vi "S4ICS.vi"() -> ()   [LabVIEW 2018]
uses:
  <vilib>/picture/picture.llb/imagedata.ctl
  MotorSim/MotorSim.lvclass
  StateManager/StateManager.lvclass
  Motor/Motor.lvclass
  StateManager/StateManager.lvclass/StateManager.ctl
  Messenger/Messenger.lvclass
  Motor/Motor.lvclass/Motor.ctl
  ICS/ICS.lvclass/ICS.ctl
  TCP-Server/TCP-Server.lvclass/TCP-Server.ctl
  Message Queue/Message Cluster.ctl
  ICS/Global Test.vi
  TCP-Server/TCP-Server.lvclass
  ICS/ICS.lvclass
  Message Queue/Message Queue.lvlib
  MotorManager/MotorManager.lvclass
panel:
  out "version":string caption="vers."
  out "tab body":enum32{"Motors", "Config"}(tab)
  out "commCALW":bool
  out "commGMIR":bool
  out "commASEL":bool
  out "commWPROT":bool
  out "commWPSEL":bool
  out "commGFOC":bool
  out "GFOC home":bool caption="Home"
  out "GFOC limit":bool caption="Limit"
  out "guider cam anime":picture
  out "gmir stat":T1
  out "ASEL Value":dbl
  out "CALW Value":dbl
  out "WPSEL Value":dbl
  out "GMIR Value":dbl
  out "WPROT Value":dbl
  out "GFOC Value":dbl
  out "calw stat":T1
  out "asel stat":T1
  out "wpsel stat":T1
  out "wprot stat":T1
  out "gfoc stat":T1
  out "asel lim on":bool caption="Limit ON"
  out "asel sec ON":bool caption="Sec. ON"
  out "asel lim off":bool caption="Limit OFF"
  out "asel sec off":bool caption="Sec. OFF"
  out "asel anime":picture
  out "asel background":picture
  out "wpsel sec/2":bool caption="Sec. L/4"
  out "wpsel sec/4":bool caption="Sec. L/2"
  out "wp home":bool caption="Home"
  out "wprot ctl":dbl(knob) scale=0.0..360.0
  out "wpsel lim/2":bool caption="Limit L/4"
  out "wpsel lim/4":bool caption="Limit L/2"
  out "wpsel anime":picture
  out "calw2":bool caption="CW 2"
  out "calw1":bool caption="CW 1"
  out "calw0":bool caption="CW 0"
  out "calw knob":cluster{dbl, dbl, dbl, dbl, dbl}(knob)={10.0, 82.0, 154.0, 226.0, 298.0} scale=0.0..360.0
  out "GMIR home":bool caption="Home"
  out "gmir knob":dbl(knob) scale=0.0..360.0
  out "asel image":T2
  in  "tips":T3(array[cluster])=[{"tip name"="login: server off", "PT"="Estado do servidor TCP/IP do S4ICS\npara clientes da rede (e.g. S4GUI).", "EN"="State of the S4ICS TCP/IP server\nfor network clients (e.g. S4GUI)."}, {"tip name"="login: exit", "PT"="Encerra a execução do programa\nS4ICS.", "EN"="Ends the execution of the S4ICS\nprogram."}, {"tip name"="login: language", "PT"="Seleciona a linguagem dos textos\nde ajuda e das dicas ou as ocultam.", "EN"="Select the language of the texts\nof help and tips or hide them."}, {"tip name"="login: user", "PT"="Nome cadastrado do usuário para\npermitir sua identificação.", "EN"="User's registered name to allow\nidentification."}, {"tip name"="login: password", "PT"="Senha cadastrada do usuário\n(digitada no 1o. acesso do usuário).", "EN"="User's registered password\n(entered on user's first login)."}, {"tip name"="login: help", "PT"="Descreve a função dos elementos\nmostrados no painel do S4ICS.", "EN"="Describes the function of elements\nshown on the S4ICS panel."}, {"tip name"="login: login", "PT"="Acesso ao S4ICS com a permissão\nestabelecida pelo administrador.", "EN"="Access to S4ICS according to\npermission set by administrator."}, {"tip name"="stopped: start srv", "PT"="Habilita o servidor TCP/IP do S4ICS\n(faz logout automaticamente).", "EN"="Enables S4ICS TCP/IP server\n(automatically logs out)."}, {"tip name"="stopped: exit", "PT"="Fecha o programa S4ICS.", "EN"="Ends S4ICS program execution."}, {"tip name"="stopped: assist", "PT"="Abre janela para testar e estacionar\nos mecanismos do instrumento.", "EN"="Opens window to test and park\ninstrument mechanisms."}, {"tip name"="stopped: setup", "PT"="Abre a janela de configuração do\ninstrumento (acesso restrito). ", "EN"="Opens the window of instrument\nconfiguration (restricted access)."}, {"tip name"="stopped: control", "PT"="Abre a janela para controlar os\nmecanismos (acesso restrito).", "EN"="Opens the window to control the\nmechanisms (restricted access)."}, {"tip name"="stopped: logout", "PT"="Libera o S4ICS para outro usuário.", "EN"="Release S4ICS for another user."}, {"tip name"="running: stop", "PT"="Desabilita o servidor\nTCP/IP doS4ICS.", "EN"="Disables S4ICS TCP/IP server."}, {"tip name"="running: logout", "PT"="Libera o S4ICS para outro usuário.", "EN"="Release S4ICS for another user."}, {"tip name"="setup: save", "PT"="Salva as alterações mantendo o\nnome do arquivo de  configuração.", "EN"="Save the changes keeping the\nname of the configuration file."}, {"tip name"="setup: save as", "PT"="Salva as alterações em um arquivo\nde  configuração com outro nome.", "EN"="Save changes to a file\nunder another name."}, {"tip name"="setup: help", "PT"="Descreve a função dos elementos\nmostrados no painel abaixo.", "EN"="Describes the function of elements\nshown on below panel."}, {"tip name"="setup: cfg file", "PT"="Nome do arquivo da\nconfiguração atual.\n", "EN"="File name of current configuration."}, {"tip name"="setup: cfg user", "PT"="Nome do usuário que salvou\na configuração atual.", "EN"="Username who saved\nthe current configuration."}, {"tip name"="setup: cfg date", "PT"="Data da configuração atual.", "EN"="Date of current configuration."}, {"tip name"="setup: return", "PT"="Retorna ao menu anterior.", "EN"="Return to previous menu."}, {"tip name"="assist: return", "PT"="Retorna ao menu anterior.", "EN"="Return to previous menu."}, {"tip name"="control: return", "PT"="Retorna ao menu anterior.", "EN"="Return to previous menu."}, {"tip name"="cfg: previous", "PT"="Mostra e seleciona\no usuário anterior.", "EN"="Show and select\nprevious user."}, {"tip name"="cfg: next", "PT"="Mostra e seleciona\no próximo usuário.", "EN"="Show and select\nthe next user."}, {"tip name"="cfg: delete", "PT"="Remove da lista o\nusuário selecionado.", "EN"="Remove from the list\nthe selected user."}, {"tip name"="cfg: name", "PT"="Nome do novo usuário\npara ser inserido na lista.", "EN"="New user name to be\ninserted into the list."}, {"tip name"="cfg: insert", "PT"="Insere na lista o novo usuário com\no nome e a permissão indicados.", "EN"="Insert the new user with the\ngiven name and permission."}, {"tip name"="cfg: permission", "PT"="Permissão do usuário. Restringir\nas atribuições Admin e Control.", "EN"="User permission. Restrict the\nAdmin and Control assignments."}, {"tip name"="cfg: change", "PT"="Atribui a atribuição ao lado\npara o usuário selecionado.", "EN"="Assign left assignment\nfor the selected user."}, {"tip name"="cfg: auto", "PT"="Tempo limite de inatividade para\nlogout automático do usuário.", "EN"="Inactivity timeout to\nautomatic user logout."}, {"tip name"="cfg: enable", "PT"="Permite o envio de e-mails\nde manutenção e configuração.", "EN"="Allows sending maintenance\nand configuration emails."}, {"tip name"="cfg: service", "PT"="Endereço IP e porta do\nservidor de e-mail.", "EN"="IP address and port\nof email server."}, {"tip name"="cfg: admin", "PT"="Endereço de e-mail que receberá\nnotificações de nova configuração.", "EN"="Email address that will receive\nnew configuration notifications."}, {"tip name"="cfg: maint", "PT"="Endereço de email que irá receber\nnotificações de erro e alarme.", "EN"="Email address that will receive\nerror and alarm notifications."}, {"tip name"="cfg: check", "PT"="Envia e-mail e confere recebimento\npara testar o servidor de e-mail.", "EN"="Send emails and check receipt\nto test the email server."}, {"tip name"="cfg: ok", "PT"="Resultado do teste do servidor de\ne-mail. Aguarde alguns segundos.", "EN"="Test result from email server test.\nPlease, wait a few seconds."}, {"tip name"="cfg: srv ip", "PT"="Endereço IP do servidor do S4ICS:\nlocalhost ou IP local (ver abaixo).", "EN"="S4ICS server IP address:\nlocalhost or local IP (see below)."}, {"tip name"="cfg: srv port", "PT"="Porta do servidor do S4ICS que\nserá usada pelos clientes (S4GUI).", "EN"="S4ICS server port used\nby clients (like S4GUI)."}, {"tip name"="cfg: srv timeout", "PT"="Tempo de espera pela conexão:\nmenor tempo exigido pelo servidor do S4ICS.", "EN"="Connection wait time: lower time\nrequired by S4ICS server."}, {"tip name"="cfg: IP1", "PT"="Porta IP ativa (com conexão)\nneste computador.", "EN"="Active IP port (with connection)\non this computer."}, {"tip name"="cfg: IP2", "PT"="Porta IP ativa (com conexão)\nneste computador.", "EN"="Active IP port (with connection)\non this computer."}]
  in  "Enddelay":u32=25
  in  "TX-RXdelay":u32=25
  in  "pubTime0mq":i32=1000 caption="Pub Time*"
  in  "0mqEndpoint":string="5565" caption="PUB Port*"
  in  "address":string="192.168.1.170" caption="Address"
  in  "runMinimized":bool
  in  "autoSS":bool
  in  "log help":bool
  in  "enabled log":string="0123456" caption="LOG Enable"
  in  "WPSEL mode":string(combo)="Control" caption="Mechanism Mode"
  in  "CALW mode":string(combo)="Control" caption="Mechanism Mode"
  in  "GFOC mode":string(combo)="Control" caption="Mechanism Mode"
  in  "animation":bool
  in  "full init":bool
  in  "timeout":i32=100 caption="Timeout"
  in  "port":u16=5564 caption="Port"
  in  "pwrPM mains":bool=TRUE caption="Mains"
  in  "pwrPM password":string="ubnt" caption="Password"
  in  "pwrPM user":string="ubnt" caption="User"
  in  "pwrPM outlet":u16=5 caption="Outlet"
  in  "pwrPM port":u16=6080 caption="Port"
  in  "pwrPM ip":string="192.168.1.20" caption="IP"
  in  "pwrGD mains":bool=TRUE caption="Mains"
  in  "pwrGD password":string="ubnt" caption="Password"
  in  "pwrGD user":string="ubnt" caption="User"
  in  "pwrGD outlet":u16=6 caption="Outlet"
  in  "pwrGD port":u16=6080 caption="Port"
  in  "pwrGD ip":string="192.168.1.20" caption="IP"
  in  "GMIR disabled":bool
  in  "GMIR mode":string(combo)="Control" caption="Mechanism Mode"
  in  "GMIR ip":string="192.168.1.249" caption="ip"
  in  "GFOC positions":cluster{"pos_name":string, "pos_value":dbl}[](array[cluster])=[{"pos_name"="OFFSET", "pos_value"=0.0}] caption="GFOC" {"pos_value" min=-400.0 max=400.0 step=0.1}
  in  "GMIR positions":cluster{"pos_name":string, "pos_value":dbl}[](array[cluster])=[{"pos_name"="OFFSET", "pos_value"=0.0}] caption="GMIR" {"pos_value" min=-10.0 max=110.0 step=0.1}
  in  "WPSEL disabled":bool
  in  "WPROT disabled":bool
  in  "WPSEL ip":string="192.168.1.246" caption="ip"
  in  "WPROT mode":string(combo)="Control" caption="Mechanism Mode"
  in  "WPROT ip":string="192.168.1.245" caption="ip"
  in  "WPSEL positions":cluster{"pos_name":string, "pos_value":dbl}[](array[cluster])=[{"pos_name"="OFFSET", "pos_value"=0.0}, {"pos_name"="L/4", "pos_value"=0.0}, {"pos_name"="OFF", "pos_value"=400000.0}, {"pos_name"="L/2", "pos_value"=800000.0}] caption="WPSEL" {"pos_value" min=-400.0 max=400.0 step=0.1}
  in  "WPROT positions":cluster{"pos_name":string, "pos_value":dbl}[](array[cluster])=[{"pos_name"="OFFSET", "pos_value"=0.0}, {"pos_name"="WP1", "pos_value"=0.0}, {"pos_name"="WP2", "pos_value"=1875.0}, {"pos_name"="WP3", "pos_value"=3750.0}, {"pos_name"="WP4", "pos_value"=5625.0}, {"pos_name"="WP5", "pos_value"=7500.0}, {"pos_name"="WP6", "pos_value"=9375.0}, {"pos_name"="WP7", "pos_value"=11250.0}, {"pos_name"="WP8", "pos_value"=13125.0}, {"pos_name"="WP9", "pos_value"=15000.0}, {"pos_name"="WP10", "pos_value"=16875.0}, {"pos_name"="WP11", "pos_value"=18750.0}, {"pos_name"="WP12", "pos_value"=20625.0}, {"pos_name"="WP13", "pos_value"=22500.0}, {"pos_name"="WP14", "pos_value"=24375.0}, {"pos_name"="WP15", "pos_value"=26250.0}, {"pos_name"="WP16", "pos_value"=28125.0}] caption="WPROT" {"pos_value" min=-10.0 max=110.0 step=0.1}
  in  "CALW disabled":bool
  in  "ASEL disabled":bool
  in  "CALW ip":string="192.168.1.247" caption="ip"
  in  "ASEL mode":string(combo)="Control" caption="Mechanism Mode"
  in  "ASEL ip":string="192.168.1.248" caption="ip"
  in  "CALW positions":cluster{"pos_name":string, "pos_value":dbl}[](array[cluster])=[{"pos_name"="OFFSET", "pos_value"=0.0}, {"pos_name"="OFF", "pos_value"=0.0}, {"pos_name"="POLARIZER", "pos_value"=12000.0}, {"pos_name"="PINHOLE", "pos_value"=24000.0}, {"pos_name"="SHUTTER", "pos_value"=36000.0}, {"pos_name"="DEPOLARIZER", "pos_value"=48000.0}] caption="CALW" {"pos_value" min=-400.0 max=400.0 step=0.1}
  in  "ASEL positions":cluster{"pos_name":string, "pos_value":dbl}[](array[cluster])=[{"pos_name"="OFFSET", "pos_value"=0.0}, {"pos_name"="OFF", "pos_value"=0.0}, {"pos_name"="ON", "pos_value"=4800.0}] caption="ASEL" {"pos_value" min=-10.0 max=110.0 step=0.1}
  in  "S4ICS password":string="se4RFVgy&8"
  in  "S4ICS login":string="s4ics@lna.br"
  in  "S4ICS email":string="s4ics@lna.br" caption="S4ICS account"
  in  "auto logout":u32=200 caption="Auto Logout period" min=30 max=3000
  out "email ok":bool
  in  "check email":bool
  in  "maint. email":string="frodrigues@lna.br" caption="Maintenance"
  in  "admin email":string="nivaldo@lna.br" caption="Configuration"
  in  "email service":string="smtp.gmail.com:587" caption="Server IP:PORT"
  out "user list":T4(array[cluster]) caption="Name                 Permission        PW"
  in  "user delete":bool
  in  "user permission":string(combo)="Start / Stop" caption="Permission"
  in  "change permission":bool
  in  "user insert":bool
  in  "user name":string caption="New User"
  in  "user previous":bool
  in  "user next":bool
  in  "email enable":bool caption="Email service"
  in  "channel":T5(ring)=enum."Inner TCP/IP" caption="Channel"
  out "local IP 1":string
  out "local IP 2":string
  in  "comm help":bool
  out "tab menu":T6(tab)
  in  "login help":bool
  in  "loginPW":string caption="Password"
  in  "loginUser":string caption="User Name"
  in  "login":bool
  out "server":bool
  in  "exitLogin":bool
  in  "language":enum32{"PT", "EN", "NONE"}(radio)=enum."NONE"
  in  "stop server":bool
  in  "logout running":bool
  in  "exitStopped":bool
  in  "logout stopped":bool
  in  "start server":bool
  in  "control":bool
  in  "setup":bool
  in  "assist":bool
  in  "return assist":bool
  in  "save as":bool
  out "last cfg date":string caption="Date"
  out "last cfg user":string caption="User"
  in  "save config":bool
  in  "return setup":bool
  in  "config help":bool
  out "cfgFile":string caption="CONFIG FILE"
  out "control response":string caption="Response"
  in  "control instruction":string caption="Instruction"
  in  "control send":bool
  in  "control jump":bool caption="JUMP"
  in  "control position":dbl caption="Mech. Position"
  in  "return control":bool
  in  "control stop":bool
  in  "control motor sel":T7(radio) caption="Motor"
  # "GFOC - Guiding Focuser"
  # "GMIR - Guiding Mirror"
  # "CALW - Calibration Wheel"
  # "FOCUSER"
  # "CLEAR"
  # "GUIDING"
  # "CAMERA"
  # "POLARIZER"
  # "PINHOLE"
  # "SHUTTER"
  # "PATROL"
  # "MIRROR"
  # "DEPOLARIZER"
  # "WPROT - Waveplate Rotator"
  # "WPSEL - Waveplate Selector"
  # "ASEL - Analyser Selector"
  # "POLARIMETRIC MECHANISMS"
  # "SERVER COMMUNICATION"
  # "USER LIST"
  # "(*) Requires EXIT after SAVE\n      Exigido EXIT depois de SAVE"
  # "SIMULATION"
  # "ANIMATION"
  # "ON"
  # "FAST"
  # "FULL"
  # "OFF"
  # "s"
  # "EMAIL SETTINGS"
  # "GUIDING MECHANISMS"
  # "POWER"
  # "POWER"
  # "GMIR & GFOC"
  # "GFOC motor is driven by the GMIR cotroller."
  # "IDENTIFICATION"
  # "LAST CONFIGURATION"
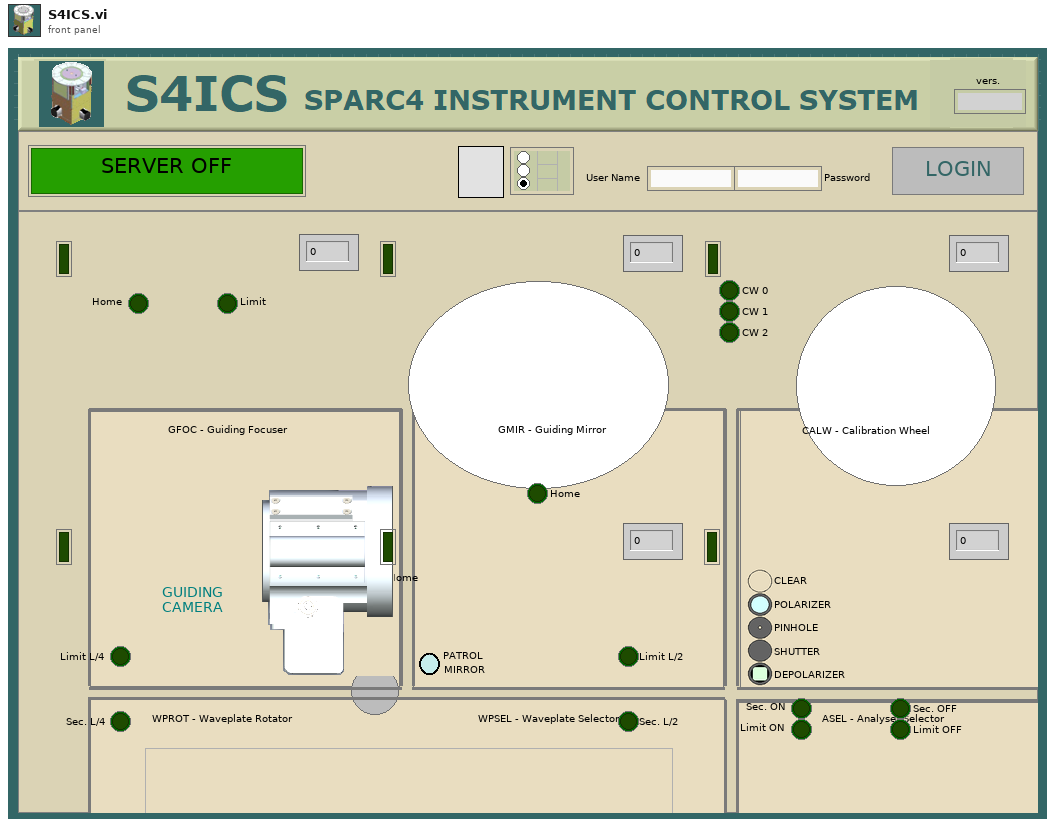
[diagram p1: front panel]
types:
  T1 = cluster{"mode":string, "condition":string, "position":string, "pos_name":string, "pos_id":string}
  T2 = typedef "imagedata.ctl" = cluster{"image type":i32, "image depth":i32, "image":u8[], "mask":u8[], "colors":u32[], "Rectangle":cluster{"left":i16, "top":i16, "right":i16, "bottom":i16}}
  T3 = cluster{"tip name":string, "PT":string, "EN":string}[]
  T4 = cluster{"name":string, "permission":string, "password":string}[]
  T5 = enum32{"Local Panel", "Inner TCP/IP", "Outer TCP/IP", "MQTT", "ZeroMQ"}
  T6 = enum32{"Login", "Running", "Stopped", "Assist", "Setup", "Control"}
  T7 = enum32{"No Selection", "control WPROT", "control WPSEL", "control ASEL", "control CALW", "control GFOC", "control GMIR"}
  T8 = cluster{"S4commandQueueName":string, "S4statusQueueName":string, "comm configuration":cluster{"channel":enum32{"Local Panel", "Inner TCP/IP", "Outer TCP/IP", "MQTT", "ZeroMQ"}, "address":string, "port":u16, "timeout":i32}}
  T9 = enum32{"Motors", "Config", "Status", "Anime", "Param"}
  T10 = cluster{"email service":string, "maint. email":string, "admin email":string, "S4ICS email":string, "S4ICS login":string, "S4ICS password":string, "email enabled":bool}
  T11 = cluster{"period":u32, "initial position (0)":i32, "translation (100)":i32, "forward":bool}[]
  T12 = enum8{"Enabled", "Disabled", "Disabled and Grayed Out"}
  T13 = enum32{"Invalid", "Standard", "Closed", "Hidden", "Minimized", "Maximized"}
  T14 = cluster{"left":i16, "top":i16, "right":i16, "bottom":i16}
  T15 = enum32{"Login", "Stopped", "Running", "Setup", "Assist", "Control"}
  T16 = enum16{"Wait", "ActiveInit", "ActiveGoto", "ActiveUpdate", "ActiveStop", "ActiveFinish", "SimInit", "SimGoto", "SimUptate", "SimFinish", "CyclicStart", "CyclicUpdate", "CyclicFinish"}
  T17 = cluster{"action":string, "param":string, "pos_name":string, "pos_idx":i32, "ack":bool, "stop":bool, "offset":bool, "immediate":bool, "instructions":string[]}
  T18 = typedef "Message Queue.lvlib/Message Cluster.ctl" = cluster{"Message":string, "Message Data":variant}
  T19 = cluster{"channel":enum32{"Local Panel", "Inner TCP/IP", "Outer TCP/IP", "MQTT", "ZeroMQ"}, "address":string, "port":u16, "timeout":i32}
  T20 = cluster{"name":string, "permission":string, "password":string}
  T21 = cluster{"[0]":dbl, "[1]":dbl, "[2]":dbl, "[3]":dbl, "[4]":dbl}
  T22 = enum32{"invalid app kind", "Development System", "Run Time System", "Student Edition", "Embedded LabVIEW", "Evaluation", "Custom"}
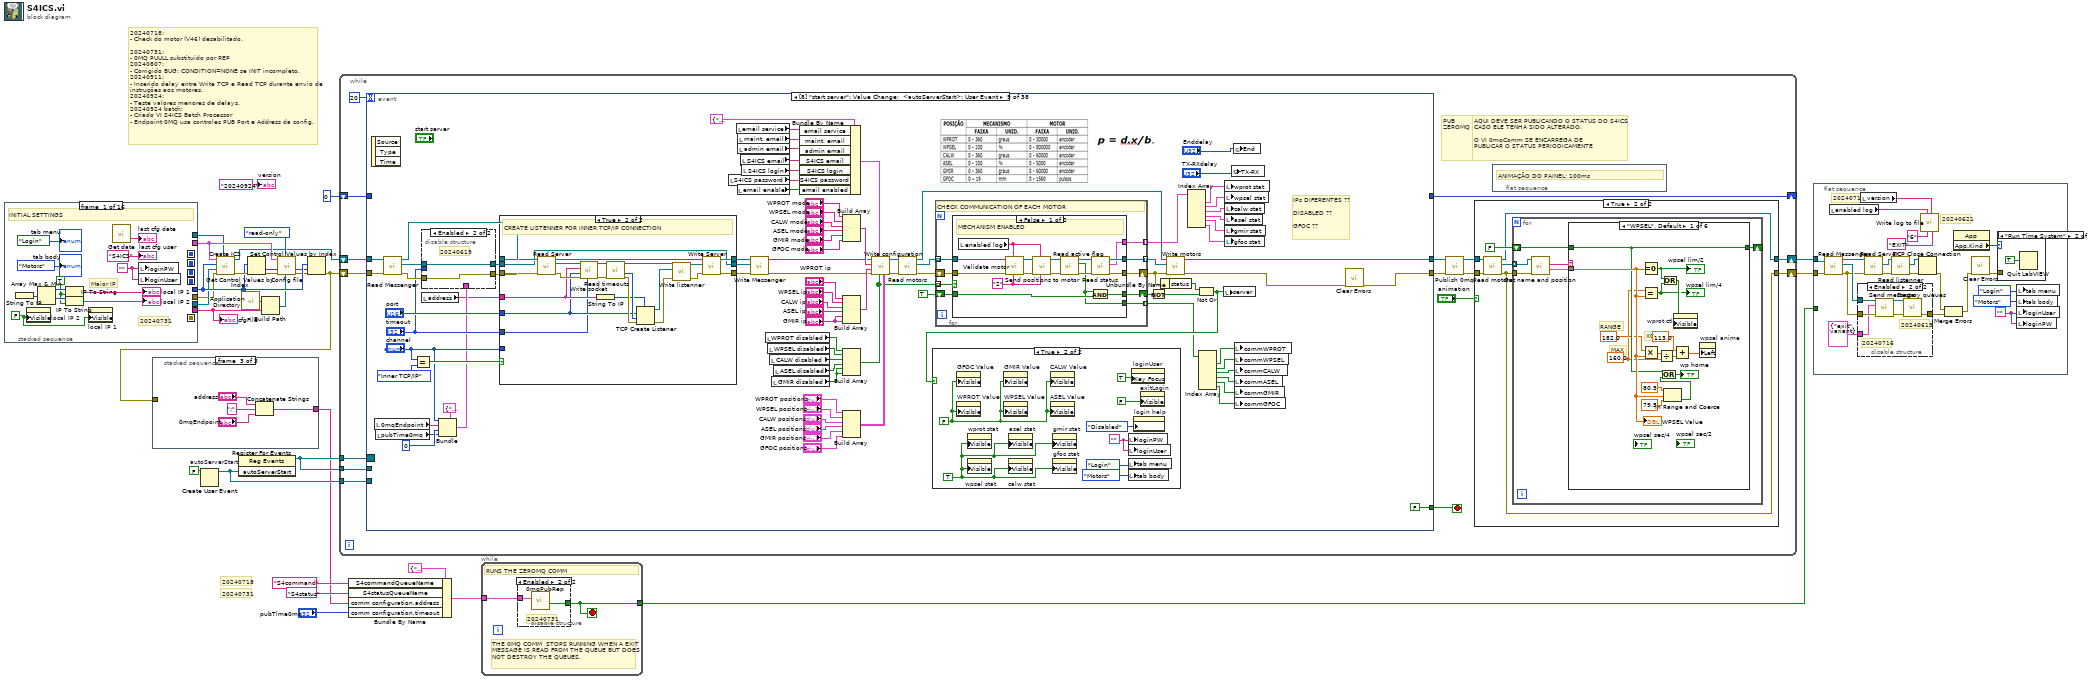
[diagram p0: block diagram]
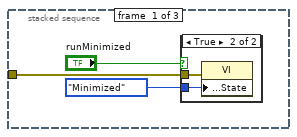
[diagram p2: hidden frame]
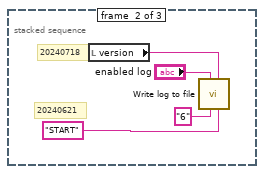
[diagram p4: hidden frame]
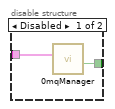
[diagram p5: hidden frame]
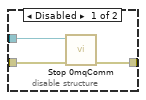
[diagram p6: hidden frame]
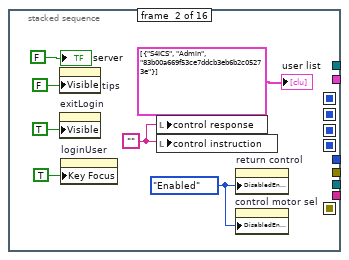
[diagram p8: hidden frame]
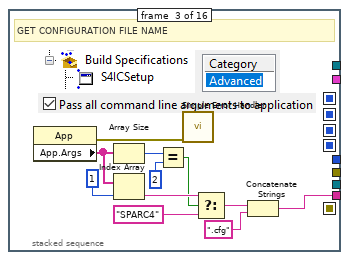
[diagram p9: hidden frame]
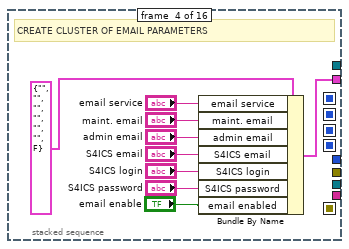
[diagram p10: hidden frame]
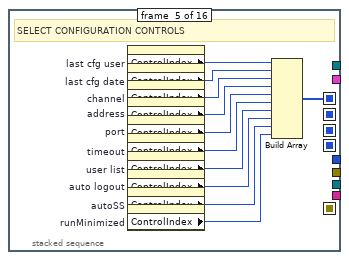
[diagram p11: hidden frame]
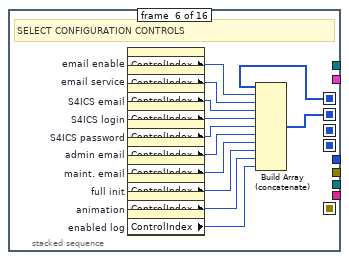
[diagram p12: hidden frame]
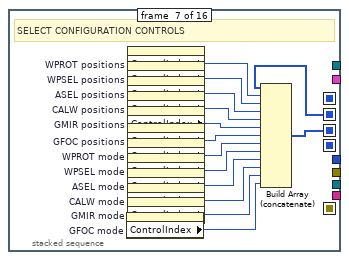
[diagram p13: hidden frame]
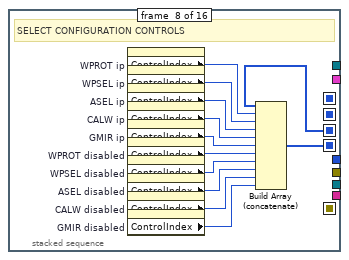
[diagram p14: hidden frame]
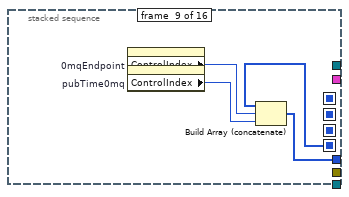
[diagram p15: hidden frame]
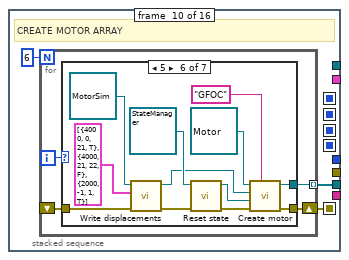
[diagram p16: hidden frame]
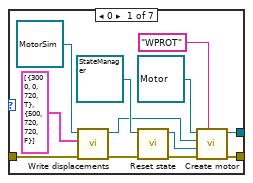
[diagram p17: hidden frame]
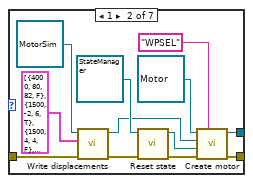
[diagram p18: hidden frame]
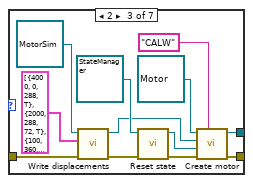
[diagram p19: hidden frame]
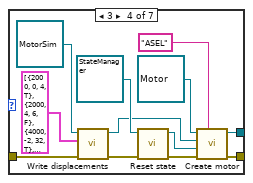
[diagram p20: hidden frame]
diagram:
  w12 = FALSE  # autoServerStart
  # "20240731"
  # "20240718"
  # "20240718:\n- Check do motor (V46) desabilitado.\n\n20240731:\n- 0MQ PUULL substituído por REP\n20240807:\n- Corrigido BUG: CONDITION=NONE se INIT incompleto.\n20240911:\n- Inserido delay entre Write TCP e Read TCP durante envio de instruções aos motores.\n20240924:\n- Teste valores menores de delays.\n20240924 batch:\n- Criado VI S4ICS Batch Processor\n- Endpoint 0MQ usa controles PUB Port e Address da config."
  n1 = stacked-sequence {
    seq-local: [_ _ _ _ w78 _ _ _ _ _ _ _ _ _ _ _] -> [_ _ _ _ _ w92 _ _ _ _ _ _ _ _ _ _]
    seq-local: [_ _ _ _ _ w84 _ _ _ _ _ _ _ _ _ _] -> [_ _ _ _ _ _ w99 _ _ _ _ _ _ _ _ _]
    seq-local: [_ _ _ _ _ _ w98 _ _ _ _ _ _ _ _ _] -> [_ _ _ _ _ _ _ w118 _ _ _ _ _ _ _ _]
    seq-local: [_ _ _ _ _ _ _ _ _ w124 _ _ _ _ _ _] -> [_ _ _ _ _ _ _ _ _ _ _ _ _ _ w240 _]
    seq-local: [_ _ _ _ _ _ _ w107 _ _ _ _ _ _ _ _] -> [_ _ _ _ _ _ _ _ w122 _ _ _ _ _ _ _]
    tunnel: [_ _ w58 _ _ _ _ _ _ _ _ _ _ _ _ _] -> w27
    tunnel: [_ _ _ w61 _ _ _ _ _ _ _ _ _ _ _ _] -> w24
    tunnel: [_ _ _ _ _ _ _ _ w121 _ _ _ _ _ _ _] -> w26
    tunnel: [_ _ _ _ _ _ _ _ _ w125 _ _ _ _ _ _] -> w25
    tunnel: [_ _ _ _ _ _ _ _ _ _ _ _ _ _ w235 _] -> w15
    tunnel: [_ _ _ _ _ _ _ _ _ _ _ _ _ _ w234 _] -> w14
    frame #0 {
      w33 = FALSE
      w37 = TRUE
      w34 = ""
      # "20240731"
      # "Maior IP"
      # "INITIAL SETTINGS"
      n2 = String To IP() -> (0:w40:u32[])  [unwired: 1 in]
      n3 = property on="local IP 2" class="Str"("Visible"=w33) -> ()  [unwired: 2 in, 2 out]
      n4 = Array Max & Min(array=w40) -> (max value=w39:u32, min value=w38:u32)  [unwired: 2 out]
      n5 = IP To String(1:w37, 2:w39) -> (0:→"local IP 1":string)
      n6 = IP To String(1:w37, 2:w38) -> (0:→"local IP 2":string)
      n7 = property on="local IP 1" class="Str"("Visible"=w33) -> ()  [unwired: 2 in, 2 out]
      n8 = call "Get date.vi"() -> ("date/time string"=→"last cfg date":string)  [unwired: 3 in]
      n9 = local write "loginPW"(w34) -> ()
      n10 = local write "loginUser"(w34) -> ()
      "last cfg user" <- "S4ICS" ("last user")
      "tab menu" <- T6."Login" ("tab menu")
      "tab body" <- T9."Motors" ("tab body")
    }
    frame #1 {
      w43 = ""
      w44 = T12."Enabled" ("Disabled")
      n11 = property on="tips" class="Arr (strict)"("Visible"=FALSE) -> ()  [unwired: 2 in, 2 out]
      n12 = property on="exitLogin" class="Bool"("Visible"=TRUE) -> ()  [unwired: 2 in, 2 out]
      n13 = property on="loginUser" class="Str"("Key Focus"=TRUE) -> ()  [unwired: 2 in, 2 out]
      n14 = local write "control response"(w43) -> ()
      n15 = local write "control instruction"(w43) -> ()
      n16 = property on="return control" class="Bool"("DisabledEnum"=w44) -> ()  [unwired: 2 in, 2 out]
      n17 = property on="control motor sel" class="RadioBtnsControl (strict)"("DisabledEnum"=w44) -> ()  [unwired: 2 in, 2 out]
      "server" <- FALSE
      "user list" <- T4 [{"name"="S4ICS", "permission"="Admin", "password"="83b00a669f53ce7ddcb3eb6b2c05273e"}] ("users")
    }
    frame #2 {
      # "GET CONFIGURATION FILE NAME"
      n18 = property class="App"() -> (error out=w59:errorcluster, "App.Args"=w55:string[])  [unwired: 2 in, 1 out]
      n19 = Array Size(array=w55) -> (size(s)=w57:i32)
      n20 = Index Array(array=w55, index=1) -> (element=w54:string)
      n21 = Equal?(x=w57, y=2 ("x")) -> (x = y?=w50:bool)
      n22 = call <vilib>:"Simple Error Handler.vi"("error in (no error)"=w59) -> ()  [unwired: 4 in, 5 out]
      n23 = Select(t=w54, s=w50, f="SPARC4" ("string")) -> (s? t:f=w52:string)
      n24 = Concatenate Strings(w52, ".cfg" ("string")) -> (w58:string)
    }
    frame #3 {
      # "CREATE CLUSTER OF EMAIL PARAMETERS"
      n25 = Bundle By Name(cluster=T10 {"email service"="", "maint. email"="", "admin email"="", "S4ICS email"="", "S4ICS login"="", "S4ICS password"="", "email enabled"=FALSE} ("email cluster"), "email service"="email service", "maint. email"="maint. email", "admin email"="admin email", "S4ICS email"="S4ICS email", "S4ICS login"="S4ICS login", "S4ICS password"="S4ICS password", "email enabled"="email enable") -> (w61:T10)
    }
    frame #4 {
      # "SELECT CONFIGURATION CONTROLS"
      n26 = property on="last cfg user" class="Str"() -> ("ControlIndex"=w79:i32)  [unwired: 2 in, 2 out]
      n27 = property on="last cfg date" class="Str"() -> ("ControlIndex"=w80:i32)  [unwired: 2 in, 2 out]
      n28 = property on="channel" class="Enum (strict)"() -> ("ControlIndex"=w72:i32)  [unwired: 2 in, 2 out]
      n29 = property on="address" class="Str"() -> ("ControlIndex"=w73:i32)  [unwired: 2 in, 2 out]
      n30 = property on="port" class="DigNum (strict)"() -> ("ControlIndex"=w74:i32)  [unwired: 2 in, 2 out]
      n31 = property on="timeout" class="DigNum (strict)"() -> ("ControlIndex"=w75:i32)  [unwired: 2 in, 2 out]
      n32 = property on="user list" class="Arr (strict)"() -> ("ControlIndex"=w76:i32)  [unwired: 2 in, 2 out]
      n33 = property on="auto logout" class="DigNum (strict)"() -> ("ControlIndex"=w77:i32)  [unwired: 2 in, 2 out]
      n34 = property on="autoSS" class="Bool (strict)"() -> ("ControlIndex"=w71:i32)  [unwired: 2 in, 2 out]
      n35 = property on="runMinimized" class="Bool (strict)"() -> ("ControlIndex"=w70:i32)  [unwired: 2 in, 2 out]
      n36 = Build Array(w79, w80, w72, w73, w74, w75, w76, w77, w71, w70) -> (w78:i32[])
    }
    frame #5 {
      # "SELECT CONFIGURATION CONTROLS"
      n37 = property on="email enable" class="Bool (strict)"() -> ("ControlIndex"=w88:i32)  [unwired: 2 in, 2 out]
      n38 = property on="email service" class="Str"() -> ("ControlIndex"=w89:i32)  [unwired: 2 in, 2 out]
      n39 = property on="S4ICS email" class="Str"() -> ("ControlIndex"=w90:i32)  [unwired: 2 in, 2 out]
      n40 = property on="S4ICS login" class="Str"() -> ("ControlIndex"=w91:i32)  [unwired: 2 in, 2 out]
      n41 = property on="S4ICS password" class="Str"() -> ("ControlIndex"=w87:i32)  [unwired: 2 in, 2 out]
      n42 = property on="admin email" class="Str"() -> ("ControlIndex"=w86:i32)  [unwired: 2 in, 2 out]
      n43 = property on="maint. email" class="Str"() -> ("ControlIndex"=w85:i32)  [unwired: 2 in, 2 out]
      n44 = property on="full init" class="Bool (strict)"() -> ("ControlIndex"=w83:i32)  [unwired: 2 in, 2 out]
      n45 = property on="animation" class="Bool (strict)"() -> ("ControlIndex"=w82:i32)  [unwired: 2 in, 2 out]
      n46 = property on="enabled log" class="Str"() -> ("ControlIndex"=w81:i32)  [unwired: 2 in, 2 out]
      n47 = Build Array (concatenate)(w92, w88, w89, w90, w91, w87, w86, w85, w83, w82, w81) -> (w84:i32[])
    }
    frame #6 {
      # "SELECT CONFIGURATION CONTROLS"
      n48 = property on="GFOC mode" class="CmbBox"() -> ("ControlIndex"=w97:i32)  [unwired: 2 in, 2 out]
      n49 = property on="WPROT positions" class="Arr (strict)"() -> ("ControlIndex"=w102:i32)  [unwired: 2 in, 2 out]
      n50 = property on="WPSEL positions" class="Arr (strict)"() -> ("ControlIndex"=w103:i32)  [unwired: 2 in, 2 out]
      n51 = property on="ASEL positions" class="Arr (strict)"() -> ("ControlIndex"=w104:i32)  [unwired: 2 in, 2 out]
      n52 = property on="CALW positions" class="Arr (strict)"() -> ("ControlIndex"=w105:i32)  [unwired: 2 in, 2 out]
      n53 = property on="GMIR positions" class="Arr (strict)"() -> ("ControlIndex"=w106:i32)  [unwired: 2 in, 2 out]
      n54 = property on="GFOC positions" class="Arr (strict)"() -> ("ControlIndex"=w101:i32)  [unwired: 2 in, 2 out]
      n55 = property on="WPROT mode" class="CmbBox"() -> ("ControlIndex"=w100:i32)  [unwired: 2 in, 2 out]
      n56 = property on="WPSEL mode" class="CmbBox"() -> ("ControlIndex"=w93:i32)  [unwired: 2 in, 2 out]
      n57 = property on="ASEL mode" class="CmbBox"() -> ("ControlIndex"=w94:i32)  [unwired: 2 in, 2 out]
      n58 = property on="CALW mode" class="CmbBox"() -> ("ControlIndex"=w95:i32)  [unwired: 2 in, 2 out]
      n59 = property on="GMIR mode" class="CmbBox"() -> ("ControlIndex"=w96:i32)  [unwired: 2 in, 2 out]
      n60 = Build Array (concatenate)(w99, w102, w103, w104, w105, w106, w101, w100, w93, w94, w95, w96, w97) -> (w98:i32[])
    }
    frame #7 {
      # "SELECT CONFIGURATION CONTROLS"
      n61 = property on="WPROT ip" class="Str"() -> ("ControlIndex"=w117:i32)  [unwired: 2 in, 2 out]
      n62 = property on="WPSEL ip" class="Str"() -> ("ControlIndex"=w116:i32)  [unwired: 2 in, 2 out]
      n63 = property on="ASEL ip" class="Str"() -> ("ControlIndex"=w115:i32)  [unwired: 2 in, 2 out]
      n64 = property on="CALW ip" class="Str"() -> ("ControlIndex"=w114:i32)  [unwired: 2 in, 2 out]
      n65 = property on="GMIR ip" class="Str"() -> ("ControlIndex"=w113:i32)  [unwired: 2 in, 2 out]
      n66 = property on="WPROT disabled" class="Bool (strict)"() -> ("ControlIndex"=w112:i32)  [unwired: 2 in, 2 out]
      n67 = property on="WPSEL disabled" class="Bool (strict)"() -> ("ControlIndex"=w111:i32)  [unwired: 2 in, 2 out]
      n68 = property on="ASEL disabled" class="Bool (strict)"() -> ("ControlIndex"=w110:i32)  [unwired: 2 in, 2 out]
      n69 = property on="CALW disabled" class="Bool (strict)"() -> ("ControlIndex"=w109:i32)  [unwired: 2 in, 2 out]
      n70 = property on="GMIR disabled" class="Bool (strict)"() -> ("ControlIndex"=w108:i32)  [unwired: 2 in, 2 out]
      n71 = Build Array (concatenate)(w118, w117, w116, w115, w114, w113, w112, w111, w110, w109, w108) -> (w107:i32[])
    }
    frame #8 {
      n72 = property on="0mqEndpoint" class="Str"() -> ("ControlIndex"=w120:i32)  [unwired: 2 in, 2 out]
      n73 = property on="pubTime0mq" class="DigNum (strict)"() -> ("ControlIndex"=w119:i32)  [unwired: 2 in, 2 out]
      n74 = Build Array (concatenate)(w122, w120, w119) -> (w121:i32[])
    }
    frame #9 {
      # "CREATE MOTOR ARRAY"
      n75 = for {
        N: 6 -> [_]
        shift-right: [w129] -> w124
        shift-left: _ -> [w128]
        tunnel: [w127] -> w125 mode=indexing
        i -> [w126]
        n76 = case shown="5" w126 {
          tunnel: [w141 w153 w165 w177 w189 w201 w202] -> w129
          tunnel: w128 -> [w140 w152 w164 w176 w188 w200 w202]
          tunnel: [w134 w146 w158 w170 w182 w194 _] -> w127
          frame 0 {
            n77 = call-dynamic "Write displacements.vi"("error in (no error)"=w140, "displacements"=T11 [{"period"=3000, "initial position (0)"=0, "translation (100)"=720, "forward"=TRUE}, {"period"=500, "initial position (0)"=720, "translation (100)"=720, "forward"=FALSE}] ("WPROT moves"), "MotorSim in"=refnum<class "MotorSim.lvclass"> refnum ("MotorSim.lvclass")) -> ("error out"=w135:errorcluster, "MotorSim out"=w132:refnum<class "MotorSim.lvclass">)  [unwired: 7 in]
            n78 = call "Reset state.vi"("error in (no error)"=w135, "StateManager in"=refnum<class "StateManager.lvclass"> refnum ("StateManager.lvclass")) -> ("error out"=w139:errorcluster, "StateManager out"=w133:refnum<class "StateManager.lvclass">)  [unwired: 8 in]
            n79 = call-dynamic "Create motor.vi"("name"="WPROT", "error in (no error)"=w139, "StateManager"=w133, "MotorSim"=w132, "Motor in"=refnum<class "Motor.lvclass"> refnum ("Motor.lvclass")) -> ("error out"=w141:errorcluster, "Motor out"=w134:refnum<class "Motor.lvclass">)  [unwired: 5 in]
          }
          frame 1 {
            n80 = call-dynamic "Write displacements.vi"("error in (no error)"=w152, "displacements"=T11 [{"period"=4000, "initial position (0)"=80, "translation (100)"=82, "forward"=FALSE}, {"period"=1500, "initial position (0)"=-2, "translation (100)"=6, "forward"=TRUE}, {"period"=1500, "initial position (0)"=4, "translation (100)"=4, "forward"=FALSE}, {"period"=6000, "initial position (0)"=0, "translation (100)"=80, "forward"=TRUE}, {"period"=6000, "initial position (0)"=80, "translation (100)"=82, "forward"=TRUE}, {"period"=2000, "initial position (0)"=162, "translation (100)"=6, "forward"=FALSE}, {"period"=2000, "initial position (0)"=156, "translation (100)"=156, "forward"=FALSE}] ("WPSEL moves"), "MotorSim in"=refnum<class "MotorSim.lvclass"> refnum ("MotorSim.lvclass")) -> ("error out"=w147:errorcluster, "MotorSim out"=w144:refnum<class "MotorSim.lvclass">)  [unwired: 7 in]
            n81 = call "Reset state.vi"("error in (no error)"=w147, "StateManager in"=refnum<class "StateManager.lvclass"> refnum ("StateManager.lvclass")) -> ("error out"=w151:errorcluster, "StateManager out"=w145:refnum<class "StateManager.lvclass">)  [unwired: 8 in]
            n82 = call-dynamic "Create motor.vi"("name"="WPSEL", "error in (no error)"=w151, "StateManager"=w145, "MotorSim"=w144, "Motor in"=refnum<class "Motor.lvclass"> refnum ("Motor.lvclass")) -> ("error out"=w153:errorcluster, "Motor out"=w146:refnum<class "Motor.lvclass">)  [unwired: 5 in]
          }
          frame 2 {
            n83 = call-dynamic "Write displacements.vi"("error in (no error)"=w164, "displacements"=T11 [{"period"=4000, "initial position (0)"=0, "translation (100)"=288, "forward"=TRUE}, {"period"=2000, "initial position (0)"=288, "translation (100)"=72, "forward"=TRUE}, {"period"=100, "initial position (0)"=360, "translation (100)"=360, "forward"=FALSE}, {"period"=1200, "initial position (0)"=0, "translation (100)"=72, "forward"=TRUE}, {"period"=1200, "initial position (0)"=72, "translation (100)"=72, "forward"=TRUE}, {"period"=1200, "initial position (0)"=144, "translation (100)"=72, "forward"=TRUE}, {"period"=1200, "initial position (0)"=216, "translation (100)"=72, "forward"=TRUE}, {"period"=1200, "initial position (0)"=288, "translation (100)"=72, "forward"=TRUE}, {"period"=100, "initial position (0)"=360, "translation (100)"=360, "forward"=FALSE}] ("CALW moves"), "MotorSim in"=refnum<class "MotorSim.lvclass"> refnum ("MotorSim.lvclass")) -> ("error out"=w159:errorcluster, "MotorSim out"=w156:refnum<class "MotorSim.lvclass">)  [unwired: 7 in]
            n84 = call "Reset state.vi"("error in (no error)"=w159, "StateManager in"=refnum<class "StateManager.lvclass"> refnum ("StateManager.lvclass")) -> ("error out"=w163:errorcluster, "StateManager out"=w157:refnum<class "StateManager.lvclass">)  [unwired: 8 in]
            n85 = call-dynamic "Create motor.vi"("name"="CALW", "error in (no error)"=w163, "StateManager"=w157, "MotorSim"=w156, "Motor in"=refnum<class "Motor.lvclass"> refnum ("Motor.lvclass")) -> ("error out"=w165:errorcluster, "Motor out"=w158:refnum<class "Motor.lvclass">)  [unwired: 5 in]
          }
          frame 3 {
            n86 = call-dynamic "Write displacements.vi"("error in (no error)"=w176, "displacements"=T11 [{"period"=2000, "initial position (0)"=0, "translation (100)"=4, "forward"=TRUE}, {"period"=2000, "initial position (0)"=4, "translation (100)"=6, "forward"=FALSE}, {"period"=4000, "initial position (0)"=-2, "translation (100)"=32, "forward"=TRUE}, {"period"=2000, "initial position (0)"=30, "translation (100)"=2, "forward"=FALSE}, {"period"=4000, "initial position (0)"=28, "translation (100)"=28, "forward"=FALSE}] ("ASEL moves"), "MotorSim in"=refnum<class "MotorSim.lvclass"> refnum ("MotorSim.lvclass")) -> ("error out"=w171:errorcluster, "MotorSim out"=w168:refnum<class "MotorSim.lvclass">)  [unwired: 7 in]
            n87 = call "Reset state.vi"("error in (no error)"=w171, "StateManager in"=refnum<class "StateManager.lvclass"> refnum ("StateManager.lvclass")) -> ("error out"=w175:errorcluster, "StateManager out"=w169:refnum<class "StateManager.lvclass">)  [unwired: 8 in]
            n88 = call-dynamic "Create motor.vi"("name"="ASEL", "error in (no error)"=w175, "StateManager"=w169, "MotorSim"=w168, "Motor in"=refnum<class "Motor.lvclass"> refnum ("Motor.lvclass")) -> ("error out"=w177:errorcluster, "Motor out"=w170:refnum<class "Motor.lvclass">)  [unwired: 5 in]
          }
          frame 4 {
            n89 = call-dynamic "Write displacements.vi"("error in (no error)"=w188, "displacements"=T11 [{"period"=3000, "initial position (0)"=0, "translation (100)"=370, "forward"=TRUE}, {"period"=3000, "initial position (0)"=370, "translation (100)"=360, "forward"=TRUE}, {"period"=3000, "initial position (0)"=710, "translation (100)"=350, "forward"=TRUE}, {"period"=100, "initial position (0)"=0, "translation (100)"=0, "forward"=TRUE}] ("WPROT moves"), "MotorSim in"=refnum<class "MotorSim.lvclass"> refnum ("MotorSim.lvclass")) -> ("error out"=w183:errorcluster, "MotorSim out"=w180:refnum<class "MotorSim.lvclass">)  [unwired: 7 in]
            n90 = call "Reset state.vi"("error in (no error)"=w183, "StateManager in"=refnum<class "StateManager.lvclass"> refnum ("StateManager.lvclass")) -> ("error out"=w187:errorcluster, "StateManager out"=w181:refnum<class "StateManager.lvclass">)  [unwired: 8 in]
            n91 = call-dynamic "Create motor.vi"("name"="GMIR", "error in (no error)"=w187, "StateManager"=w181, "MotorSim"=w180, "Motor in"=refnum<class "Motor.lvclass"> refnum ("Motor.lvclass")) -> ("error out"=w189:errorcluster, "Motor out"=w182:refnum<class "Motor.lvclass">)  [unwired: 5 in]
          }
          frame 5 {
            n92 = call-dynamic "Write displacements.vi"("error in (no error)"=w200, "displacements"=T11 [{"period"=4000, "initial position (0)"=0, "translation (100)"=21, "forward"=TRUE}, {"period"=4000, "initial position (0)"=21, "translation (100)"=22, "forward"=FALSE}, {"period"=2000, "initial position (0)"=-1, "translation (100)"=1, "forward"=TRUE}] ("GFOC moves"), "MotorSim in"=refnum<class "MotorSim.lvclass"> refnum ("MotorSim.lvclass")) -> ("error out"=w195:errorcluster, "MotorSim out"=w192:refnum<class "MotorSim.lvclass">)  [unwired: 7 in]
            n93 = call "Reset state.vi"("error in (no error)"=w195, "StateManager in"=refnum<class "StateManager.lvclass"> refnum ("StateManager.lvclass")) -> ("error out"=w199:errorcluster, "StateManager out"=w193:refnum<class "StateManager.lvclass">)  [unwired: 8 in]
            n94 = call-dynamic "Create motor.vi"("name"="GFOC", "error in (no error)"=w199, "StateManager"=w193, "MotorSim"=w192, "Motor in"=refnum<class "Motor.lvclass"> refnum ("Motor.lvclass")) -> ("error out"=w201:errorcluster, "Motor out"=w194:refnum<class "Motor.lvclass">)  [unwired: 5 in]
          }
          frame 6, Default {
            # "Useless case: just to take \n\"Default\" from others."
          }
        }
      }
    }
    frame #10 {
      # "CONTROLS WAITING FOR IMPLEMENTATION"
    }
    frame #11 {
      w203 = sgl 0.5 ("Zoom Factor")
      # "ANIMATION: GFOC, GMIR, AND CALW"
      n95 = call <vilib>:"Application Directory.vi"() -> ("Application Directory"=w211:path)
      n96 = property on="calw knob" class="Knob (strict)"("Scale.Visible"=FALSE) -> ()  [unwired: 2 in, 2 out]
      n97 = property on="gmir knob" class="Knob (strict)"("Scale.Visible"=FALSE) -> ()  [unwired: 2 in, 2 out]
      n98 = Build Path(base path=w211, name or relative path="Custom\\Luca transparent.png") -> (appended path=w212:path)
      n99 = call <vilib>:"Read PNG File.vi"("path to PNG file"=w212) -> ("image data"=w209:T2)  [unwired: 8 in, 2 out]
      n100 = call <vilib>:"Draw Flattened Pixmap.vi"("image data"=w209, "picture"=picture data[5B]) -> ("new picture"=→"guider cam anime":picture)  [unwired: 7 in]
      n101 = property on="asel background" class="Pict"("ZoomFactor"=w203) -> ()  [unwired: 2 in, 2 out]
      n102 = property on="asel anime" class="Pict"("ZoomFactor"=w203) -> ()  [unwired: 2 in, 2 out]
      "calw knob" <- cluster{dbl, dbl, dbl, dbl, dbl} {0.0, 72.0, 144.0, 216.0, 288.0} ("Knob")
    }
    frame #12 {
      # "ANIMATION: WPROT, WPSEL, AND ASEL"
      n103 = call <vilib>:"Application Directory.vi"() -> ("Application Directory"=w228:path)
      n104 = call <vilib>:"Application Directory.vi"() -> ("Application Directory"=w218:path)
      n105 = call <vilib>:"Application Directory.vi"() -> ("Application Directory"=w222:path)
      n106 = Build Path(base path=w228, name or relative path="Custom\\wpsel transparent.png") -> (appended path=w229:path)
      n107 = Build Path(base path=w218, name or relative path="Custom\\asel transparent.png") -> (appended path=w217:path)
      n108 = Build Path(base path=w222, name or relative path="Custom\\asel background.png") -> (appended path=w223:path)
      n109 = call <vilib>:"Read PNG File.vi"("path to PNG file"=w229) -> ("image data"=w226:T2)  [unwired: 8 in, 2 out]
      n110 = call <vilib>:"Read PNG File.vi"("path to PNG file"=w223) -> ("image data"=w221:T2)  [unwired: 8 in, 2 out]
      n111 = call <vilib>:"Draw Flattened Pixmap.vi"("image data"=w226, "picture"=picture data[5B]) -> ("new picture"=→"wpsel anime":picture)  [unwired: 7 in]
      n112 = call <vilib>:"Read PNG File.vi"("path to PNG file"=w217) -> ("image data"=→"asel image":T2)  [unwired: 8 in, 2 out]
      n113 = call <vilib>:"Draw Flattened Pixmap.vi"("image data"=w221, "picture"=picture data[5B]) -> ("new picture"=→"asel background":picture)  [unwired: 7 in]
      n114 = property on="asel image" class="Clust (strict)"("Visible"=FALSE) -> ()  [unwired: 2 in, 2 out]
    }
    frame #13 {
      w230 = TRUE
      w231 = FALSE
      # "MECHANISM STATUS DISPLAY"
      n115 = property on="wprot stat" class="Clust (strict)"("Visible"=w231) -> ()  [unwired: 2 in, 2 out]
      n116 = property on="wpsel stat" class="Clust (strict)"("Visible"=w231) -> ()  [unwired: 2 in, 2 out]
      n117 = property on="GFOC Value" class="DigNum (strict)"("Visible"=w230) -> ()  [unwired: 2 in, 2 out]
      n118 = property on="WPROT Value" class="DigNum (strict)"("Visible"=w230) -> ()  [unwired: 2 in, 2 out]
      n119 = property on="asel stat" class="Clust (strict)"("Visible"=w231) -> ()  [unwired: 2 in, 2 out]
      n120 = property on="calw stat" class="Clust (strict)"("Visible"=w231) -> ()  [unwired: 2 in, 2 out]
      n121 = property on="GMIR Value" class="DigNum (strict)"("Visible"=w230) -> ()  [unwired: 2 in, 2 out]
      n122 = property on="WPSEL Value" class="DigNum (strict)"("Visible"=w230) -> ()  [unwired: 2 in, 2 out]
      n123 = property on="gmir stat" class="Clust (strict)"("Visible"=w231) -> ()  [unwired: 2 in, 2 out]
      n124 = property on="gfoc stat" class="Clust (strict)"("Visible"=w231) -> ()  [unwired: 2 in, 2 out]
      n125 = property on="CALW Value" class="DigNum (strict)"("Visible"=w230) -> ()  [unwired: 2 in, 2 out]
      n126 = property on="ASEL Value" class="DigNum (strict)"("Visible"=w230) -> ()  [unwired: 2 in, 2 out]
    }
    frame #14 {
      # "PELA URGÊNCIA, OS PARÂMETROS DE PUB 0MQ\nFORAM  INSERIDOS  NA CLASSE MESSENGER."
      # "CREATE THE QUEUED COMMUNICATION OBJECTS"
      n127 = call-dynamic "Create messenger.vi"("InterComm path"=path "InterComm.vi", "0mqComm path"=path "0mqComm.vi" ("InterComm path"), "error in (no error)"=w240, "S4statusQueueName"="S4status", "S4commandQueueName"="S4command", "Messenger in"=refnum<class "Messenger.lvclass"> refnum) -> ("error out"=w236:errorcluster, "Messenger out"=w233:refnum<class "Messenger.lvclass">)  [unwired: 4 in]
      n128 = call-dynamic "Create queues.vi"("error in (no error)"=w236, "timeout"=500, "Messenger in"=w233) -> ("error out"=w235:errorcluster, "Messenger out"=w234:refnum<class "Messenger.lvclass">)  [unwired: 7 in]
    }
    frame #15 {
      w243 = FALSE ("commWPROT")
      # "RESET THE COMMUNICATION LEDS"
      "commCALW" <- w243
      "commGMIR" <- w243
      "commASEL" <- w243
      "commWPROT" <- w243
      "commWPSEL" <- w243
      "commGFOC" <- w243
    }
  }
  "cfgFile" <- w27
  n129 = Create User Event(user event datatype=w12) -> (user event=w11:refnum<user-event>)  [unwired: 1 in, 1 out]
  n130 = call "Create ICS.vi"("Messenger"=w14, "error in (no error)"=w15, "motors"=w25, "control indices"=w26, "email settings"=w24) -> ("error out"=w29:errorcluster, "ICS out"=w16:refnum<class "ICS.lvclass">)  [unwired: 5 in]
  n131 = register-events(w11) -> (reference out=w9:refnum<event-registration>)  [unwired: 2 in, 1 out]
  n132 = call <vilib>:"Application Directory.vi"() -> ("Application Directory"=w23:path)
  n133 = Get Control Values by Index(1:w26, 3:w29) -> (10:w18:variant[], 11:w22:errorcluster)  [unwired: 1 in]
  n134 = Build Path(base path=w23, name or relative path=w27) -> (appended path=w20:path)
  n135 = call "Config file.vi"("path"=w20, "access (0:read/write)"=enum16{"read/write", "read-only", "write-only"}."read-only", "error in (no error)"=w22, "data values"=w18, "email settings"=w24) -> ("error out"=w21:errorcluster, "data out"=w17:variant[])  [unwired: 5 in]
  n136 = Set Control Values by Index(1:w26, 2:w17, 3:w21) -> (11:w2:errorcluster)  [unwired: 1 in]
  n137 = stacked-sequence {
    tunnel: w2 -> [w244 _ _]
    tunnel: [_ _ w253] -> w1
    frame #0 {
      n138 = case shown="True" "runMinimized" {
        tunnel: w244 -> [_ w248]
        tunnel: T13."Minimized" ("Front Panel Window:State") -> [_ w247]
        frame False {
        }
        frame True {
          n139 = property class="VI"(error in=w248, "Front Panel Window:State"=w247) -> ()  [unwired: 1 in, 2 out]
        }
      }
    }
    frame #1 {
      # "20240718"
      # "20240621"
      n140 = local read "version"() -> (w252:string)
      n141 = call "Write log to file.vi"("prefix"="START" ("current priority"), "version"=w252, "current priority"="6", "enabled priority"="enabled log") -> ()  [unwired: 5 in, 3 out]
    }
    frame #2 {
      n142 = Concatenate Strings("address", ":" ("string"), "0mqEndpoint") -> (w253:string)
    }
  }
  n143 = while {
    shift-right: [w267] -> w30
    shift-left: w16 -> [w270]
    shift-right: [w266] -> w10
    shift-left: w2 -> [w271]
    shift-right: [w268] -> _
    shift-left: 0 -> [w269]
    tunnel: w9 -> [w264]
    tunnel: w11 -> [w263]
    tunnel: w9 -> [w262]
    stop <- w257 stop-if-true
    # "PUB\nZEROMQ"
    # "AQUI DEVE SER PUBLICANDO O STATUS DO S4ICS\nCASO ELE TENHA SIDO ALTERADO.\n\nO VI 0mqComm SE ENCARREGA DE \nPUBLICAR O STATUS PERIODICAMENTE"
    n144 = event shown="[8] \"start server\": Value Change;  <autoServerStart>: User Event" {
      selector: w264 -> [_ _ _ _ _ _ _ _ _ _ _ _ _ _ _ _ _ _ _ _ _ _ _ _ _ _ _ _ _ _ _ _ _ _ _ _ _ _]
      dyn-events: _ -> [_ _ _ _ _ _ _ _ _ _ _ _ _ _ _ _ _ _ _ _ _ _ _ _ _ _ _ _ _ _ _ _ _ _ _ _ _ _]
      timeout: 20 -> [_ _ _ _ _ _ _ _ _ _ _ _ _ _ _ _ _ _ _ _ _ _ _ _ _ _ _ _ _ _ _ _ _ _ _ _ _ _]
      tunnel: w270 -> [w400 w1770 w1828 w1839 w1841 w1916 w1924 w1960 w2083 w2221 w2247 w2251 w2255 w2260 w2289 w2352 w2414 w2416 w2417 w2420 w2422 w2424 w2425 w2434 w2443 w2461 w2509 w2551 w2594 w2610 w2616 w2638 w2653 w2664 w2681 w2714 w2763 w2786]
      tunnel: w271 -> [w410 w1769 w1827 w1838 w1840 w1915 w1923 w1959 w2082 w2220 w2246 w2250 w2256 w2259 w2290 w2353 w2413 w2415 w2418 w2419 w2421 w2423 w2426 w2433 w2442 w2462 w2510 w2550 w2591 w2609 w2615 w2626 w2652 w2663 w2682 w2711 w2760 w2787]
      tunnel: [w407 w1769 w1827 w1838 w1858 w1915 w1923 w1944 w2033 w2219 w2235 w2250 w2254 w2259 w2280 w2350 w2413 w2415 w2418 w2419 w2421 w2423 w2426 w2433 w2442 w2463 w2508 w2550 w2593 w2609 w2615 w2632 w2652 w2662 w2685 w2710 w2759 w2784] -> w260
      tunnel: [w406 w1770 w1828 w1839 w1859 w1916 w1924 w1943 w2096 w2218 w2234 w2251 w2253 w2260 w2287 w2351 w2414 w2416 w2417 w2420 w2422 w2424 w2425 w2434 w2443 w2459 w2506 w2551 w2592 w2610 w2616 w2631 w2653 w2661 w2679 w2714 w2763 w2785] -> w261
      tunnel: w269 -> [w403 _ _ _ _ _ _ _ _ _ _ _ _ _ _ _ _ _ _ _ _ _ _ _ _ _ _ _ _ _ _ _ _ _ _ _ _ _]
      tunnel: [w402 _ _ _ _ _ _ _ _ _ _ _ _ _ _ _ _ _ _ _ _ _ _ _ _ _ _ _ _ _ _ _ _ _ _ _ _ _] -> w268
      tunnel: w263 -> [w399 _ _ _ _ _ _ _ _ _ _ _ _ _ _ _ _ _ _ _ _ _ _ _ _ _ _ _ _ _ _ _ _ _ _ _ _ _]
      tunnel: w262 -> [w398 _ _ _ _ _ _ _ _ _ _ _ _ _ _ _ _ _ _ _ _ _ _ _ _ _ _ _ _ _ _ _ _ _ _ _ _ _]
      tunnel: [_ _ _ _ _ _ _ _ FALSE TRUE TRUE _ _ _ _ _ _ _ _ _ _ _ _ _ _ _ _ _ _ _ _ _ _ _ _ _ _ _] -> w257
      event Timeout {
        # "CHECK FOR SERVER ENABLE"
        n145 = event-data() -> ()  [unwired: 1 in, 3 out]
        n146 = local read "server"() -> (w405:bool)
        n147 = call-dynamic "Check moving.vi"("error in (no error)"=w410, "ICS in"=w400) -> ("error out"=w409:errorcluster, "in motion"=w401:bool, "ICS out"=w408:refnum<class "ICS.lvclass">)  [unwired: 7 in]
        n148 = Or(x=w401, y=w405) -> (x .or. y?=w404:bool)
        n149 = case shown="True" w404 {
          tunnel: w409 -> [w415 w468]
          tunnel: w408 -> [w416 w466]
          tunnel: [w412 w470] -> w407
          tunnel: [w411 w469] -> w406
          tunnel: w403 -> [w429 _]
          tunnel: [w426 _] -> w402
          tunnel: w399 -> [w421 _]
          tunnel: w398 -> [w417 w455]
          frame False {
            # "READ AND DISCARD 0MQ PULL MESSAGES"
            # "CHECK FOR AUTOMATIC LOGOUT"
            n150 = First Call?() -> (First Call?: T/F=w420:bool)
            n151 = call-dynamic "Read Messenger.vi"("error in (no error)"=w415, "ICS in"=w416) -> ("error out"=w413:errorcluster, "Messenger.lvclass"=w414:refnum<class "Messenger.lvclass">, "ICS out"=w411:refnum<class "ICS.lvclass">)  [unwired: 7 in]
            n152 = And(x=w420, y="autoSS") -> (x .and. y?=w418:bool)
            n153 = case shown="True" w418 {
              selector: w418 -> [_ w431]
              tunnel: w421 -> [_ w436]
              tunnel: w417 -> [_ _]
              frame False {
              }
              frame True {
                w435 = T12."Disabled and Grayed Out" ("Disabled")
                n154 = Generate User Event(user event=w436, event data cluster=w431) -> (user event out=w430:refnum<user-event>)  [unwired: 2 in, 1 out]
                n155 = Destroy User Event(user event=w430) -> ()  [unwired: 1 in, 1 out]
                n156 = property on="assist" class="Bool"("DisabledEnum"=w435) -> ()  [unwired: 2 in, 2 out]
                n157 = property on="setup" class="Bool"("DisabledEnum"=w435) -> ()  [unwired: 2 in, 2 out]
                n158 = property on="control" class="Bool"("DisabledEnum"=w435) -> ()  [unwired: 2 in, 2 out]
                n159 = property on="start server" class="Bool"("DisabledEnum"=T12."Enabled" ("Disabled")) -> ()  [unwired: 2 in, 2 out]
                n160 = local write "tab menu"(T6."Stopped" ("tab menu")) -> ()
                n161 = local write "tab body"(enum32{"Motors", "Config"}."Motors" ("tab body")) -> ()
              }
            }
            n162 = call-dynamic "Get command.vi"("error in (no error)"=w413, "Messenger in"=w414) -> ("error out"=w412:errorcluster)  [unwired: 6 in, 3 out]
            n163 = local read "tab menu"() -> (w427:T6)
            n164 = Multiply(x="auto logout", y=1000 ("f")) -> (x*y=w422:u32)
            n165 = Not Equal?(x=w427, y=T15."Login" ("tab menu")) -> (x != y?=w425:bool)
            n166 = case shown="True" w425 {
              tunnel: w429 -> [_ w440]
              tunnel: [0 w441] -> w426
              tunnel: w422 -> [_ w438]
              frame False {
              }
              frame True {
                n167 = Greater?(x=w440, y=w438) -> (0:w439:bool)
                n168 = case shown="True" w439 {
                  tunnel: w440 -> [w444 _]
                  tunnel: [w442 0] -> w441
                  frame False {
                    # "KEEP COUNTING"
                    n169 = Add(x=w444, y=5) -> (x+y=w442:i32)
                  }
                  frame True {
                    w450 = ""
                    # "LOGOUT"
                    n170 = local write "tab menu"(T6."Login" ("tab menu")) -> ()
                    n171 = local write "tab body"(enum32{"Motors", "Config"}."Motors" ("tab body")) -> ()
                    n172 = local write "loginPW"(w450) -> ()
                    n173 = local write "loginUser"(w450) -> ()
                    n174 = local read "server"() -> (w445:bool)
                    n175 = Not(x=w445) -> (.not. x?=w451:bool)
                    n176 = property on="exitLogin" class="Bool"("Visible"=w451) -> ()  [unwired: 2 in, 2 out]
                    n177 = property on="loginUser" class="Str"("Key Focus"=TRUE) -> ()  [unwired: 2 in, 2 out]
                  }
                }
              }
            }
          }
          frame True {
            # "CHECK FOR INCOMMING MESSAGES FROM CLIENTS"
            n178 = local read "channel"() -> (w465:T5)
            n179 = call-dynamic "Read motors.vi"("ICS in"=w466) -> ("motors"=w463:refnum<class "Motor.lvclass">[])  [unwired: 8 in, 2 out]
            n180 = First Call?() -> (First Call?: T/F=w454:bool)
            n181 = Equal?(x=w465, y=T5."Inner TCP/IP" ("channel")) -> (x = y?=w453:bool)
            n182 = case shown="True" w453 {
              tunnel: w468 -> [w488 w507]
              tunnel: [w487 w506] -> w467
              tunnel: w466 -> [w486 w508]
              tunnel: [w485 w505] -> w458
              tunnel: [w484 w504] -> w456
              tunnel: [w483 w503] -> w462
              tunnel: [FALSE w502] -> w452
              frame False {
                # "READ CLIENT COMMAND\nUSING INTERCOMM VI"
                n183 = disable-structure shown="Enabled" {
                  disable-tunnel: w488 -> [w499 w501]
                  disable-tunnel: [w492 w500] -> w487
                  disable-tunnel: w486 -> [w498 w500]
                  disable-tunnel: [w497 _] -> w485
                  disable-tunnel: [w496 _] -> w484
                  disable-tunnel: [w489 w501] -> w483
                  frame Enabled {
                    n184 = call-dynamic "Read Messenger.vi"("error in (no error)"=w499, "ICS in"=w498) -> ("error out"=w495:errorcluster, "Messenger.lvclass"=w494:refnum<class "Messenger.lvclass">, "ICS out"=w493:refnum<class "ICS.lvclass">)  [unwired: 7 in]
                    n185 = call-dynamic "Get command.vi"("error in (no error)"=w495, "Messenger in"=w494) -> ("error out"=w490:errorcluster, "isAcommand"=w496:bool, "command"=w497:string, "Messenger out"=w491:refnum<class "Messenger.lvclass">)  [unwired: 6 in]
                    n186 = call-dynamic "Write Messenger.vi"("error in (no error)"=w490, "Messenger.lvclass"=w491, "ICS in"=w493) -> ("error out"=w489:errorcluster, "ICS out"=w492:refnum<class "ICS.lvclass">)  [unwired: 7 in]
                  }
                  frame Disabled {
                  }
                }
              }
              frame True {
                # "READ CLIENT COMMAND\nUSING INNER TCP/IP CONNECTION\nAND/OR ZEROMQ PULL"
                n187 = disable-structure shown="Disabled" {
                  disable-tunnel: w508 -> [w519 w534]
                  disable-tunnel: w507 -> [w518 w535]
                  disable-tunnel: [w515 w533] -> w506
                  disable-tunnel: [w511 w532] -> w505
                  disable-tunnel: [w510 w531] -> w504
                  disable-tunnel: [w509 w536] -> w503
                  disable-tunnel: [_ w530] -> w502
                  frame Disabled {
                    n188 = call "Read Server.vi"("error in (no error)"=w518, "ICS in"=w519) -> ("error out"=w517:errorcluster, "Server"=w520:refnum<class "TCP-Server.lvclass">, "ICS out"=w516:refnum<class "ICS.lvclass">)  [unwired: 7 in]
                    n189 = call-dynamic "Wait on listenner.vi"("error in (no error)"=w517, "Server in"=w520) -> ("error out"=w513:errorcluster, "Server out"=w514:refnum<class "TCP-Server.lvclass">)  [unwired: 8 in]
                    n190 = call "Write Server.vi"("error in (no error)"=w513, "Server"=w514, "ICS in"=w516) -> ("error out"=w512:errorcluster, "ICS out"=w515:refnum<class "ICS.lvclass">)  [unwired: 7 in]
                    n191 = case shown="Error" w512 {
                      selector: w512 -> [w525 w528]
                      tunnel: w514 -> [w521 _]
                      tunnel: [w524 w527] -> w509
                      tunnel: [w522 FALSE] -> w510
                      tunnel: [w523 _] -> w511
                      frame No Error {
                        n192 = call-dynamic "Receive message.vi"("error in (no error)"=w525, "Server in"=w521) -> ("error out"=w524:errorcluster, "isAcommand"=w522:bool, "message"=w523:string)  [unwired: 6 in, 1 out]
                      }
                      frame Error {
                        n193 = call <vilib>:"Clear Errors.vi"("error in (no error)"=w528, "specific error code to clear (0: all)"=56) -> ("error out"=w527:errorcluster)  [unwired: 4 in, 1 out]
                      }
                    }
                  }
                  frame Enabled {
                    n194 = call-dynamic "Read 0mq-Tcp command.vi"("error in (no error)"=w535, "ICS in"=w534) -> ("error out"=w536:errorcluster, "isAcommand"=w531:bool, "command"=w532:string, "ICS out"=w533:refnum<class "ICS.lvclass">, "rec0mq"=w530:bool)  [unwired: 5 in]
                  }
                }
              }
            }
            n195 = for {
              tunnel: w463 -> [w473] mode=indexing
              # "UPDATE STATUS DISPLAY"
              n196 = call-dynamic "Read status.vi"("Motor in"=w473) -> ("name"=w475:string, "status"=w474:T1)  [unwired: 7 in, 2 out]
              n197 = case shown="\"ASEL\"" w475 {
                tunnel: w474 -> [w476 w477 w478 w479 w480 w481]
                frame "Default", Default {
                  "gfoc stat" <- w476
                }
                frame "WPROT" {
                  "wprot stat" <- w477
                }
                frame "WPSEL" {
                  "wpsel stat" <- w478
                }
                frame "ASEL" {
                  "asel stat" <- w479
                }
                frame "CALW" {
                  "calw stat" <- w480
                }
                frame "GMIR" {
                  "gmir stat" <- w481
                }
              }
            }
            n198 = case shown="True" w454 {
              tunnel: w455 -> [_ w472]
              frame False {
              }
              frame True {
                n199 = Unregister For Events(event registration refnum=w472) -> (error out=w471:errorcluster)  [unwired: 1 in]
                n200 = call <vilib>:"Clear Errors.vi"("error in (no error)"=w471) -> ()  [unwired: 5 in, 2 out]
              }
            }
            n201 = call "Check message.vi"("error in (no error)"=w462, "isAcommand"=w456, "message in"=w458) -> ("error out"=w461:errorcluster, "valid"=w460:bool, "message"=w459:string, "not empty"=w457:bool)  [unwired: 5 in]
            n202 = case shown="False" w460 {
              tunnel: [w538 w1632] -> w470
              tunnel: w467 -> [w544 w1639]
              tunnel: [w539 w1633] -> w469
              tunnel: w459 -> [_ w1613]
              tunnel: w461 -> [w537 w1640]
              tunnel: w457 -> [_ w1635]
              tunnel: w453 -> [_ w1602]
              tunnel: w452 -> [_ w1601]
              frame False {
                # "NO CLIENT CONNECTION: TAKE CARE OF MECHANISMS"
                n203 = call-dynamic "Select motor.vi"("error in (no error)"=w537, "ICS in"=w544) -> ("error out"=w540:errorcluster, "valid"=w543:bool, "selected motor"=w542:refnum<class "Motor.lvclass">, "ICS out"=w541:refnum<class "ICS.lvclass">)  [unwired: 6 in]
                n204 = case shown="True" w543 {
                  tunnel: w542 -> [_ w700]
                  tunnel: [w546 w688] -> w538
                  tunnel: w541 -> [w547 w680]
                  tunnel: w540 -> [w548 w699]
                  tunnel: [w545 w691] -> w539
                  frame False {
                    # "NO MOTOR SELECTED, GET UPDATED MOTOR INFORMATION"
                    n205 = disable-structure shown="Enabled" {
                      disable-tunnel: w548 -> [w568 w602 w675]
                      disable-tunnel: w547 -> [w567 w603 w676]
                      disable-tunnel: [w551 w604 w675] -> w546
                      disable-tunnel: [w550 w605 w676] -> w545
                      frame Disabled {
                        # "DEPOIS DE TESTAR O FUNCIONAMENTO,\nCRIAR UM VI PARA SELECIONAR UM MOTOR\nQUE ESTEJA HABILITADO E NO MODO CONTROL"
                        n206 = call-dynamic "Read motors.vi"("error in (no error)"=w568, "ICS in"=w567) -> ("error out"=w565:errorcluster, "motors"=w552:refnum<class "Motor.lvclass">[], "ICS out"=w566:refnum<class "ICS.lvclass">)  [unwired: 7 in]
                        n207 = call-dynamic "Read MotorManager.vi"("error in (no error)"=w565, "ICS in"=w566) -> ("error out"=w570:errorcluster, "MotorManager.lvclass"=w569:refnum<class "MotorManager.lvclass">, "ICS out"=w553:refnum<class "ICS.lvclass">)  [unwired: 7 in]
                        n208 = Build Array("GS0", "V31") -> (w560:string[])
                        n209 = call-dynamic "Read current state.vi"("error in (no error)"=w570, "StateManager in"=w569) -> ("error out"=w564:errorcluster, "currentState"=w554:u32, "StateManager out"=w555:refnum<class "MotorManager.lvclass">)  [unwired: 7 in]
                        n210 = Index Array(array=w552, index=w554) -> (element=w563:refnum<class "Motor.lvclass">)
                        n211 = Wait (ms)(milliseconds to wait=u32 50) -> ()  [unwired: 1 out]
                        n212 = call-dynamic "Send instructions.vi"("error in (no error)"=w564, "instructions"=w560, "Motor in"=w563) -> ("error out"=w557:errorcluster, "error"=w558:bool, "replies"=w559:string[], "Motor out"=w556:refnum<class "Motor.lvclass">)  [unwired: 4 in, 1 out]
                        n213 = case shown="False" w558 {
                          tunnel: w559 -> [w595 _]
                          tunnel: w557 -> [w594 w597]
                          tunnel: w556 -> [w593 _]
                          tunnel: w555 -> [w576 _]
                          tunnel: w554 -> [w583 _]
                          tunnel: w553 -> [w579 w596]
                          tunnel: w552 -> [w584 _]
                          tunnel: [w572 w597] -> w551
                          tunnel: [w571 w596] -> w550
                          frame False {
                            # "STORE MOTOR INFO AND SELECT ANOTHER MOTOR FOR NEXT READING"
                            n214 = Increment(x=w583) -> (x+1=w586:u32)
                            n215 = Index Array(array=w595, index=1) -> (element=w592:string)
                            n216 = Decimal String To Number(string=w592, default (0L)=u32 0 ("default (0 I32)")) -> (number=w591:u32)  [unwired: 1 in, 1 out]
                            n217 = Greater Or Equal?(x=w586, y=u32 5) -> (x >= y?=w587:bool)
                            n218 = call-dynamic "Write motor info.vi"("error in (no error)"=w594, "motor info"=w591, "Motor in"=w593) -> ("error out"=w581:errorcluster, "Motor out"=w582:refnum<class "Motor.lvclass">)  [unwired: 7 in]
                            n219 = Select(t=u32 0 ("y"), s=w587, f=w586) -> (s? t:f=w577:u32)
                            n220 = Replace Array Subset(array=w584, new element=w582, index=w583) -> (w580:refnum<class "Motor.lvclass">[])
                            n221 = call-dynamic "Write motors.vi"("error in (no error)"=w581, "motors"=w580, "ICS in"=w579) -> ("error out"=w578:errorcluster, "ICS out"=w574:refnum<class "ICS.lvclass">)  [unwired: 7 in]
                            n222 = call-dynamic "Write current state.vi"("error in (no error)"=w578, "currentState"=w577, "StateManager in"=w576) -> ("error out"=w575:errorcluster, "StateManager out"=w573:refnum<class "MotorManager.lvclass">)  [unwired: 7 in]
                            n223 = call-dynamic "Write MotorManager.vi"("error in (no error)"=w575, "MotorManager.lvclass"=w573, "ICS in"=w574) -> ("error out"=w572:errorcluster, "ICS out"=w571:refnum<class "ICS.lvclass">)  [unwired: 7 in]
                          }
                          frame True {
                            # "NO RESPONSE FROM MOTOR"
                          }
                        }
                      }
                      frame Disabled {
                        n224 = Tick Count (ms)() -> (millisecond timer value=w598:u32)
                        n225 = call-dynamic "Check moving.vi"("error in (no error)"=w602, "ICS in"=w603) -> ("error out"=w600:errorcluster, "in motion"=w599:bool, "ICS out"=w601:refnum<class "ICS.lvclass">)  [unwired: 7 in]
                        n226 = case shown="False" w599 {
                          tunnel: w601 -> [w615 w673]
                          tunnel: w600 -> [w614 w674]
                          tunnel: [w613 w673] -> w605
                          tunnel: [w612 w674] -> w604
                          tunnel: w598 -> [w606 _]
                          frame False {
                            # "V46 DE S4DMX FOI ALTERADO:\nV46 < 0   MOTOR SEM INIT\nV46 = 0   MOTOR PARADO\nV46 = 1   MOTOR BUSY \nV46 > 10  ERRO NO MOVIMENTO."
                            # "NO MECHANISM IS MOVING, CHECK MOTORS"
                            n227 = call-dynamic "Read motors.vi"("error in (no error)"=w614, "ICS in"=w615) -> ("error out"=w609:errorcluster, "motors"=w610:refnum<class "Motor.lvclass">[], "ICS out"=w611:refnum<class "ICS.lvclass">)  [unwired: 7 in]
                            n228 = for {
                              tunnel: w610 -> [w624] mode=indexing
                              tunnel: w609 -> [w623]
                              tunnel: [w625] -> w608 mode=indexing
                              tunnel: [w618] -> w607
                              n229 = call-dynamic "Read status.vi"("error in (no error)"=w623, "Motor in"=w624) -> ("error out"=w621:errorcluster, "name"=w619:string, "status"=w620:T1, "Motor out"=w622:refnum<class "Motor.lvclass">)  [unwired: 6 in]
                              n230 = case shown="\"ANY\", Default" w619 {
                                tunnel: [w626 w639] -> w625
                                tunnel: w622 -> [w626 w638]
                                tunnel: w621 -> [_ w637]
                                tunnel: w620 -> [_ w636]
                                frame "GFOC" {
                                }
                                frame "ANY", Default {
                                n231 = local read "enabled log"() -> (w646:string)
                                n232 = local read "version"() -> (w645:string)
                                n233 = Build Array("V46") -> (w648:string[])
                                n234 = call-dynamic "Send check instructions.vi"("version"=w645, "current code"="7", "enabled codes"=w646, "error in (no error)"=w637, "prefix"="CHECK", "instructions"=w648, "Motor in"=w638) -> ("error out"=w640:errorcluster, "error"=w634:bool, "replies"=w643:string[], "Motor out"=w641:refnum<class "Motor.lvclass">)  [unwired: 1 out]
                                n235 = Index Array(array=w643, index=0) -> (element=w635:string)
                                n236 = Select(t="10" ("current code"), s=w634, f=w635) -> (s? t:f=w632:string)
                                n237 = Decimal String To Number(string=w632, default (0L)=0 ("index")) -> (number=w628:i32)  [unwired: 1 in, 1 out]
                                n238 = Less Than 0?(x=w628) -> (x < 0?=w630:bool)
                                n239 = Select(t=-1 ("index"), s=w630, f=w628) -> (s? t:f=w627:i32)
                                n240 = case shown="-1" w627 {
                                tunnel: w641 -> [w656 w658 w665 w672]
                                tunnel: w640 -> [w655 w657 w664 w671]
                                tunnel: [w653 w658 w662 w669] -> w639
                                tunnel: [w652 w657 w661 w668] -> _
                                tunnel: w636 -> [w650 _ w659 w666]
                                frame -1 {
                                # "POWER OFF"
                                n241 = Bundle By Name(cluster=w650, "condition"="NONE") -> (w654:T1)
                                n242 = call-dynamic "Write status.vi"("error in (no error)"=w655, "status"=w654, "Motor in"=w656) -> ("error out"=w652:errorcluster, "Motor out"=w653:refnum<class "Motor.lvclass">)  [unwired: 7 in]
                                }
                                frame 0 {
                                # "READY"
                                }
                                frame 1 {
                                # "BUSY"
                                n243 = Bundle By Name(cluster=w659, "condition"="TIMEOUT") -> (w663:T1)
                                n244 = call-dynamic "Write status.vi"("error in (no error)"=w664, "status"=w663, "Motor in"=w665) -> ("error out"=w661:errorcluster, "Motor out"=w662:refnum<class "Motor.lvclass">)  [unwired: 7 in]
                                }
                                frame 10, Default {
                                # "SUB ERROR"
                                n245 = Bundle By Name(cluster=w666, "condition"="TIMEOUT") -> (w670:T1)
                                n246 = call-dynamic "Write status.vi"("error in (no error)"=w671, "status"=w670, "Motor in"=w672) -> ("error out"=w668:errorcluster, "Motor out"=w669:refnum<class "Motor.lvclass">)  [unwired: 7 in]
                                }
                                }
                                }
                              }
                              n247 = Tick Count (ms)() -> (millisecond timer value=w618:u32)
                            }
                            n248 = disable-structure shown="Disabled" {
                              disable-tunnel: w607 -> [w617 _]
                              disable-tunnel: w606 -> [w616 _]
                              frame Disabled {
                                # "100 ms"
                                n249 = Subtract(x=w617, y=w616) -> ()  [unwired: 1 out]
                              }
                              frame Enabled {
                              }
                            }
                            n250 = call-dynamic "Write motors.vi"("error in (no error)"=w609, "motors"=w608, "ICS in"=w611) -> ("error out"=w612:errorcluster, "ICS out"=w613:refnum<class "ICS.lvclass">)  [unwired: 7 in]
                          }
                          frame True {
                          }
                        }
                      }
                      frame Enabled {
                        # "FICOU PARA A PRÓXIMA VERSÃO O CKECK DO MOTOR\nTALVEZ SEJA MELHOR FAZER ISSO NUM LOOP SEPARADO."
                      }
                    }
                  }
                  frame True {
                    # "20240718"
                    # "PROCESS SELECTED MOTOR"
                    n251 = call-dynamic "Read StateManager.vi"("error in (no error)"=w699, "Motor in"=w700) -> ("error out"=w697:errorcluster, "StateManager"=w698:refnum<class "StateManager.lvclass">, "Motor out"=w685:refnum<class "Motor.lvclass">, "stateEnum"=w694:T16)  [unwired: 5 in, 1 out]
                    n252 = call-dynamic "Read current state.vi"("error in (no error)"=w697, "StateManager in"=w698) -> ("error out"=w696:errorcluster, "currentState"=w695:u32, "StateManager out"=w679:refnum<class "StateManager.lvclass">)  [unwired: 7 in]
                    n253 = local read "version"() -> (w677:string)
                    n254 = Variant To Data(error in=w696, type=w694, Variant=w695) -> (data=w687:T16, error out=w686:errorcluster)
                    n255 = case shown="\"ActiveGoto\"" w687 {
                      tunnel: w686 -> [w704 w759 w815 w884 w915 w1037 w1105 w1188 w1236 w1341 w1415 w1473 w1526]
                      tunnel: w685 -> [w706 w758 w816 w885 w916 w1036 w1104 w1187 w1235 w1340 w1416 w1474 w1527]
                      tunnel: [w707 w766 w825 w887 w909 w1009 w1100 w1183 w1229 w1319 w1418 w1477 w1512] -> w684
                      tunnel: [w702 w762 w820 w881 w901 w988 w1101 w1185 w1233 w1338 w1400 w1467 w1528] -> w683
                      tunnel: [w705 w765 w824 w886 w908 w1035 w1099 w1182 w1228 w1337 w1417 w1476 w1511] -> w682
                      tunnel: [w703 w763 w821 w879 w902 w989 w1102 w1186 w1234 w1339 w1399 w1466 w1510] -> w681
                      tunnel: w680 -> [w707 w766 w825 w887 w909 w1025 w1100 w1183 w1229 w1320 w1418 w1477 w1512]
                      tunnel: w679 -> [w705 w765 w824 w886 w908 w1035 w1099 w1182 w1228 w1337 w1417 w1476 w1511]
                      tunnel: [w701 w761 w819 w868 w900 T16."Wait" ("stateEnum") T16."SimUptate" ("stateEnum") T16."SimUptate" ("stateEnum") w1232 T16."Wait" ("stateEnum") w1419 w1456 w1508] -> w678
                      tunnel: w677 -> [_ w749 w808 w866 w892 w993 _ _ _ _ w1390 w1451 w1507]
                      frame "Wait", Default {
                        # "CHECK FOR RECEIVED COMMAND (ACK = TRUE) - MOTOR STATE MACHINE"
                        n256 = call-dynamic "Read ack flag.vi"("error in (no error)"=w704, "Motor in"=w706) -> ("error out"=w713:errorcluster, "ack"=w716:bool, "Motor out"=w714:refnum<class "Motor.lvclass">)  [unwired: 6 in, 1 out]
                        n257 = call "Read mode.vi"("error in (no error)"=w713, "Motor in"=w714) -> ("error out"=w711:errorcluster, "mode"=w715:string, "Motor out"=w712:refnum<class "Motor.lvclass">)  [unwired: 7 in]
                        n258 = call-dynamic "Read action-param.vi"("error in (no error)"=w711, "Motor in"=w712) -> ("error out"=w708:errorcluster, "action"=w710:string, "Motor out"=w709:refnum<class "Motor.lvclass">)  [unwired: 6 in, 1 out]
                        n259 = case shown="True" w716 {
                          tunnel: w715 -> [_ w728]
                          tunnel: w710 -> [_ w727]
                          tunnel: [T16."Wait" ("stateEnum") w721] -> w701
                          tunnel: w709 -> [w718 w725]
                          tunnel: w708 -> [w719 w724]
                          tunnel: [w718 w723] -> w702
                          tunnel: [w719 w722] -> w703
                          frame False {
                            # "NO COMMAND WAS RECEIVED"
                          }
                          frame True {
                            # "COMMAND RECEIVED, SET NEXT STATE"
                            n260 = case shown="\"ACTIVE\"" w728 {
                              tunnel: w727 -> [_ w737 w744]
                              tunnel: [T16."Wait" ("stateEnum") w736 w743] -> w721
                              frame "NONE", Default {
                              }
                              frame "ACTIVE" {
                                n261 = case shown="\"STOP\"" w737 {
                                tunnel: [T16."ActiveInit" ("stateEnum") T16."ActiveGoto" ("stateEnum") T16."CyclicStart" ("stateEnum") T16."ActiveStop" ("stateEnum") T16."Wait" ("stateEnum")] -> w736
                                frame "INIT" {
                                }
                                frame "GOTO" {
                                }
                                frame "CYCLIC" {
                                }
                                frame "STOP" {
                                }
                                frame "NONE", Default {
                                }
                                }
                              }
                              frame "SIMULATED" {
                                n262 = case shown="\"STOP\"" w744 {
                                tunnel: [T16."SimInit" ("stateEnum") T16."SimGoto" ("stateEnum") T16."SimFinish" ("stateEnum") T16."Wait" ("stateEnum")] -> w743
                                frame "INIT" {
                                }
                                frame "GOTO" {
                                }
                                frame "STOP" {
                                }
                                frame "NONE", Default {
                                }
                                }
                              }
                            }
                            n263 = Equal?(x=T16."Wait" ("stateEnum"), y=w721) -> (x = y?=w726:bool)
                            n264 = case shown="True" w726 {
                              tunnel: w725 -> [w730 w734]
                              tunnel: w724 -> [w729 w733]
                              tunnel: [w729 w732] -> w722
                              tunnel: [w730 w731] -> w723
                              frame False {
                              }
                              frame True {
                                n265 = call-dynamic "Clear ack flag.vi"("error in (no error)"=w733, "Motor in"=w734) -> ("error out"=w732:errorcluster, "Motor out"=w731:refnum<class "Motor.lvclass">)  [unwired: 8 in]
                              }
                            }
                          }
                        }
                      }
                      frame "ActiveInit" {
                        # "SEND INIT INSTRUCTIONS TO MOTOR"
                        n266 = call-dynamic "Get init instructions.vi"("error in (no error)"=w759, "Motor in"=w758) -> ("error out"=w760:errorcluster, "name"=w750:string, "init instructions"=w753:string[], "Motor out"=w757:refnum<class "Motor.lvclass">)  [unwired: 6 in]
                        n267 = local read "enabled log"() -> (w752:string)
                        n268 = call-dynamic "Send and log instructions.vi"("version"=w749, "current code"="2" ("current priority"), "enabled codes"=w752, "error in (no error)"=w760, "prefix"=w750, "instructions"=w753, "Motor in"=w757) -> ("error out"=w755:errorcluster, "replies"=w754:string[], "Motor out"=w756:refnum<class "Motor.lvclass">, "ok"=w764:bool)  [unwired: 1 out]
                        n269 = case shown="False" w764 {
                          tunnel: w755 -> [w778 w801]
                          tunnel: w756 -> [w779 w800]
                          tunnel: [w789 w795] -> w762
                          tunnel: [w788 w797] -> w763
                          tunnel: [T16."Wait" ("stateEnum") T16."ActiveUpdate" ("stateEnum")] -> w761
                          tunnel: w754 -> [w776 _]
                          tunnel: w753 -> [w775 _]
                          tunnel: w752 -> [w774 _]
                          tunnel: w749 -> [w770 _]
                          frame False {
                            w784 = ""
                            # "ERROR: CLEAR ACK FLAG IN ORDER TO ENABLE COMMANDS"
                            n270 = call-dynamic "Read name.vi"("error in (no error)"=w778, "Motor in"=w779) -> ("error out"=w783:errorcluster, "name"=w780:string, "Motor out"=w768:refnum<class "Motor.lvclass">)  [unwired: 7 in]
                            n271 = Concatenate Strings("COM ERROR ", w780, ": ActiveInit. Send Instructions, OK return fails.") -> (w769:string)
                            n272 = call-dynamic "Motor write log.vi"("prefix"=w769, "version"=w770, "current priority"="2", "enabled priority"=w774, "error in (no error)"=w783, "resp array"=w776, "send array"=w775, "Motor in"=w768) -> ("error out"=w777:errorcluster, "Motor out"=w767:refnum<class "Motor.lvclass">)  [unwired: 2 out]
                            n273 = Bundle By Name(cluster=T1 {"mode"="", "condition"="", "position"="", "pos_name"="", "pos_id"=""} ("status"), "mode"=w784, "condition"="NONE" ("x"), "position"=w784, "pos_name"=w784, "pos_id"=w784) -> (w785:T1)
                            n274 = call-dynamic "Write command in.vi"("error in (no error)"=w777, "command in"=T17 {"action"="", "param"="", "pos_name"="", "pos_idx"=0, "ack"=FALSE, "stop"=FALSE, "offset"=FALSE, "immediate"=FALSE, "instructions"=[]}, "Motor in"=w767) -> ("error out"=w786:errorcluster, "Motor out"=w787:refnum<class "Motor.lvclass">)  [unwired: 7 in]
                            n275 = call-dynamic "Write status.vi"("hold if empty"=TRUE, "error in (no error)"=w786, "status"=w785, "Motor in"=w787) -> ("error out"=w788:errorcluster, "Motor out"=w789:refnum<class "Motor.lvclass">)  [unwired: 6 in]
                          }
                          frame True {
                            w803 = ""
                            # "MOTOR RECEIVED INSTRUCTIONS: SET BUSY CONDITION"
                            n276 = Bundle By Name(cluster=T1 {"mode"="", "condition"="", "position"="", "pos_name"="", "pos_id"=""} ("status"), "mode"=w803, "condition"="BUSY" ("string"), "position"=w803, "pos_name"="NONE", "pos_id"="-1") -> (w804:T1)
                            n277 = call-dynamic "Write status.vi"("hold if empty"=TRUE, "error in (no error)"=w801, "status"=w804, "Motor in"=w800) -> ("error out"=w798:errorcluster, "Motor out"=w796:refnum<class "Motor.lvclass">)  [unwired: 6 in]
                            n278 = call-dynamic "Write moving flag.vi"("error in (no error)"=w798, "moving"=TRUE, "Motor in"=w796) -> ("error out"=w797:errorcluster, "Motor out"=w795:refnum<class "Motor.lvclass">)  [unwired: 7 in]
                          }
                        }
                      }
                      frame "ActiveGoto" {
                        # "SEND GOTO INSTRUCTIONS TO MOTOR"
                        n279 = call-dynamic "Get goto instructions.vi"("error in (no error)"=w815, "Motor in"=w816) -> ("error out"=w817:errorcluster, "name"=w809:string, "goto instructions"=w812:string[], "Motor out"=w818:refnum<class "Motor.lvclass">)  [unwired: 6 in]
                        n280 = local read "enabled log"() -> (w810:string)
                        n281 = call-dynamic "Send and log instructions.vi"("version"=w808, "current code"="2" ("current priority"), "enabled codes"=w810, "error in (no error)"=w817, "prefix"=w809, "instructions"=w812, "Motor in"=w818) -> ("error out"=w814:errorcluster, "replies"=w813:string[], "Motor out"=w822:refnum<class "Motor.lvclass">, "ok"=w823:bool)  [unwired: 1 out]
                        n282 = case shown="False" w823 {
                          tunnel: w814 -> [w842 w853]
                          tunnel: w822 -> [w841 w854]
                          tunnel: [w844 w858] -> w820
                          tunnel: [w843 w857] -> w821
                          tunnel: [T16."Wait" ("stateEnum") T16."ActiveUpdate" ("stateEnum")] -> w819
                          tunnel: w810 -> [w838 _]
                          tunnel: w813 -> [w836 _]
                          tunnel: w812 -> [w835 _]
                          tunnel: w808 -> [w829 _]
                          frame False {
                            w846 = ""
                            # "ERROR: CLEAR ACK FLAG IN ORDER TO ENABLE COMMANDS"
                            n283 = call-dynamic "Read name.vi"("error in (no error)"=w842, "Motor in"=w841) -> ("error out"=w840:errorcluster, "name"=w834:string, "Motor out"=w827:refnum<class "Motor.lvclass">)  [unwired: 7 in]
                            n284 = Concatenate Strings("COM ERROR ", w834, ": ActiveGoto. Send instructions, OK return fails. ") -> (w828:string)
                            n285 = call-dynamic "Motor write log.vi"("prefix"=w828, "version"=w829, "current priority"="0", "enabled priority"=w838, "error in (no error)"=w840, "resp array"=w836, "send array"=w835, "Motor in"=w827) -> ("error out"=w839:errorcluster, "Motor out"=w826:refnum<class "Motor.lvclass">)  [unwired: 2 out]
                            n286 = Bundle By Name(cluster=T1 {"mode"="", "condition"="", "position"="", "pos_name"="", "pos_id"=""} ("status"), "mode"=w846, "condition"="TIMEOUT" ("x"), "position"=w846, "pos_name"=w846, "pos_id"=w846) -> (w847:T1)
                            n287 = call-dynamic "Write command in.vi"("error in (no error)"=w839, "command in"=T17 {"action"="", "param"="", "pos_name"="", "pos_idx"=0, "ack"=FALSE, "stop"=FALSE, "offset"=FALSE, "immediate"=FALSE, "instructions"=[]}, "Motor in"=w826) -> ("error out"=w848:errorcluster, "Motor out"=w849:refnum<class "Motor.lvclass">)  [unwired: 7 in]
                            n288 = call-dynamic "Write status.vi"("hold if empty"=TRUE, "error in (no error)"=w848, "status"=w847, "Motor in"=w849) -> ("error out"=w843:errorcluster, "Motor out"=w844:refnum<class "Motor.lvclass">)  [unwired: 6 in]
                          }
                          frame True {
                            w855 = TRUE ("hold if empty")
                            w861 = ""
                            # "MOTOR RECEIVED INSTRUCTIONS: SET BUSY CONDITION"
                            n289 = Bundle By Name(cluster=T1 {"mode"="", "condition"="", "position"="", "pos_name"="", "pos_id"=""} ("status"), "mode"=w861, "condition"="BUSY" ("string"), "position"=w861, "pos_name"="NONE", "pos_id"="-1") -> (w862:T1)
                            n290 = call-dynamic "Write status.vi"("hold if empty"=w855, "error in (no error)"=w853, "status"=w862, "Motor in"=w854) -> ("error out"=w856:errorcluster, "Motor out"=w859:refnum<class "Motor.lvclass">)  [unwired: 6 in]
                            n291 = call-dynamic "Write moving flag.vi"("error in (no error)"=w856, "moving"=w855, "Motor in"=w859) -> ("error out"=w857:errorcluster, "Motor out"=w858:refnum<class "Motor.lvclass">)  [unwired: 7 in]
                          }
                        }
                      }
                      frame "ActiveStop" {
                        # "20240718"
                        n292 = call-dynamic "Read stop flag.vi"("error in (no error)"=w884, "Motor in"=w885) -> ("error out"=w875:errorcluster, "stop"=w883:bool, "Motor out"=w877:refnum<class "Motor.lvclass">)  [unwired: 7 in]
                        n293 = case shown="False" w883 {
                          tunnel: string[] ["STOP", "SR0=0"] ("instructions") -> [w890 w891]
                          tunnel: [w889 w891] -> w878
                          tunnel: "V46=251" -> [w888 _]
                          frame False {
                            # "STOP CMD WHILE\nMOTOR MOVING"
                            n294 = Insert Into Array(array=w890, new element=w888) -> (w889:string[])  [unwired: 1 in]
                          }
                          frame True {
                            # "STOP CMD WHILE\nMOTOR STATIC"
                          }
                        }
                        n295 = local read "enabled log"() -> (w872:string)
                        n296 = call-dynamic "Read name.vi"("error in (no error)"=w875, "Motor in"=w877) -> ("error out"=w874:errorcluster, "name"=w867:string, "Motor out"=w876:refnum<class "Motor.lvclass">)  [unwired: 7 in]
                        n297 = call-dynamic "Send and log instructions.vi"("version"=w866, "current code"="2" ("current priority"), "enabled codes"=w872, "error in (no error)"=w874, "prefix"=w867, "instructions"=w878, "Motor in"=w876) -> ("error out"=w879:errorcluster, "Motor out"=w881:refnum<class "Motor.lvclass">, "ok"=w869:bool)  [unwired: 2 out]
                        n298 = Select(t=T16."ActiveFinish" ("stateEnum"), s=w869, f=T16."ActiveStop" ("stateEnum")) -> (s? t:f=w868:T16)
                      }
                      frame "ActiveUpdate" {
                        n299 = local read "enabled log"() -> (w894:string)
                        n300 = call-dynamic "Get update instructions.vi"("error in (no error)"=w915, "only position"=FALSE, "Motor in"=w916) -> ("error out"=w911:errorcluster, "name"=w893:string, "read instructions"=w896:string[], "Motor out"=w910:refnum<class "Motor.lvclass">)  [unwired: 5 in]
                        n301 = call-dynamic "Send and log instructions.vi"("version"=w892, "current code"="5" ("current priority"), "enabled codes"=w894, "error in (no error)"=w911, "prefix"=w893, "instructions"=w896, "Motor in"=w910) -> ("error out"=w912:errorcluster, "error"=w907:bool, "replies"=w914:string[], "Motor out"=w913:refnum<class "Motor.lvclass">)  [unwired: 1 out]
                        n302 = case shown="False" w907 {
                          tunnel: w914 -> [w944 w981]
                          tunnel: w913 -> [w951 w971]
                          tunnel: w912 -> [w953 w980]
                          tunnel: [w925 w979] -> w906
                          tunnel: [w955 T16."ActiveUpdate" ("stateEnum")] -> w899
                          tunnel: [w926 w970] -> w898
                          tunnel: w896 -> [w943 w982]
                          tunnel: w893 -> [w938 w976]
                          tunnel: w894 -> [w940 _]
                          tunnel: w892 -> [w935 w973]
                          frame False {
                            # "PROCESS MOTOR RESPONSES"
                            n303 = Index Array(array=w944, index=1) -> (element=w952:string)
                            n304 = Index Array(array=w944, index=0) -> (element=w937:string)
                            n305 = call-dynamic "Encoder to mechanism position.vi"("error in (no error)"=w953, "motor position"=w952, "Motor in"=w951) -> ("error out"=w949:errorcluster, "mechanism position"=w942:string, "Motor out"=w950:refnum<class "Motor.lvclass">)  [unwired: 6 in]
                            n306 = Concatenate Strings("S4DMX ERROR ", w938, ": ActiveUpdate. Track code, error=1. ", w937) -> (w933:string)
                            n307 = call-dynamic "Write status position.vi"("error in (no error)"=w949, "status position"=w942, "Motor in"=w950) -> ("error out"=w930:errorcluster, "Motor out"=w932:refnum<class "Motor.lvclass">)  [unwired: 7 in]
                            n308 = Concatenate Strings(w938, "=" ("current priority"), w942) -> (w934:string)
                            n309 = call-dynamic "Motor write log.vi"("prefix"=w934, "version"=w935, "current priority"="5", "enabled priority"=w940, "error in (no error)"=w930, "Motor in"=w932) -> ("error out"=w929:errorcluster, "Motor out"=w931:refnum<class "Motor.lvclass">)  [unwired: 2 in, 2 out]
                            n310 = call-dynamic "Track movement.vi"("error in (no error)"=w929, "tracking code"=w937, "Motor in"=w931) -> ("error out"=w927:errorcluster, "error"=w946:bool, "moving"=w954:bool, "Motor out"=w928:refnum<class "Motor.lvclass">)  [unwired: 5 in]
                            n311 = Select(t=T16."ActiveUpdate" ("stateEnum"), s=w954, f=T16."ActiveFinish" ("stateEnum")) -> (s? t:f=w955:T16)
                            n312 = case shown="True" w946 {
                              tunnel: w940 -> [_ w969]
                              tunnel: w943 -> [_ w968]
                              tunnel: w944 -> [_ w967]
                              tunnel: w935 -> [_ w965]
                              tunnel: w933 -> [_ w964]
                              tunnel: w928 -> [w959 w963]
                              tunnel: w927 -> [w958 w960]
                              tunnel: [w959 w962] -> w926
                              tunnel: [w958 w961] -> w925
                              frame False {
                              }
                              frame True {
                                n313 = call-dynamic "Motor write log.vi"("prefix"=w964, "version"=w965, "current priority"="0", "enabled priority"=w969, "error in (no error)"=w960, "resp array"=w967, "send array"=w968, "Motor in"=w963) -> ("error out"=w961:errorcluster, "Motor out"=w962:refnum<class "Motor.lvclass">)  [unwired: 2 out]
                              }
                            }
                          }
                          frame True {
                            # "ERROR ON COMMUNICATION: TRY AGAIN"
                            n314 = local read "enabled log"() -> (w978:string)
                            n315 = Concatenate Strings("COM ERROR ", w976, ": ActiveUpdate. Send Instructions, error=1. ") -> (w972:string)
                            n316 = call-dynamic "Motor write log.vi"("prefix"=w972, "version"=w973, "current priority"="2", "enabled priority"=w978, "error in (no error)"=w980, "resp array"=w981, "send array"=w982, "Motor in"=w971) -> ("error out"=w979:errorcluster, "Motor out"=w970:refnum<class "Motor.lvclass">)  [unwired: 2 out]
                          }
                        }
                        n317 = call-dynamic "Read stop flag.vi"("error in (no error)"=w906, "Motor in"=w898) -> ("error out"=w903:errorcluster, "stop"=w905:bool, "Motor out"=w904:refnum<class "Motor.lvclass">)  [unwired: 7 in]
                        n318 = case shown="True" w905 {
                          tunnel: w904 -> [w919 w923]
                          tunnel: w903 -> [w918 w924]
                          tunnel: [w918 w922] -> w902
                          tunnel: [w919 w921] -> w901
                          tunnel: [w917 T16."ActiveStop" ("stateEnum")] -> w900
                          tunnel: w899 -> [w917 _]
                          frame False {
                          }
                          frame True {
                            n319 = call-dynamic "Clear stop flag.vi"("error in (no error)"=w924, "Motor in"=w923) -> ("error out"=w922:errorcluster, "Motor out"=w921:refnum<class "Motor.lvclass">)  [unwired: 8 in]
                          }
                        }
                      }
                      frame "ActiveFinish" {
                        w984 = "\t"
                        w1044 = ""
                        # "20240621"
                        # "TODO O CASE DEDERIA SER UM VI DA CLASSE MOTOR"
                        n320 = call-dynamic "Read command in.vi"("error in (no error)"=w1037, "Motor in"=w1036) -> ("error out"=w1003:errorcluster, "command in"=w1046:T17, "Motor out"=w1004:refnum<class "Motor.lvclass">)  [unwired: 6 in, 1 out]
                        n321 = call-dynamic "Read name.vi"("error in (no error)"=w1003, "Motor in"=w1004) -> ("error out"=w1001:errorcluster, "name"=w986:string, "Motor out"=w1002:refnum<class "Motor.lvclass">)  [unwired: 7 in]
                        n322 = call-dynamic "Read tracking code.vi"("error in (no error)"=w1001, "Motor in"=w1002) -> ("error out"=w999:errorcluster, "tracking code"=w1000:string, "Motor out"=w997:refnum<class "Motor.lvclass">)  [unwired: 7 in]
                        n323 = Unbundle By Name(w1046) -> ("action"=w1033:string, "pos_name"=w1023:string, "pos_idx"=w1043:i32, "stop"=w1045:bool)  [unwired: 2 out]
                        n324 = Equal?(x="INIT", y=w1033) -> (x = y?=w1031:bool)
                        n325 = Search and Replace String(input string=w1023, search string="L/" ("replace string (\"\")")) -> (offset past replacement=w1022:i32)  [unwired: 6 in, 3 out]
                        n326 = Equal?(x=w986, y="WPSEL" ("x")) -> (x = y?=w1020:bool)
                        n327 = Greater Or Equal To 0?(x=w1022) -> (x >= 0?=w1021:bool)
                        n328 = Number To Decimal String(number=w1043) -> (decimal integer string=w1042:string)  [unwired: 1 in]
                        n329 = Not Equal?(x="0", y=w1000) -> (x != y?=w1014:bool)
                        n330 = Select(t="NONE" ("condition"), s=w1031, f="TIMEOUT" ("condition")) -> (s? t:f=w1027:string)
                        n331 = And(x=w1020, y=w1021) -> (x .and. y?=w1019:bool)
                        n332 = case shown="False" w1045 {
                          tunnel: [w1068 "-1"] -> w1047
                          tunnel: [w1067 "NONE" ("pos_name")] -> w1048
                          tunnel: w1023 -> [w1070 _]
                          tunnel: [w1071 w1093] -> w1011
                          tunnel: w1042 -> [w1069 _]
                          tunnel: w1014 -> [w1066 _]
                          tunnel: w1027 -> [w1065 w1093]
                          tunnel: [w1064 w1095] -> w1013
                          tunnel: w1025 -> [w1063 w1095]
                          tunnel: w999 -> [w1062 w1094]
                          tunnel: [w1061 w1094] -> w1012
                          tunnel: w1019 -> [w1060 _]
                          frame False {
                            # "END OF MOVEMENT"
                            n333 = case shown="False" w1066 {
                              tunnel: [w1072 w1092] -> w1071
                              tunnel: w1070 -> [w1078 _]
                              tunnel: w1069 -> [w1079 _]
                              tunnel: [w1079 "-1" ("t")] -> w1068
                              tunnel: [w1078 "NONE" ("condition")] -> w1067
                              tunnel: w1065 -> [_ w1092]
                              tunnel: [w1074 w1089] -> w1064
                              tunnel: w1063 -> [w1077 w1089]
                              tunnel: w1062 -> [w1076 w1088]
                              tunnel: [w1073 w1088] -> w1061
                              tunnel: w1060 -> [w1075 _]
                              frame False {
                                # "NORMAL END"
                                n334 = case shown="False" w1075 {
                                tunnel: [w1082 w1087] -> w1074
                                tunnel: w1077 -> [w1082 w1086]
                                tunnel: w1076 -> [w1081 w1085]
                                tunnel: [w1081 w1084] -> w1073
                                tunnel: ["READY" ("condition") ""] -> w1072
                                frame False {
                                }
                                frame True {
                                n335 = call-dynamic "Add wprot init.vi"("error in (no error)"=w1085, "ICS in"=w1086) -> ("error out"=w1084:errorcluster, "ICS out"=w1087:refnum<class "ICS.lvclass">)  [unwired: 8 in]
                                }
                                }
                              }
                              frame True {
                                # "END WITH ERROR"
                              }
                            }
                          }
                          frame True {
                            # "FINISHED BY STOP COMMAND"
                          }
                        }
                        n336 = Equal?(x=w986, y="WPROT" ("x")) -> (x = y?=w1010:bool)
                        n337 = case shown="True" w1010 {
                          tunnel: [w1054 w1059] -> w1009
                          tunnel: w1013 -> [w1054 w1058]
                          tunnel: w1012 -> [w1053 w1057]
                          tunnel: w1011 -> [w1052 w1055]
                          tunnel: [w1053 w1056] -> w998
                          tunnel: [w1052 w1055] -> w1008
                          frame False {
                          }
                          frame True {
                            n338 = call-dynamic "Set wpsel ready.vi"("error in (no error)"=w1057, "ICS in"=w1058) -> ("error out"=w1056:errorcluster, "ICS out"=w1059:refnum<class "ICS.lvclass">)  [unwired: 8 in]
                          }
                        }
                        n339 = call-dynamic "Write commPriority.vi"("error in (no error)"=w998, "commPriority"=FALSE ("moving"), "Motor in"=w997) -> ("error out"=w1017:errorcluster, "Motor out"=w1018:refnum<class "Motor.lvclass">)  [unwired: 7 in]
                        n340 = call-dynamic "Write moving flag.vi"("error in (no error)"=w1017, "moving"=FALSE, "Motor in"=w1018) -> ("error out"=w1006:errorcluster, "Motor out"=w1007:refnum<class "Motor.lvclass">)  [unwired: 7 in]
                        n341 = call-dynamic "Write command in.vi"("error in (no error)"=w1006, "Motor in"=w1007) -> ("error out"=w1050:errorcluster, "Motor out"=w1049:refnum<class "Motor.lvclass">)  [unwired: 8 in]
                        n342 = call-dynamic "Clear ack flag.vi"("error in (no error)"=w1050, "Motor in"=w1049) -> ("error out"=w1040:errorcluster, "Motor out"=w1041:refnum<class "Motor.lvclass">)  [unwired: 8 in]
                        n343 = Bundle By Name(cluster=T1 {"mode"="", "condition"="", "position"="", "pos_name"="", "pos_id"=""} ("status"), "mode"=w1044, "condition"=w1008, "position"=w1044, "pos_name"=w1048, "pos_id"=w1047) -> (w1039:T1)
                        n344 = call-dynamic "Write status.vi"("hold if empty"=TRUE, "error in (no error)"=w1040, "status"=w1039, "Motor in"=w1041) -> ("error out"=w995:errorcluster, "Motor out"=w996:refnum<class "Motor.lvclass">)  [unwired: 6 in]
                        n345 = call-dynamic "Get status.vi"("error in (no error)"=w995, "Motor in"=w996) -> ("error out"=w990:errorcluster, "status string"=w987:string, "Motor out"=w991:refnum<class "Motor.lvclass">)  [unwired: 7 in]
                        n346 = Concatenate Strings(w986, w984, " Finish " ("current priority"), w984, w987) -> (w992:string)
                        n347 = call-dynamic "Motor write log.vi"("prefix"=w992, "version"=w993, "current priority"="6", "error in (no error)"=w990, "Motor in"=w991) -> ("error out"=w989:errorcluster, "Motor out"=w988:refnum<class "Motor.lvclass">)  [unwired: 3 in, 2 out]
                      }
                      frame "SimInit" {
                        w1112 = ""
                        n348 = local read "full init"() -> (w1103:bool)
                        n349 = case shown="False" w1103 {
                          tunnel: w1104 -> [w1132 w1160]
                          tunnel: w1105 -> [w1133 w1159]
                          tunnel: [w1137 w1153] -> w1117
                          tunnel: [w1136 w1152] -> w1116
                          tunnel: [w1135 w1150] -> w1115
                          frame True {
                            w1122 = 0 ("move index")
                            # "FULL INIT: SIMULATE ALL MOVEMENTS OF MECHANISM"
                            n350 = call-dynamic "Write moving flag.vi"("error in (no error)"=w1133, "moving"=TRUE, "Motor in"=w1132) -> ("error out"=w1131:errorcluster, "Motor out"=w1130:refnum<class "Motor.lvclass">)  [unwired: 7 in]
                            n351 = call <vilib>:"Space Constant.vi"() -> ("String"=w1140:string)
                            n352 = call-dynamic "Read MotorSim.vi"("error in (no error)"=w1131, "Motor in"=w1130) -> ("error out"=w1125:errorcluster, "MotorSim"=w1128:refnum<class "MotorSim.lvclass">, "Motor out"=w1137:refnum<class "Motor.lvclass">)  [unwired: 7 in]
                            n353 = Concatenate Strings("INIT" ("string"), w1140, "NONE" ("string")) -> (w1129:string)
                            n354 = call-dynamic "Write move index.vi"("error in (no error)"=w1125, "move index"=w1122, "MotorSim in"=w1128) -> ("error out"=w1124:errorcluster, "MotorSim out"=w1127:refnum<class "MotorSim.lvclass">)  [unwired: 7 in]
                            n355 = call-dynamic "Read movements.vi"("error in (no error)"=w1124, "index"=w1122, "MotorSim in"=w1127) -> ("error out"=w1123:errorcluster, "period"=w1120:u32, "initial position (0)"=w1121:i32, "MotorSim out"=w1126:refnum<class "MotorSim.lvclass">, "translation (100)"=w1119:i32, "forward"=w1118:bool)  [unwired: 3 in]
                            n356 = call-dynamic "Start movement.vi"("motor instructions"=w1129, "translation (100)"=w1119, "forward"=w1118, "error in (no error)"=w1123, "period"=w1120, "initial position (0)"=w1121, "MotorSim in"=w1126) -> ("error out"=w1135:errorcluster, "MotorSim out"=w1136:refnum<class "MotorSim.lvclass">)  [unwired: 3 in]
                          }
                          frame False {
                            # "FAST INIT: ONE DELAY ONLY IS DONE"
                            n357 = call-dynamic "Read max value.vi"("error in (no error)"=w1159, "Motor in"=w1160) -> ("error out"=w1148:errorcluster, "max value"=w1156:string, "Motor out"=w1147:refnum<class "Motor.lvclass">)  [unwired: 6 in, 1 out]
                            n358 = call <vilib>:"Space Constant.vi"() -> ("String"=w1161:string)
                            n359 = Fract/Exp String To Number(string=w1156) -> (number=w1141:dbl)  [unwired: 3 in, 1 out]
                            n360 = Random Number (0-1)() -> (number: 0 to 1=w1168:dbl)
                            n361 = Concatenate Strings("INIT" ("string"), w1161, "NONE" ("string")) -> (w1142:string)
                            n362 = call-dynamic "Write moving flag.vi"("error in (no error)"=w1148, "moving"=TRUE, "Motor in"=w1147) -> ("error out"=w1146:errorcluster, "Motor out"=w1145:refnum<class "Motor.lvclass">)  [unwired: 7 in]
                            n363 = Add(x=w1168, y=0.3) -> (x+y=w1166:dbl)
                            n364 = Divide(x=w1166, y=2.0) -> (x/y=w1162:dbl)
                            n365 = call-dynamic "Read MotorSim.vi"("error in (no error)"=w1146, "Motor in"=w1145) -> ("error out"=w1151:errorcluster, "MotorSim"=w1154:refnum<class "MotorSim.lvclass">, "Motor out"=w1153:refnum<class "Motor.lvclass">)  [unwired: 7 in]
                            n366 = Multiply(x=w1162, y=u32 12000 ("loopLimite")) -> (x*y=w1164:dbl)
                            n367 = Multiply(x=w1141, y=w1162) -> (x*y=w1169:dbl)
                            n368 = To Unsigned Long Integer(number=w1164) -> (unsigned 32bit integer=w1144:u32)
                            n369 = To Long Integer(number=w1169) -> (32bit integer=w1143:i32)
                            n370 = call-dynamic "Start movement.vi"("motor instructions"=w1142, "translation (100)"=w1143, "forward"=FALSE, "error in (no error)"=w1151, "period"=w1144, "initial position (0)"=w1143, "MotorSim in"=w1154) -> ("error out"=w1150:errorcluster, "MotorSim out"=w1152:refnum<class "MotorSim.lvclass">)  [unwired: 3 in]
                          }
                        }
                        n371 = call-dynamic "Write MotorSim.vi"("error in (no error)"=w1115, "MotorSim"=w1116, "Motor in"=w1117) -> ("error out"=w1111:errorcluster, "Motor out"=w1109:refnum<class "Motor.lvclass">)  [unwired: 7 in]
                        n372 = Bundle By Name(cluster=T1 {"mode"="", "condition"="", "position"="", "pos_name"="", "pos_id"=""} ("status"), "mode"=w1112, "condition"="BUSY" ("string"), "position"=w1112, "pos_name"="NONE", "pos_id"="-1") -> (w1107:T1)
                        n373 = call-dynamic "Write status.vi"("hold if empty"=TRUE, "error in (no error)"=w1111, "status"=w1107, "Motor in"=w1109) -> ("error out"=w1102:errorcluster, "Motor out"=w1101:refnum<class "Motor.lvclass">)  [unwired: 6 in]
                      }
                      frame "SimGoto" {
                        w1191 = ""
                        n374 = call-dynamic "Read command in.vi"("error in (no error)"=w1188, "Motor in"=w1187) -> ("error out"=w1178:errorcluster, "command in"=w1210:T17, "Motor out"=w1181:refnum<class "Motor.lvclass">)  [unwired: 6 in, 1 out]
                        n375 = Unbundle By Name(w1210) -> ("action"=w1209:string, "param"=w1177:string)
                        n376 = Fract/Exp String To Number(string=w1177) -> (number=w1176:dbl)  [unwired: 3 in, 1 out]
                        n377 = call-dynamic "Unit conversion.vi"("error in (no error)"=w1178, "To(T) or From(F) Encoder"=FALSE ("hold if empty"), "value in"=w1176, "Motor in"=w1181) -> ("error out"=w1179:errorcluster, "value out"=w1175:dbl, "Motor out"=w1180:refnum<class "Motor.lvclass">)  [unwired: 5 in]
                        n378 = call-dynamic "Read max value.vi"("error in (no error)"=w1179, "Motor in"=w1180) -> ("error out"=w1195:errorcluster, "max value"=w1224:string, "position"=w1208:string, "Motor out"=w1194:refnum<class "Motor.lvclass">)  [unwired: 6 in]
                        n379 = Fract/Exp String To Number(string=w1208, default (0 dbl)=0 ("default (0 DBL)")) -> (number=w1173:i32)  [unwired: 2 in, 1 out]
                        n380 = Fract/Exp String To Number(string=w1208) -> (number=w1206:dbl)  [unwired: 3 in, 1 out]
                        n381 = Fract/Exp String To Number(string=w1224) -> (number=w1205:dbl)  [unwired: 3 in, 1 out]
                        n382 = call <vilib>:"Space Constant.vi"() -> ("String"=w1213:string)
                        n383 = Subtract(x=w1206, y=w1175) -> (x-y=w1223:dbl)
                        n384 = Concatenate Strings(w1209, w1213, w1177) -> (w1201:string)
                        n385 = Divide(x=w1223, y=w1205) -> (x/y=w1222:dbl)
                        n386 = call-dynamic "Write moving flag.vi"("error in (no error)"=w1195, "moving"=TRUE, "Motor in"=w1194) -> ("error out"=w1193:errorcluster, "Motor out"=w1192:refnum<class "Motor.lvclass">)  [unwired: 7 in]
                        n387 = Absolute Value(x=w1223) -> (abs(x)=w1216:dbl)
                        n388 = Less Than 0?(x=w1223) -> (x < 0?=w1204:bool)
                        n389 = Multiply(x=w1222, y=u32 12000 ("loopLimite")) -> (x*y=w1219:dbl)
                        n390 = Absolute Value(x=w1219) -> (abs(x)=w1217:dbl)
                        n391 = To Long Integer(number=w1216) -> (32bit integer=w1172:i32)
                        n392 = call-dynamic "Read MotorSim.vi"("error in (no error)"=w1193, "Motor in"=w1192) -> ("error out"=w1202:errorcluster, "MotorSim"=w1203:refnum<class "MotorSim.lvclass">, "Motor out"=w1200:refnum<class "Motor.lvclass">)  [unwired: 7 in]
                        n393 = To Unsigned Long Integer(number=w1217) -> (unsigned 32bit integer=w1218:u32)
                        n394 = Add(x=u32 1000 ("loopLimite"), y=w1218) -> (x+y=w1171:u32)
                        n395 = call-dynamic "Start movement.vi"("motor instructions"=w1201, "translation (100)"=w1172, "forward"=w1204, "error in (no error)"=w1202, "period"=w1171, "initial position (0)"=w1173, "MotorSim in"=w1203) -> ("error out"=w1198:errorcluster, "MotorSim out"=w1199:refnum<class "MotorSim.lvclass">)  [unwired: 3 in]
                        n396 = call-dynamic "Write MotorSim.vi"("error in (no error)"=w1198, "MotorSim"=w1199, "Motor in"=w1200) -> ("error out"=w1211:errorcluster, "Motor out"=w1212:refnum<class "Motor.lvclass">)  [unwired: 7 in]
                        n397 = Bundle By Name(cluster=T1 {"mode"="", "condition"="", "position"="", "pos_name"="", "pos_id"=""} ("status"), "mode"=w1191, "condition"="BUSY" ("string"), "position"=w1191, "pos_name"="NONE", "pos_id"="-1") -> (w1197:T1)
                        n398 = call-dynamic "Write status.vi"("hold if empty"=TRUE, "error in (no error)"=w1211, "status"=w1197, "Motor in"=w1212) -> ("error out"=w1186:errorcluster, "Motor out"=w1185:refnum<class "Motor.lvclass">)  [unwired: 6 in]
                      }
                      frame "SimUptate" {
                        w1226 = T16."SimFinish" ("stateEnum")
                        n399 = call-dynamic "Read command in.vi"("error in (no error)"=w1236, "Motor in"=w1235) -> ("error out"=w1248:errorcluster, "command in"=w1247:T17, "Motor out"=w1249:refnum<class "Motor.lvclass">)  [unwired: 6 in, 1 out]
                        n400 = Unbundle By Name(w1247) -> ("stop"=w1246:bool)
                        n401 = call-dynamic "Read MotorSim.vi"("error in (no error)"=w1248, "Motor in"=w1249) -> ("error out"=w1253:errorcluster, "MotorSim"=w1254:refnum<class "MotorSim.lvclass">, "Motor out"=w1245:refnum<class "Motor.lvclass">)  [unwired: 7 in]
                        n402 = Select(t=w1226, s=w1246, f=T16."SimUptate" ("stateEnum")) -> (s? t:f=w1238:T16)
                        n403 = local read "full init"() -> (w1227:bool)
                        n404 = call-dynamic "Get position.vi"("error in (no error)"=w1253, "MotorSim in"=w1254) -> ("error out"=w1241:errorcluster, "end"=w1244:bool, "MotorSim out"=w1243:refnum<class "MotorSim.lvclass">, "current position"=w1242:string)  [unwired: 5 in, 1 out]
                        n405 = case shown="True" w1244 {
                          tunnel: w1243 -> [w1258 w1268]
                          tunnel: w1242 -> [w1256 w1266]
                          tunnel: w1241 -> [w1257 w1267]
                          tunnel: w1226 -> [_ w1263]
                          tunnel: [w1255 w1261] -> w1232
                          tunnel: [w1256 w1265] -> w1240
                          tunnel: [w1258 w1264] -> w1239
                          tunnel: [w1257 w1260] -> w1237
                          tunnel: w1238 -> [w1255 w1262]
                          tunnel: w1227 -> [_ w1259]
                          frame False {
                          }
                          frame True {
                            n406 = case shown="True" w1259 {
                              tunnel: w1268 -> [w1270 w1289]
                              tunnel: w1267 -> [w1271 w1276]
                              tunnel: w1266 -> [w1272 w1279]
                              tunnel: [w1272 w1278] -> w1265
                              tunnel: [w1271 w1273] -> w1260
                              tunnel: [w1270 w1280] -> w1264
                              tunnel: w1263 -> [w1269 w1277]
                              tunnel: w1262 -> [_ w1281]
                              tunnel: [w1269 w1282] -> w1261
                              frame False {
                              }
                              frame True {
                                n407 = call-dynamic "Read displacements.vi"("error in (no error)"=w1276, "MotorSim in"=w1289) -> ("error out"=w1275:errorcluster, "displacements"=w1287:T11, "MotorSim out"=w1288:refnum<class "MotorSim.lvclass">)  [unwired: 7 in]
                                n408 = call-dynamic "Read move index.vi"("error in (no error)"=w1275, "MotorSim in"=w1288) -> ("error out"=w1274:errorcluster, "move index"=w1286:i32, "MotorSim out"=w1290:refnum<class "MotorSim.lvclass">)  [unwired: 7 in]
                                n409 = Increment(x=w1286) -> (x+1=w1284:i32)
                                n410 = Array Size(array=w1287) -> (size(s)=w1285:i32)
                                n411 = Equal?(x=w1284, y=w1285) -> (x = y?=w1283:bool)
                                n412 = case shown="False" w1283 {
                                tunnel: w1274 -> [w1293 w1309]
                                tunnel: w1290 -> [w1306 w1310]
                                tunnel: w1284 -> [w1303 _]
                                tunnel: [T16."SimUptate" ("stateEnum") w1307] -> w1282
                                tunnel: w1281 -> [_ _]
                                tunnel: [w1299 w1310] -> w1280
                                tunnel: [w1301 w1309] -> w1273
                                tunnel: w1279 -> [_ w1308]
                                tunnel: [w1294 w1308] -> w1278
                                tunnel: w1277 -> [_ w1307]
                                frame False {
                                n413 = call-dynamic "Write move index.vi"("error in (no error)"=w1293, "move index"=w1303, "MotorSim in"=w1306) -> ("error out"=w1304:errorcluster, "MotorSim out"=w1305:refnum<class "MotorSim.lvclass">)  [unwired: 7 in]
                                n414 = call-dynamic "Read movements.vi"("error in (no error)"=w1304, "index"=w1303, "MotorSim in"=w1305) -> ("error out"=w1302:errorcluster, "period"=w1297:u32, "initial position (0)"=w1295:i32, "MotorSim out"=w1300:refnum<class "MotorSim.lvclass">, "translation (100)"=w1296:i32, "forward"=w1298:bool)  [unwired: 3 in]
                                n415 = call-dynamic "Start movement.vi"("translation (100)"=w1296, "forward"=w1298, "error in (no error)"=w1302, "period"=w1297, "initial position (0)"=w1295, "MotorSim in"=w1300) -> ("error out"=w1301:errorcluster, "MotorSim out"=w1299:refnum<class "MotorSim.lvclass">)  [unwired: 4 in]
                                n416 = Number To Fractional String(number=w1295, precision (6)=i16 3) -> (F-format string=w1294:string)  [unwired: 2 in]
                                }
                                frame True {
                                }
                                }
                              }
                            }
                          }
                        }
                        n417 = Bundle By Name(cluster=T1 {"mode"="", "condition"="", "position"="", "pos_name"="", "pos_id"=""} ("status"), "position"=w1240) -> (w1250:T1)
                        n418 = call-dynamic "Write MotorSim.vi"("error in (no error)"=w1237, "MotorSim"=w1239, "Motor in"=w1245) -> ("error out"=w1251:errorcluster, "Motor out"=w1252:refnum<class "Motor.lvclass">)  [unwired: 7 in]
                        n419 = call-dynamic "Write status.vi"("hold if empty"=TRUE, "error in (no error)"=w1251, "status"=w1250, "Motor in"=w1252) -> ("error out"=w1234:errorcluster, "Motor out"=w1233:refnum<class "Motor.lvclass">)  [unwired: 6 in]
                      }
                      frame "SimFinish" {
                        n420 = call-dynamic "Read command in.vi"("error in (no error)"=w1341, "Motor in"=w1340) -> ("error out"=w1324:errorcluster, "command in"=w1355:T17, "Motor out"=w1326:refnum<class "Motor.lvclass">)  [unwired: 6 in, 1 out]
                        n421 = Unbundle By Name(w1355) -> ("param"=w1328:string, "pos_name"=w1317:string, "pos_idx"=w1335:i32, "stop"=w1342:bool)  [unwired: 2 out]
                        n422 = call-dynamic "Read name.vi"("error in (no error)"=w1324, "Motor in"=w1326) -> ("error out"=w1315:errorcluster, "name"=w1323:string, "Motor out"=w1325:refnum<class "Motor.lvclass">)  [unwired: 7 in]
                        n423 = Equal?(x=w1323, y="WPSEL") -> (x = y?=w1321:bool)
                        n424 = call-dynamic "Encoder to mechanism position.vi"("error in (no error)"=w1315, "motor position"=w1328, "Motor in"=w1325) -> ("error out"=w1330:errorcluster, "mechanism position"=w1327:string, "Motor out"=w1329:refnum<class "Motor.lvclass">)  [unwired: 6 in]
                        n425 = Search and Replace String(input string=w1317, search string="L/" ("replace string (\"\")")) -> (offset past replacement=w1316:i32)  [unwired: 6 in, 3 out]
                        n426 = case shown="False" w1342 {
                          tunnel: [w1374 "-1"] -> w1347
                          tunnel: [w1368 "NONE" ("pos_name")] -> w1333
                          tunnel: w1335 -> [w1373 _]
                          tunnel: w1317 -> [w1368 _]
                          tunnel: [w1370 ""] -> w1332
                          tunnel: ["READY" ("condition") "TIMEOUT" ("pos_name")] -> w1331
                          tunnel: w1327 -> [w1371 _]
                          tunnel: w1321 -> [w1367 _]
                          tunnel: w1320 -> [w1363 w1382]
                          tunnel: [w1362 w1382] -> w1319
                          tunnel: w1316 -> [w1365 _]
                          tunnel: [w1361 w1381] -> w1314
                          tunnel: w1315 -> [w1360 w1381]
                          frame False {
                            # "END OF MOVEMENT"
                            n427 = Greater Or Equal To 0?(x=w1365) -> (x >= 0?=w1366:bool)
                            n428 = Search and Replace String(input string=w1371, search string="-") -> (result string=w1370:string)  [unwired: 6 in, 3 out]
                            n429 = Number To Decimal String(number=w1373) -> (decimal integer string=w1374:string)  [unwired: 1 in]
                            n430 = And(x=w1367, y=w1366) -> (x .and. y?=w1364:bool)
                            n431 = case shown="True" w1364 {
                              tunnel: w1363 -> [w1376 w1380]
                              tunnel: [w1376 w1379] -> w1362
                              tunnel: w1360 -> [w1375 w1378]
                              tunnel: [w1375 w1377] -> w1361
                              frame False {
                              }
                              frame True {
                                n432 = call-dynamic "Add wprot init.vi"("error in (no error)"=w1378, "ICS in"=w1380) -> ("error out"=w1377:errorcluster, "ICS out"=w1379:refnum<class "ICS.lvclass">)  [unwired: 8 in]
                              }
                            }
                          }
                          frame True {
                            # "FINISHED BY STOP COMMAND"
                          }
                        }
                        n433 = call-dynamic "Write moving flag.vi"("error in (no error)"=w1330, "moving"=FALSE, "Motor in"=w1329) -> ("error out"=w1349:errorcluster, "Motor out"=w1352:refnum<class "Motor.lvclass">)  [unwired: 7 in]
                        n434 = call-dynamic "Write command in.vi"("error in (no error)"=w1349, "Motor in"=w1352) -> ("error out"=w1350:errorcluster, "Motor out"=w1351:refnum<class "Motor.lvclass">)  [unwired: 8 in]
                        n435 = call-dynamic "Read MotorSim.vi"("error in (no error)"=w1350, "Motor in"=w1351) -> ("error out"=w1313:errorcluster, "MotorSim"=w1359:refnum<class "MotorSim.lvclass">, "Motor out"=w1358:refnum<class "Motor.lvclass">)  [unwired: 7 in]
                        n436 = Merge Errors(w1313, w1314) -> (w1312:errorcluster)
                        n437 = call-dynamic "Get position.vi"("error in (no error)"=w1312, "MotorSim in"=w1359) -> ("error out"=w1356:errorcluster, "MotorSim out"=w1357:refnum<class "MotorSim.lvclass">)  [unwired: 5 in, 3 out]
                        n438 = Bundle By Name(cluster=T1 {"mode"="", "condition"="", "position"="", "pos_name"="", "pos_id"=""} ("status"), "mode"="", "condition"=w1331, "position"=w1332, "pos_name"=w1333, "pos_id"=w1347) -> (w1354:T1)
                        n439 = call-dynamic "Write MotorSim.vi"("error in (no error)"=w1356, "MotorSim"=w1357, "Motor in"=w1358) -> ("error out"=w1346:errorcluster, "Motor out"=w1343:refnum<class "Motor.lvclass">)  [unwired: 7 in]
                        n440 = call-dynamic "Clear ack flag.vi"("error in (no error)"=w1346, "Motor in"=w1343) -> ("error out"=w1345:errorcluster, "Motor out"=w1344:refnum<class "Motor.lvclass">)  [unwired: 8 in]
                        n441 = call-dynamic "Write status.vi"("hold if empty"=TRUE, "error in (no error)"=w1345, "status"=w1354, "Motor in"=w1344) -> ("error out"=w1339:errorcluster, "Motor out"=w1338:refnum<class "Motor.lvclass">)  [unwired: 6 in]
                      }
                      frame "CyclicStart" {
                        w1406 = ""
                        n442 = call-dynamic "Read action-param.vi"("error in (no error)"=w1415, "Motor in"=w1416) -> ("error out"=w1414:errorcluster, "param"=w1412:string, "Motor out"=w1413:refnum<class "Motor.lvclass">)  [unwired: 6 in, 1 out]
                        n443 = local read "enabled log"() -> (w1393:string)
                        n444 = call-dynamic "Get cyclic instructions.vi"("error in (no error)"=w1414, "cyclic parameter"=w1412, "Motor in"=w1413) -> ("error out"=w1420:errorcluster, "start"=w1408:bool, "cyclic instructions"=w1394:string[], "Motor out"=w1421:refnum<class "Motor.lvclass">)  [unwired: 5 in]
                        n445 = Select(t=T16."CyclicUpdate" ("stateEnum"), s=w1408, f=T16."CyclicFinish" ("stateEnum")) -> (s? t:f=w1411:T16)
                        n446 = call-dynamic "Send instructions.vi"("error in (no error)"=w1420, "instructions"=w1394, "Motor in"=w1421) -> ("error out"=w1397:errorcluster, "replies"=w1395:string[], "Motor out"=w1388:refnum<class "Motor.lvclass">, "ok"=w1422:bool)  [unwired: 4 in, 1 out]
                        n447 = call-dynamic "Motor write log.vi"("prefix"="BUG ERROR. <Cyclic Start> ", "version"=w1390, "current priority"="0", "enabled priority"=w1393, "error in (no error)"=w1397, "resp array"=w1395, "send array"=w1394, "Motor in"=w1388) -> ("error out"=w1396:errorcluster, "Motor out"=w1387:refnum<class "Motor.lvclass">)  [unwired: 2 out]
                        n448 = case shown="False" w1422 {
                          tunnel: w1396 -> [w1429 w1438]
                          tunnel: w1387 -> [w1430 w1439]
                          tunnel: [w1426 w1442] -> w1402
                          tunnel: [w1425 w1441] -> w1401
                          tunnel: [T16."Wait" ("stateEnum") w1435] -> w1419
                          tunnel: w1411 -> [_ w1435]
                          tunnel: w1408 -> [_ w1434]
                          tunnel: [w1423 w1433] -> w1405
                          tunnel: [w1423 w1432] -> w1404
                          tunnel: ["TIMEOUT" ("string") "BUSY"] -> w1403
                          frame False {
                            w1423 = ""
                            # "ERROR: CLEAR COMMAND INPUT"
                            n449 = call-dynamic "Write command in.vi"("error in (no error)"=w1429, "command in"=T17 {"action"="", "param"="", "pos_name"="", "pos_idx"=0, "ack"=FALSE, "stop"=FALSE, "offset"=FALSE, "immediate"=FALSE, "instructions"=[]}, "Motor in"=w1430) -> ("error out"=w1425:errorcluster, "Motor out"=w1426:refnum<class "Motor.lvclass">)  [unwired: 7 in]
                          }
                          frame True {
                            # "MOTOR RECEIVED INSTRUCTIONS: SET BUSY CONDITION"
                            n450 = case shown="False" w1434 {
                              tunnel: [w1443 "NONE"] -> w1433
                              tunnel: [w1443 "-1"] -> w1432
                              frame False {
                                w1443 = ""
                              }
                              frame True {
                              }
                            }
                            n451 = call-dynamic "Write cyclic flag.vi"("error in (no error)"=w1438, "cyclic"=w1434, "Motor in"=w1439) -> ("error out"=w1436:errorcluster, "Motor out"=w1437:refnum<class "Motor.lvclass">)  [unwired: 7 in]
                            n452 = call-dynamic "Write moving flag.vi"("error in (no error)"=w1436, "moving"=TRUE ("hold if empty"), "Motor in"=w1437) -> ("error out"=w1441:errorcluster, "Motor out"=w1442:refnum<class "Motor.lvclass">)  [unwired: 7 in]
                          }
                        }
                        n453 = Bundle By Name(cluster=T1 {"mode"="", "condition"="", "position"="", "pos_name"="", "pos_id"=""} ("status"), "mode"=w1406, "condition"=w1403, "position"=w1406, "pos_name"=w1405, "pos_id"=w1404) -> (w1398:T1)
                        n454 = call-dynamic "Write status.vi"("hold if empty"=TRUE, "error in (no error)"=w1401, "status"=w1398, "Motor in"=w1402) -> ("error out"=w1399:errorcluster, "Motor out"=w1400:refnum<class "Motor.lvclass">)  [unwired: 6 in]
                      }
                      frame "CyclicUpdate" {
                        # "TO STOP PRG1 WITHOUT ANY WP MOVEMENT, ICS MUST WRITE V42=0 AND THEN INVERT AND RESTORE THE POLARITY OF DI2 INPUT (POL=2064 / POL=16)."
                        n455 = call-dynamic "Read stop flag.vi"("error in (no error)"=w1473, "Motor in"=w1474) -> ("error out"=w1463:errorcluster, "stop"=w1461:bool, "Motor out"=w1464:refnum<class "Motor.lvclass">)  [unwired: 7 in]
                        n456 = call-dynamic "Clear stop flag.vi"("error in (no error)"=w1463, "Motor in"=w1464) -> ("error out"=w1462:errorcluster, "Motor out"=w1465:refnum<class "Motor.lvclass">)  [unwired: 8 in]
                        n457 = disable-structure shown="Enabled" {
                          disable-tunnel: ["LTEX" "V31"] -> w1475
                          frame Disabled {
                          }
                          frame Enabled {
                          }
                        }
                        n458 = local read "enabled log"() -> (w1455:string)
                        n459 = Build Array("V42=0", "POL=2064", "POL=16") -> (w1468:string[])
                        n460 = Build Array(w1475) -> (w1472:string[])
                        n461 = Select(t=w1468, s=w1461, f=w1472) -> (s? t:f=w1452:string[])
                        n462 = Select(t=T16."CyclicFinish" ("stateEnum"), s=w1461, f=T16."CyclicUpdate" ("stateEnum")) -> (s? t:f=w1457:T16)
                        n463 = call-dynamic "Send instructions.vi"("error in (no error)"=w1462, "instructions"=w1452, "Motor in"=w1465) -> ("error out"=w1446:errorcluster, "replies"=w1453:string[], "Motor out"=w1449:refnum<class "Motor.lvclass">, "ok"=w1458:bool)  [unwired: 4 in, 1 out]
                        n464 = call-dynamic "Motor write log.vi"("prefix"="BUG ERROR. <Cyclic  Update> ", "version"=w1451, "current priority"="0", "enabled priority"=w1455, "error in (no error)"=w1446, "resp array"=w1453, "send array"=w1452, "Motor in"=w1449) -> ("error out"=w1447:errorcluster, "Motor out"=w1448:refnum<class "Motor.lvclass">)  [unwired: 2 out]
                        n465 = case shown="False" w1458 {
                          tunnel: w1453 -> [w1487 _]
                          tunnel: w1448 -> [w1481 w1503]
                          tunnel: w1447 -> [w1489 w1502]
                          tunnel: [w1490 w1493] -> w1466
                          tunnel: [w1480 w1492] -> w1467
                          tunnel: w1452 -> [w1488 w1505]
                          tunnel: w1457 -> [_ w1491]
                          tunnel: [T16."CyclicUpdate" ("stateEnum") w1491] -> w1456
                          tunnel: w1455 -> [w1484 _]
                          tunnel: w1451 -> [w1483 _]
                          frame False {
                            # "COMMUNICATION ERROR"
                            n466 = call-dynamic "Motor write log.vi"("prefix"="COM ERROR <Cyclic Update>. Send instructions, ok=0. ", "version"=w1483, "current priority"="1", "enabled priority"=w1484, "error in (no error)"=w1489, "resp array"=w1487, "send array"=w1488, "Motor in"=w1481) -> ("error out"=w1490:errorcluster, "Motor out"=w1480:refnum<class "Motor.lvclass">)  [unwired: 2 out]
                          }
                          frame True {
                            w1498 = ""
                            # "CORRECTION HAS NOT YET BEEN IMPLEMENTED."
                            # "CHECK AND CORRECT CYCLIC POSITION"
                            n467 = Index Array(array=w1505, index=0) -> (element=w1501:string)
                            n468 = call-dynamic "Read predef by index.vi"("error in (no error)"=w1502, "index"=w1501, "Motor in"=w1503) -> ("error out"=w1495:errorcluster, "pos_name"=w1500:string, "pos_value"=w1499:string, "Motor out"=w1496:refnum<class "Motor.lvclass">)  [unwired: 5 in]
                            n469 = Bundle By Name(cluster=T1 {"mode"="", "condition"="", "position"="", "pos_name"="", "pos_id"=""} ("status"), "mode"=w1498, "condition"=w1498, "position"=w1499, "pos_name"=w1500, "pos_id"=w1501) -> (w1494:T1)
                            n470 = call-dynamic "Write status.vi"("hold if empty"=TRUE, "error in (no error)"=w1495, "status"=w1494, "Motor in"=w1496) -> ("error out"=w1493:errorcluster, "Motor out"=w1492:refnum<class "Motor.lvclass">)  [unwired: 6 in]
                          }
                        }
                      }
                      frame "CyclicFinish" {
                        n471 = call-dynamic "Read cyclic flag.vi"("error in (no error)"=w1526, "Motor in"=w1527) -> ("error out"=w1524:errorcluster, "cyclic"=w1523:bool, "Motor out"=w1525:refnum<class "Motor.lvclass">)  [unwired: 7 in]
                        n472 = Build Array("V31", "SR1=0") -> (w1529:string[])
                        n473 = case shown="True" w1523 {
                          tunnel: w1529 -> [_ w1549]
                          tunnel: w1525 -> [w1536 w1554]
                          tunnel: w1524 -> [w1535 w1553]
                          tunnel: [w1536 w1552] -> w1515
                          tunnel: [w1535 w1547] -> w1514
                          tunnel: [w1534 w1551] -> w1513
                          tunnel: [T16."Wait" ("stateEnum") w1542] -> w1508
                          tunnel: w1507 -> [_ w1538]
                          frame False {
                            w1533 = ""
                            # "SINGLE OR SEVERAL OR U16 CYCLIC COMMAND WAS EXECUTED"
                            n474 = Bundle By Name(cluster=T1 {"mode"="", "condition"="", "position"="", "pos_name"="", "pos_id"=""} ("status"), "mode"=w1533, "condition"="READY", "position"=w1533, "pos_name"=w1533, "pos_id"=w1533) -> (w1534:T1)
                          }
                          frame True {
                            # "CYCLE ENABLED"
                            n475 = local read "enabled log"() -> (w1546:string)
                            n476 = call-dynamic "Send instructions.vi"("error in (no error)"=w1553, "instructions"=w1549, "Motor in"=w1554) -> ("error out"=w1545:errorcluster, "error"=w1550:bool, "replies"=w1548:string[], "Motor out"=w1540:refnum<class "Motor.lvclass">)  [unwired: 4 in, 1 out]
                            n477 = call-dynamic "Motor write log.vi"("prefix"="BUG ERROR.  <Cyclic Finish> ", "version"=w1538, "current priority"="1", "enabled priority"=w1546, "error in (no error)"=w1545, "resp array"=w1548, "send array"=w1549, "Motor in"=w1540) -> ("error out"=w1544:errorcluster, "Motor out"=w1539:refnum<class "Motor.lvclass">)  [unwired: 2 out]
                            n478 = case shown="False" w1550 {
                              tunnel: w1539 -> [w1571 w1596]
                              tunnel: w1544 -> [w1570 w1597]
                              tunnel: [w1557 w1597] -> w1547
                              tunnel: [w1556 w1596] -> w1552
                              tunnel: w1548 -> [w1568 _]
                              tunnel: [w1569 w1595] -> w1551
                              tunnel: [T16."Wait" ("stateEnum") T16."CyclicFinish" ("stateEnum")] -> w1542
                              frame False {
                                # "UPDATE WPROT STATUS"
                                n479 = Index Array(array=w1568, index=0) -> (element=w1562:string)
                                n480 = call-dynamic "Read predef by index.vi"("error in (no error)"=w1570, "index"=w1562, "Motor in"=w1571) -> ("error out"=w1558:errorcluster, "pos_name"=w1561:string, "pos_value"=w1566:string, "Motor out"=w1559:refnum<class "Motor.lvclass">)  [unwired: 5 in]
                                n481 = disable-structure shown="Enabled" {
                                disable-tunnel: [w1580 "READY" ("condition")] -> w1567
                                disable-tunnel: w1566 -> [w1575 w1591]
                                disable-tunnel: [_ w1591] -> w1565
                                disable-tunnel: [w1579 w1590] -> w1564
                                disable-tunnel: [w1578 w1589] -> w1563
                                disable-tunnel: w1562 -> [w1577 w1589]
                                disable-tunnel: w1561 -> [w1576 w1590]
                                frame Disabled {
                                n482 = case shown="False" {
                                selector: _ -> [_ _]
                                tunnel: w1575 -> [_ w1587]
                                tunnel: w1576 -> [_ w1588]
                                tunnel: ["NONE" ("x") w1588] -> w1579
                                tunnel: ["" w1587] -> _
                                tunnel: ["-1" ("x") w1586] -> w1578
                                tunnel: w1577 -> [_ w1586]
                                tunnel: ["TIMEOUT" ("x") "READY" ("condition")] -> w1580
                                frame False {
                                # "FAIL"
                                }
                                frame True {
                                # "OK"
                                }
                                }
                                }
                                frame Enabled {
                                }
                                }
                                n483 = Bundle By Name(cluster=T1 {"mode"="", "condition"="", "position"="", "pos_name"="", "pos_id"=""} ("status"), "mode"="", "condition"=w1567, "position"=w1565, "pos_name"=w1564, "pos_id"=w1563) -> (w1569:T1)
                                n484 = call-dynamic "Write cyclic flag.vi"("error in (no error)"=w1558, "cyclic"=FALSE, "Motor in"=w1559) -> ("error out"=w1557:errorcluster, "Motor out"=w1556:refnum<class "Motor.lvclass">)  [unwired: 7 in]
                              }
                              frame True {
                                w1593 = ""
                                # "RETRY"
                                n485 = Bundle By Name(cluster=T1 {"mode"="", "condition"="", "position"="", "pos_name"="", "pos_id"=""} ("status"), "mode"=w1593, "condition"=w1593, "position"=w1593, "pos_name"=w1593, "pos_id"=w1593) -> (w1595:T1)
                              }
                            }
                          }
                        }
                        n486 = call-dynamic "Write status.vi"("hold if empty"=TRUE, "error in (no error)"=w1514, "status"=w1513, "Motor in"=w1515) -> ("error out"=w1522:errorcluster, "Motor out"=w1521:refnum<class "Motor.lvclass">)  [unwired: 6 in]
                        n487 = call-dynamic "Write moving flag.vi"("error in (no error)"=w1522, "moving"=FALSE, "Motor in"=w1521) -> ("error out"=w1517:errorcluster, "Motor out"=w1518:refnum<class "Motor.lvclass">)  [unwired: 7 in]
                        n488 = call-dynamic "Write command in.vi"("error in (no error)"=w1517, "command in"=T17 {"action"="", "param"="", "pos_name"="", "pos_idx"=0, "ack"=FALSE, "stop"=FALSE, "offset"=FALSE, "immediate"=FALSE, "instructions"=[]}, "Motor in"=w1518) -> ("error out"=w1510:errorcluster, "Motor out"=w1528:refnum<class "Motor.lvclass">)  [unwired: 7 in]
                      }
                    }
                    n489 = call-dynamic "Write current state.vi"("error in (no error)"=w681, "currentState"=w678, "StateManager in"=w682) -> ("error out"=w692:errorcluster, "StateManager out"=w693:refnum<class "StateManager.lvclass">)  [unwired: 7 in]
                    n490 = call-dynamic "Write StateManager.vi"("error in (no error)"=w692, "StateManager"=w693, "Motor in"=w683) -> ("error out"=w690:errorcluster, "Motor out"=w689:refnum<class "Motor.lvclass">)  [unwired: 7 in]
                    n491 = call-dynamic "Write selected motor.vi"("error in (no error)"=w690, "Motor.lvclass"=w689, "ICS in"=w684) -> ("error out"=w688:errorcluster, "ICS out"=w691:refnum<class "ICS.lvclass">)  [unwired: 7 in]
                  }
                }
              }
              frame True {
                w1619 = "WPROT"
                # "20240718"
                # "VALID MESSAGE RECEIVED FROM CLIENT: VALIDATE & REPLY COMMAND"
                n492 = call-dynamic "Read motors.vi"("error in (no error)"=w1640, "ICS in"=w1639) -> ("error out"=w1637:errorcluster, "motors"=w1636:refnum<class "Motor.lvclass">[], "ICS out"=w1638:refnum<class "ICS.lvclass">)  [unwired: 7 in]
                n493 = case shown="True" w1635 {
                  tunnel: [w1740 w1749] -> w1641
                  tunnel: [w1741 w1748] -> w1630
                  tunnel: w1638 -> [w1741 w1748]
                  tunnel: w1637 -> [w1740 w1745]
                  tunnel: w1636 -> [w1742 w1746]
                  tunnel: [w1742 w1747] -> w1634
                  tunnel: [bool[] [] w1744] -> w1615
                  tunnel: w1613 -> [_ w1743]
                  frame False {
                  }
                  frame True {
                    n494 = for {
                      tunnel: w1746 -> [w1754] mode=indexing
                      tunnel: w1743 -> [w1753]
                      tunnel: w1745 -> [w1755]
                      tunnel: [w1752] -> w1749
                      tunnel: [w1751] -> w1747 mode=indexing
                      tunnel: [w1750] -> w1744 mode=indexing
                      n495 = call-dynamic "Validate command.vi"("error in (no error)"=w1755, "message"=w1753, "Motor in"=w1754) -> ("error out"=w1752:errorcluster, "ack"=w1750:bool, "Motor out"=w1751:refnum<class "Motor.lvclass">)  [unwired: 6 in]
                    }
                  }
                }
                n496 = for {
                  tunnel: w1634 -> [w1767] mode=indexing
                  shift-right: [w1759] -> w1599
                  shift-left: "" -> [w1758]
                  shift-right: [w1757] -> w1631
                  shift-left: w1641 -> [w1768]
                  tunnel: [w1756] -> w1629 mode=indexing
                  i -> [w1766]
                  # "CREATE STATUS MESSAGE"
                  n497 = Equal?(x=5, y=w1766) -> (x = y?=w1764:bool)
                  n498 = call-dynamic "Get status.vi"("error in (no error)"=w1768, "Motor in"=w1767) -> ("error out"=w1757:errorcluster, "status string"=w1760:string, "Motor out"=w1756:refnum<class "Motor.lvclass">)  [unwired: 7 in]
                  n499 = Select(t="\r\n", s=w1764, f=", ") -> (s? t:f=w1761:string)
                  n500 = Concatenate Strings(w1758, w1760, w1761) -> (w1759:string)
                }
                n501 = Boolean Array To Number(Boolean array=w1615) -> (number=w1614:u32)
                n502 = Not Equal To 0?(x=w1614) -> (x != 0?=w1609:bool)
                n503 = call-dynamic "Write motors.vi"("error in (no error)"=w1631, "motors"=w1629, "ICS in"=w1630) -> ("error out"=w1605:errorcluster, "ICS out"=w1603:refnum<class "ICS.lvclass">)  [unwired: 7 in]
                n504 = case shown="False" w1601 {
                  tunnel: [w1648 w1679] -> w1628
                  tunnel: [w1647 w1678] -> w1611
                  tunnel: w1599 -> [w1646 _]
                  tunnel: w1605 -> [w1645 w1678]
                  tunnel: w1603 -> [w1644 w1679]
                  tunnel: w1602 -> [w1643 _]
                  frame False {
                    # "NO COMMAND AT 0MQ PULL"
                    n505 = case shown="False" w1643 {
                      tunnel: [w1653 w1673] -> w1647
                      tunnel: w1645 -> [w1652 w1669]
                      tunnel: w1646 -> [w1651 w1677]
                      tunnel: [w1650 w1671] -> w1648
                      tunnel: w1644 -> [w1649 w1667]
                      frame False {
                        # "SEND STATUS TO CLIENT\nUSING INTERCOMM VI"
                        n506 = disable-structure shown="Enabled" {
                          disable-tunnel: [w1663 w1664] -> w1653
                          disable-tunnel: w1652 -> [w1658 w1664]
                          disable-tunnel: w1651 -> [w1662 _]
                          disable-tunnel: [w1661 w1665] -> w1650
                          disable-tunnel: w1649 -> [w1656 w1665]
                          frame Enabled {
                            n507 = call-dynamic "Read Messenger.vi"("error in (no error)"=w1658, "ICS in"=w1656) -> ("error out"=w1657:errorcluster, "Messenger.lvclass"=w1655:refnum<class "Messenger.lvclass">, "ICS out"=w1654:refnum<class "ICS.lvclass">)  [unwired: 7 in]
                            n508 = call-dynamic "Send status.vi"("error in (no error)"=w1657, "status"=w1662, "Messenger in"=w1655) -> ("error out"=w1660:errorcluster, "Messenger out"=w1659:refnum<class "Messenger.lvclass">)  [unwired: 7 in]
                            n509 = call-dynamic "Write Messenger.vi"("error in (no error)"=w1660, "Messenger.lvclass"=w1659, "ICS in"=w1654) -> ("error out"=w1663:errorcluster, "ICS out"=w1661:refnum<class "ICS.lvclass">)  [unwired: 7 in]
                          }
                          frame Disabled {
                          }
                        }
                      }
                      frame True {
                        # "SEND STATUS TO CLIENT\nUSING INNER TCP/IP CONNECTION"
                        n510 = call "Read Server.vi"("error in (no error)"=w1669, "ICS in"=w1667) -> ("error out"=w1668:errorcluster, "Server"=w1670:refnum<class "TCP-Server.lvclass">, "ICS out"=w1666:refnum<class "ICS.lvclass">)  [unwired: 7 in]
                        n511 = call-dynamic "Send message.vi"("error in (no error)"=w1668, "message"=w1677, "Server in"=w1670) -> ("error out"=w1676:errorcluster, "Server out"=w1675:refnum<class "TCP-Server.lvclass">)  [unwired: 7 in]
                        n512 = call-dynamic "Close connection.vi"("error in (no error)"=w1676, "Server in"=w1675) -> ("error out"=w1674:errorcluster, "Server out"=w1672:refnum<class "TCP-Server.lvclass">)  [unwired: 8 in]
                        n513 = call "Write Server.vi"("error in (no error)"=w1674, "Server"=w1672, "ICS in"=w1666) -> ("error out"=w1673:errorcluster, "ICS out"=w1671:refnum<class "ICS.lvclass">)  [unwired: 7 in]
                      }
                    }
                  }
                  frame True {
                    # "DO NOT SEND STATUS TO\nCLIENTS CONNECTED USING\nTCP/IP OR INTERCOMM.VI\n(NO CONNECTION TO THEM)"
                    # "THE COMMAND COMES FROM 0MQ PULL"
                  }
                }
                n514 = case shown="True" w1609 {
                  tunnel: w1613 -> [_ w1682]
                  tunnel: w1605 -> [w1680 w1687]
                  tunnel: [w1680 w1685] -> w1604
                  tunnel: w1599 -> [_ w1681]
                  frame False {
                  }
                  frame True {
                    # "20240718"
                    # "WRITE STATUS  & LOG CMD"
                    n515 = local read "enabled log"() -> (w1684:string)
                    n516 = local read "version"() -> (w1683:string)
                    n517 = call "Write log to file.vi"("prefix"=w1682, "version"=w1683, "current priority"="3", "enabled priority"=w1684, "error in"=w1687) -> ("error out"=w1686:errorcluster)  [unwired: 4 in, 2 out]
                    n518 = call "Write log to file.vi"("prefix"=w1681, "version"=w1683, "current priority"="4", "enabled priority"=w1684, "error in"=w1686) -> ("error out"=w1685:errorcluster)  [unwired: 4 in, 2 out]
                  }
                }
                n519 = call-dynamic "Read motor by name.vi"("error in (no error)"=w1611, "motor name"=w1619, "ICS in"=w1628) -> ("error out"=w1627:errorcluster, "Motor.lvclass"=w1626:refnum<class "Motor.lvclass">, "ICS out"=w1610:refnum<class "ICS.lvclass">)  [unwired: 5 in, 1 out]
                n520 = local read "enabled log"() -> (w1607:string)
                n521 = local read "version"() -> (w1600:string)
                n522 = call-dynamic "Read command in.vi"("error in (no error)"=w1627, "Motor in"=w1626) -> ("error out"=w1622:errorcluster, "command in"=w1625:T17, "Motor out"=w1621:refnum<class "Motor.lvclass">)  [unwired: 6 in, 1 out]
                n523 = Unbundle By Name(w1625) -> ("immediate"=w1624:bool, "instructions"=w1623:string[], "action"=w1618:string)
                n524 = Equal?(x=w1618, y="CYCLIC") -> (x = y?=w1616:bool)
                n525 = case shown="True" w1624 {
                  tunnel: w1623 -> [_ w1700]
                  tunnel: w1622 -> [w1690 w1710]
                  tunnel: w1621 -> [w1692 w1711]
                  tunnel: [w1690 w1699] -> w1606
                  tunnel: [w1692 w1706] -> w1620
                  tunnel: w1616 -> [_ w1701]
                  tunnel: [w1691 w1698] -> w1612
                  tunnel: w1610 -> [w1691 w1698]
                  tunnel: "<Immediate> " ("current priority") -> [_ w1694]
                  tunnel: w1607 -> [_ w1695]
                  tunnel: w1604 -> [_ _]
                  tunnel: w1600 -> [_ w1693]
                  frame False {
                  }
                  frame True {
                    n526 = call-dynamic "Send and log instructions.vi"("version"=w1693, "current code"="2" ("current priority"), "enabled codes"=w1695, "error in (no error)"=w1710, "prefix"=w1694, "instructions"=w1700, "Motor in"=w1711) -> ("error out"=w1697:errorcluster, "error"=w1709:bool, "Motor out"=w1708:refnum<class "Motor.lvclass">)  [unwired: 2 out]
                    n527 = Select(t=T16."CyclicUpdate" ("stateEnum"), s=w1701, f=T16."ActiveUpdate" ("stateEnum")) -> (s? t:f=w1702:T16)
                    n528 = case shown="False" w1709 {
                      tunnel: w1697 -> [w1732 w1738]
                      tunnel: w1708 -> [w1731 w1737]
                      tunnel: [w1714 w1738] -> w1707
                      tunnel: [w1716 w1737] -> w1705
                      tunnel: w1702 -> [w1718 _]
                      tunnel: w1701 -> [w1713 _]
                      frame False {
                        w1728 = ""
                        # "MANTER POS_NAME\nE POS_ID EM CYCLIC?"
                        n529 = call-dynamic "Read StateManager.vi"("error in (no error)"=w1732, "Motor in"=w1731) -> ("error out"=w1734:errorcluster, "StateManager"=w1733:refnum<class "StateManager.lvclass">, "Motor out"=w1730:refnum<class "Motor.lvclass">)  [unwired: 5 in, 2 out]
                        n530 = Bundle By Name(cluster=T1 {"mode"="", "condition"="", "position"="", "pos_name"="", "pos_id"=""} ("status"), "mode"=w1728, "condition"="BUSY" ("string"), "position"=w1728, "pos_name"="NONE", "pos_id"="-1") -> (w1721:T1)
                        n531 = call-dynamic "Write current state.vi"("error in (no error)"=w1734, "currentState"=w1718, "StateManager in"=w1733) -> ("error out"=w1735:errorcluster, "StateManager out"=w1736:refnum<class "StateManager.lvclass">)  [unwired: 7 in]
                        n532 = call-dynamic "Write StateManager.vi"("error in (no error)"=w1735, "StateManager"=w1736, "Motor in"=w1730) -> ("error out"=w1719:errorcluster, "Motor out"=w1720:refnum<class "Motor.lvclass">)  [unwired: 7 in]
                        n533 = call-dynamic "Write status.vi"("hold if empty"=TRUE, "error in (no error)"=w1719, "status"=w1721, "Motor in"=w1720) -> ("error out"=w1725:errorcluster, "Motor out"=w1724:refnum<class "Motor.lvclass">)  [unwired: 6 in]
                        n534 = call-dynamic "Write moving flag.vi"("error in (no error)"=w1725, "moving"=TRUE, "Motor in"=w1724) -> ("error out"=w1715:errorcluster, "Motor out"=w1717:refnum<class "Motor.lvclass">)  [unwired: 7 in]
                        n535 = call-dynamic "Write cyclic flag.vi"("error in (no error)"=w1715, "cyclic"=w1713, "Motor in"=w1717) -> ("error out"=w1714:errorcluster, "Motor out"=w1716:refnum<class "Motor.lvclass">)  [unwired: 7 in]
                      }
                      frame True {
                      }
                    }
                    n536 = call-dynamic "Clear immediate flag.vi"("error in (no error)"=w1707, "Motor in"=w1705) -> ("error out"=w1699:errorcluster, "Motor out"=w1706:refnum<class "Motor.lvclass">)  [unwired: 8 in]
                  }
                }
                n537 = call-dynamic "Write motor by name.vi"("error in (no error)"=w1606, "name"=w1619, "motor"=w1620, "ICS in"=w1612) -> ("error out"=w1632:errorcluster, "ICS out"=w1633:refnum<class "ICS.lvclass">)  [unwired: 6 in]
              }
            }
          }
        }
      }
      event "login help": Value Change {
        n538 = event-data() -> ()  [unwired: 1 in, 6 out]
        n539 = call "Help login.vi"() -> ()  [unwired: 12 in]
      }
      event "language": Value Change {
        n540 = event-data() -> ()  [unwired: 1 in, 6 out]
        n541 = control-ref of="check email"() -> (w1781:refnum<vi>)
        n542 = control-ref of="email ok"() -> (w1780:refnum<vi>)
        n543 = control-ref of="port"() -> (w1784:refnum<vi>)
        n544 = control-ref of="timeout"() -> (w1771:refnum<vi>)
        n545 = control-ref of="address"() -> (w1779:refnum<vi>)
        n546 = control-ref of="local IP 1"() -> (w1778:refnum<vi>)
        n547 = control-ref of="local IP 2"() -> (w1777:refnum<vi>)
        n548 = control-ref of="language"() -> (w1824:refnum<vi>)
        n549 = Build Array(w1781, w1780, w1779, w1784, w1771, w1778, w1777) -> (w1785:refnum<vi>[])
        n550 = control-ref of="server"() -> (w1826:refnum<vi>)
        n551 = control-ref of="exitLogin"() -> (w1825:refnum<vi>)
        n552 = control-ref of="login help"() -> (w1821:refnum<vi>)
        n553 = control-ref of="login"() -> (w1820:refnum<vi>)
        n554 = control-ref of="start server"() -> (w1817:refnum<vi>)
        n555 = control-ref of="exitStopped"() -> (w1816:refnum<vi>)
        n556 = control-ref of="assist"() -> (w1815:refnum<vi>)
        n557 = control-ref of="setup"() -> (w1814:refnum<vi>)
        n558 = control-ref of="control"() -> (w1813:refnum<vi>)
        n559 = control-ref of="loginUser"() -> (w1823:refnum<vi>)
        n560 = control-ref of="loginPW"() -> (w1822:refnum<vi>)
        n561 = Build Array(w1826, w1825, w1824, w1823, w1822, w1821, w1820, w1817, w1816, w1815, w1814, w1813) -> (w1819:refnum<vi>[])
        n562 = control-ref of="return assist"() -> (w1801:refnum<vi>)
        n563 = control-ref of="return control"() -> (w1800:refnum<vi>)
        n564 = control-ref of="logout stopped"() -> (w1812:refnum<vi>)
        n565 = control-ref of="stop server"() -> (w1811:refnum<vi>)
        n566 = control-ref of="logout running"() -> (w1810:refnum<vi>)
        n567 = control-ref of="save config"() -> (w1809:refnum<vi>)
        n568 = control-ref of="save as"() -> (w1808:refnum<vi>)
        n569 = control-ref of="config help"() -> (w1807:refnum<vi>)
        n570 = control-ref of="return setup"() -> (w1803:refnum<vi>)
        n571 = control-ref of="cfgFile"() -> (w1806:refnum<vi>)
        n572 = control-ref of="last cfg user"() -> (w1805:refnum<vi>)
        n573 = control-ref of="last cfg date"() -> (w1804:refnum<vi>)
        n574 = Build Array(w1812, w1811, w1810, w1809, w1808, w1807, w1806, w1805, w1804, w1803, w1801, w1800) -> (w1802:refnum<vi>[])
        n575 = Insert Into Array(array=w1819, new element=w1802) -> (w1786:refnum<vi>[])  [unwired: 1 in]
        n576 = Equal?(x="language", y=enum32{"PT", "EN", "NONE"}."NONE" ("language")) -> (x = y?=w1773:bool)
        n577 = Equal?(x="language", y=enum32{"PT", "EN", "NONE"}."PT" ("language")) -> (x = y?=w1772:bool)
        n578 = control-ref of="user permission"() -> (w1791:refnum<vi>)
        n579 = control-ref of="user previous"() -> (w1798:refnum<vi>)
        n580 = control-ref of="user next"() -> (w1787:refnum<vi>)
        n581 = control-ref of="user delete"() -> (w1788:refnum<vi>)
        n582 = control-ref of="user insert"() -> (w1790:refnum<vi>)
        n583 = control-ref of="change permission"() -> (w1792:refnum<vi>)
        n584 = control-ref of="email enable"() -> (w1794:refnum<vi>)
        n585 = control-ref of="auto logout"() -> (w1793:refnum<vi>)
        n586 = control-ref of="user name"() -> (w1789:refnum<vi>)
        n587 = control-ref of="email service"() -> (w1795:refnum<vi>)
        n588 = control-ref of="admin email"() -> (w1796:refnum<vi>)
        n589 = control-ref of="maint. email"() -> (w1797:refnum<vi>)
        n590 = Build Array(w1798, w1787, w1788, w1789, w1790, w1791, w1792, w1793, w1794, w1795, w1796, w1797) -> (w1799:refnum<vi>[])
        n591 = Insert Into Array(array=w1786, new element=w1799) -> (w1783:refnum<vi>[])  [unwired: 1 in]
        n592 = Insert Into Array(array=w1783, new element=w1785) -> (w1782:refnum<vi>[])  [unwired: 1 in]
        n593 = for {
          tunnel: w1782 -> [w1837] mode=indexing
          tunnel: "tips" -> [w1836] mode=indexing
          tunnel: w1772 -> [w1834]
          tunnel: w1773 -> [w1831]
          n594 = Unbundle By Name(w1836) -> ("PT"=w1833:string, "EN"=w1835:string)
          n595 = Select(t=w1833, s=w1834, f=w1835) -> (s? t:f=w1829:string)
          n596 = Select(t="", s=w1831, f=w1829) -> (s? t:f=w1832:string)
          n597 = property class="Ctl"(reference=w1837, "TipStrip"=w1832) -> ()  [unwired: 1 in, 2 out]
        }
      }
      event "comm help": Value Change {
        n598 = event-data() -> ()  [unwired: 1 in, 6 out]
        n599 = call "Help communication.vi"() -> ()  [unwired: 12 in]
      }
      event "login": Value Change {
        # "DO NOT OPEN\nPOPUP WHEN\nSERVER IS ON."
        n600 = event-data() -> ()  [unwired: 1 in, 3 out]
        n601 = local read "user list"() -> (w1849:T4)
        n602 = local read "server"() -> (w1846:bool)
        n603 = Not(x=w1846) -> (.not. x?=w1845:bool)
        n604 = call "Check id.vi"("password"="loginPW", "user name"="loginUser", "users in"=w1849) -> ("id ok"=w1853:bool, "first access"=w1844:bool, "users out"=w1842:T4, "permission"=w1857:string)  [unwired: 5 in]
        n605 = And(x=w1844, y=w1845) -> (x .and. y?=w1843:bool)
        n606 = case shown="False" w1843 {
          selector: w1843 -> [w1877 _]
          tunnel: "CONTINUE?" -> [_ w1881]
          tunnel: "Esta será sua senha\npermanente.\n\nYour password will\nbecome permanent." -> [_ w1880]
          tunnel: [w1878 w1879] -> w1852
          tunnel: w1853 -> [w1878 _]
          tunnel: [w1877 w1879] -> w1851
          frame False {
          }
          frame True {
            n607 = Two Button Dialog(message=w1880, 2:w1881) -> (T button?=w1879:bool)  [unwired: 1 in]
          }
        }
        n608 = case shown="True" w1851 {
          tunnel: w1841 -> [w1861 w1873]
          tunnel: [w1861 w1870] -> w1855
          tunnel: [w1860 w1869] -> w1854
          tunnel: w1840 -> [w1860 w1865]
          tunnel: w1842 -> [_ w1862]
          frame False {
            # "USER ALREADY HAS PASSWORD"
          }
          frame True {
            # "1st USER ACCESS: SAVE PASSWORD"
            n609 = local read "cfgFile"() -> (w1867:string)
            n610 = local write "user list"(w1862) -> ()
            n611 = call "Get attributes.vi"("error in (no error)"=w1865, "ICS in"=w1873) -> ("error out"=w1871:errorcluster, "email settings"=w1864:T10, "control indices"=w1872:i32[], "ICS out"=w1870:refnum<class "ICS.lvclass">)  [unwired: 6 in]
            n612 = call "Get date.vi"() -> ("date/time string"=w1863:string)  [unwired: 3 in]
            n613 = call <vilib>:"Application Directory.vi"() -> ("Application Directory"=w1868:path)
            n614 = Get Control Values by Index(1:w1872, 3:w1871) -> (10:w1874:variant[], 11:w1876:errorcluster)  [unwired: 1 in]
            n615 = Build Path(base path=w1868, name or relative path=w1867) -> (appended path=w1866:path)
            n616 = local write "last cfg date"(w1863) -> ()
            n617 = call "Config file.vi"("path"=w1866, "access (0:read/write)"=enum16{"read/write", "read-only", "write-only"}."write-only", "error in (no error)"=w1876, "data values"=w1874, "email settings"=w1864) -> ("error out"=w1869:errorcluster)  [unwired: 5 in, 1 out]
          }
        }
        n618 = case shown="True" w1852 {
          tunnel: w1857 -> [_ w1893]
          tunnel: w1855 -> [w1882 w1885]
          tunnel: [w1883 w1887] -> w1858
          tunnel: w1854 -> [w1883 w1888]
          tunnel: [w1882 w1886] -> w1859
          tunnel: "loginUser" -> [_ w1884]
          frame False {
            n619 = call <vilib>:"Beep.vi"() -> ()  [unwired: 12 in]
          }
          frame True {
            w1895 = T12."Disabled and Grayed Out" ("Disabled")
            w1896 = T12."Enabled" ("Disabled")
            # "USER CREDENTIALS ARE CORRECT"
            n620 = local read "server"() -> (w1906:bool)
            n621 = Equal?(x="Control", y=w1893) -> (x = y?=w1899:bool)
            n622 = Not Equal?(x=w1884, y="S4ICS") -> (x != y?=w1898:bool)
            n623 = Select(t=T6."Running" ("tab menu"), s=w1906, f=T6."Stopped" ("tab menu")) -> (s? t:f=w1903:T6)
            n624 = Equal?(x="Admin", y=w1893) -> (x = y?=w1907:bool)
            n625 = And(x=w1899, y=w1898) -> (x .and. y?=w1897:bool)
            n626 = call "Write current user.vi"("error in (no error)"=w1888, "current user"=w1884, "ICS in"=w1885) -> ("error out"=w1887:errorcluster, "ICS out"=w1886:refnum<class "ICS.lvclass">)  [unwired: 7 in]
            n627 = local write "tab menu"(w1903) -> ()
            n628 = local write "tab body"(enum32{"Motors", "Config"}."Motors" ("tab body")) -> ()
            n629 = Select(t=w1896, s=w1897, f=w1895) -> (s? t:f=w1908:T12)
            n630 = Select(t=w1896, s=w1907, f=w1895) -> (s? t:f=w1901:T12)
            n631 = Select(t=w1896, s=w1898, f=w1895) -> (s? t:f=w1900:T12)
            n632 = Build Array(0) -> (w1904:i32[])
            n633 = property on="setup" class="Bool"("DisabledEnum"=w1901) -> ()  [unwired: 2 in, 2 out]
            n634 = property on="control" class="Bool"("DisabledEnum"=w1908) -> ()  [unwired: 2 in, 2 out]
            n635 = property on="start server" class="Bool"("DisabledEnum"=w1900) -> ()  [unwired: 2 in, 2 out]
            n636 = property on="assist" class="Bool"("DisabledEnum"=w1900) -> ()  [unwired: 2 in, 2 out]
            n637 = property on="user list" class="Arr (strict)"("Index Values"=w1904) -> ()  [unwired: 2 in, 2 out]
          }
        }
      }
      event "logout running": Value Change {
        w1914 = ""
        n638 = event-data() -> ()  [unwired: 1 in, 6 out]
        n639 = local read "server"() -> (w1909:bool)
        n640 = local write "tab menu"(T6."Login" ("tab menu")) -> ()
        n641 = local write "tab body"(enum32{"Motors", "Config"}."Motors" ("tab body")) -> ()
        n642 = local write "loginPW"(w1914) -> ()
        n643 = local write "loginUser"(w1914) -> ()
        n644 = Not(x=w1909) -> (.not. x?=w1913:bool)
        n645 = property on="exitLogin" class="Bool"("Visible"=w1913) -> ()  [unwired: 2 in, 2 out]
        n646 = property on="loginUser" class="Str"("Key Focus"=TRUE) -> ()  [unwired: 2 in, 2 out]
      }
      event "logout stopped": Value Change {
        w1922 = ""
        n647 = event-data() -> ()  [unwired: 1 in, 6 out]
        n648 = local read "server"() -> (w1917:bool)
        n649 = local write "tab menu"(T6."Login" ("tab menu")) -> ()
        n650 = local write "tab body"(enum32{"Motors", "Config"}."Motors" ("tab body")) -> ()
        n651 = local write "loginPW"(w1922) -> ()
        n652 = local write "loginUser"(w1922) -> ()
        n653 = Not(x=w1917) -> (.not. x?=w1921:bool)
        n654 = property on="exitLogin" class="Bool"("Visible"=w1921) -> ()  [unwired: 2 in, 2 out]
        n655 = property on="loginUser" class="Str"("Key Focus"=TRUE) -> ()  [unwired: 2 in, 2 out]
      }
      event "stop server": Value Change {
        w1951 = FALSE
        w1950 = TRUE
        # "IF FIRST USER ACCESS (NO PASSWORD), RETURN TO LOGIN INSTEAD OF STOPPED MENU PAGE."
        n656 = event-data() -> ()  [unwired: 1 in, 1 out]
        n657 = local read "user list"() -> (w1958:T4)
        n658 = call "Read current user.vi"("error in (no error)"=w1959, "ICS in"=w1960) -> ("error out"=w1934:errorcluster, "current user"=w1957:string, "ICS out"=w1933:refnum<class "ICS.lvclass">)  [unwired: 7 in]
        n659 = property on="GFOC Value" class="DigNum (strict)"("Visible"=w1950) -> ()  [unwired: 2 in, 2 out]
        n660 = property on="WPROT Value" class="DigNum (strict)"("Visible"=w1950) -> ()  [unwired: 2 in, 2 out]
        n661 = property on="wprot stat" class="Clust (strict)"("Visible"=w1951) -> ()  [unwired: 2 in, 2 out]
        n662 = property on="wpsel stat" class="Clust (strict)"("Visible"=w1951) -> ()  [unwired: 2 in, 2 out]
        n663 = for {
          tunnel: w1958 -> [w2029] mode=indexing
          tunnel: w1957 -> [w2027]
          tunnel: [w2024] -> w1955
          stop <- w2023 stop-if-true
          n664 = Unbundle By Name(w2029) -> ("name"=w2028:string, "password"=w2026:string)  [unwired: 1 out]
          n665 = Equal?(x=w2028, y=w2027) -> (x = y?=w2023:bool)
          n666 = Empty String/Path?(string/path=w2026) -> (empty?=w2025:bool)
          n667 = And(x=w2025, y=w2023) -> (x .and. y?=w2024:bool)
        }
        n668 = property on="asel stat" class="Clust (strict)"("Visible"=w1951) -> ()  [unwired: 2 in, 2 out]
        n669 = property on="calw stat" class="Clust (strict)"("Visible"=w1951) -> ()  [unwired: 2 in, 2 out]
        n670 = property on="GMIR Value" class="DigNum (strict)"("Visible"=w1950) -> ()  [unwired: 2 in, 2 out]
        n671 = property on="WPSEL Value" class="DigNum (strict)"("Visible"=w1950) -> ()  [unwired: 2 in, 2 out]
        n672 = property on="gmir stat" class="Clust (strict)"("Visible"=w1951) -> ()  [unwired: 2 in, 2 out]
        n673 = property on="gfoc stat" class="Clust (strict)"("Visible"=w1951) -> ()  [unwired: 2 in, 2 out]
        n674 = call-dynamic "Read Messenger.vi"("error in (no error)"=w1934, "ICS in"=w1933) -> ("error out"=w1928:errorcluster, "Messenger.lvclass"=w1929:refnum<class "Messenger.lvclass">, "ICS out"=w1930:refnum<class "ICS.lvclass">)  [unwired: 7 in]
        n675 = property on="CALW Value" class="DigNum (strict)"("Visible"=w1950) -> ()  [unwired: 2 in, 2 out]
        n676 = property on="ASEL Value" class="DigNum (strict)"("Visible"=w1950) -> ()  [unwired: 2 in, 2 out]
        n677 = Select(t=T6."Login" ("tab menu"), s=w1955, f=T6."Stopped" ("tab menu")) -> (s? t:f=w1952:T6)
        n678 = disable-structure shown="Disabled" {
          disable-tunnel: w1930 -> [w1969 w1985]
          disable-tunnel: w1929 -> [w1968 w1986]
          disable-tunnel: w1928 -> [w1967 w1987]
          disable-tunnel: [w1966 w1985] -> w1927
          disable-tunnel: [w1964 w1986] -> w1926
          disable-tunnel: [w1963 w1987] -> w1925
          frame Disabled {
            n679 = flat-sequence {
              tunnel: w1969 -> [w1976]
              tunnel: w1968 -> [w1980]
              tunnel: w1967 -> [w1979]
              tunnel: T18 {"Message"="exit", "Message Data"=variant} ("message") -> [w1975]
              tunnel: [w1978] -> w1973
              tunnel: [w1977] -> w1972
              tunnel: [w1976] -> w1971
              tunnel: [u32 250 ("milliseconds to wait")] -> w1970
              tunnel: [w1982] -> w1966
              tunnel: [w1983] -> w1964
              tunnel: [w1984] -> w1963
              tunnel: w1973 -> [w1984]
              tunnel: w1972 -> [w1983]
              tunnel: w1971 -> [w1982]
              tunnel: w1970 -> [w1981]
              frame #0 {
                n680 = call-dynamic "Send message.vi"("error in (no error)"=w1979, "message"=w1975, "Messenger in"=w1980) -> ("error out"=w1978:errorcluster, "Messenger out"=w1977:refnum<class "Messenger.lvclass">)  [unwired: 7 in]
              }
              frame #1 {
                n681 = Wait (ms)(milliseconds to wait=w1981) -> ()  [unwired: 1 out]
              }
            }
          }
          frame Enabled {
            # "20240716"
          }
        }
        n682 = local write "tab menu"(w1952) -> ()
        n683 = local write "tab body"(enum32{"Motors", "Config"}."Motors" ("tab body")) -> ()
        n684 = local write "server"(FALSE) -> ()
        n685 = property on="login help" class="Bool"("DisabledEnum"=T12."Enabled" ("Disabled")) -> ()  [unwired: 2 in, 2 out]
        n686 = disable-structure shown="Enabled" {
          disable-tunnel: [w1993 w1995] -> w1932
          disable-tunnel: [w1992 w1994] -> w1931
          disable-tunnel: w1926 -> [w1991 w1994]
          disable-tunnel: w1925 -> [w1988 w1995]
          frame Disabled {
            n687 = call-dynamic "Destroy queues.vi"("error in (no error)"=w1988, "Messenger in"=w1991) -> ("error out"=w1989:errorcluster, "Messenger out"=w1990:refnum<class "Messenger.lvclass">)  [unwired: 8 in]
            n688 = call-dynamic "Stop 0mqComm.vi"("error in (no error)"=w1989, "Messenger in"=w1990) -> ("error out"=w1993:errorcluster, "Messenger out"=w1992:refnum<class "Messenger.lvclass">)  [unwired: 8 in]
          }
          frame Enabled {
            # "20240619"
          }
        }
        n689 = local read "channel"() -> (w1942:T5)
        n690 = Equal?(x=w1942, y=T5."Inner TCP/IP" ("channel")) -> (x = y?=w1941:bool)
        n691 = case shown="True" w1941 {
          tunnel: w1932 -> [w2001 w2014]
          tunnel: [w2000 w2012] -> w1938
          tunnel: [w1999 w2011] -> w1939
          tunnel: w1927 -> [w1998 w2013]
          tunnel: w1931 -> [w1997 w2010]
          tunnel: [w1996 w2010] -> w1935
          frame False {
            # "CLOSE INTERCOMM VI"
            n692 = disable-structure shown="Enabled" {
              disable-tunnel: w2001 -> [w2002 w2008]
              disable-tunnel: [w2005 w2008] -> w2000
              disable-tunnel: [w2006 w2009] -> w1999
              disable-tunnel: w1998 -> [w2006 w2009]
              disable-tunnel: w1997 -> [w2004 w2007]
              disable-tunnel: [w2003 w2007] -> w1996
              frame Enabled {
                n693 = call-dynamic "Stop InterComm.vi"("error in (no error)"=w2002, "Messenger in"=w2004) -> ("error out"=w2005:errorcluster, "Messenger out"=w2003:refnum<class "Messenger.lvclass">)  [unwired: 8 in]
              }
              frame Disabled {
              }
            }
          }
          frame True {
            # "CLOSE INNER TCP/IP CONNECTION"
            n694 = call "Read Server.vi"("error in (no error)"=w2014, "ICS in"=w2013) -> ("error out"=w2015:errorcluster, "Server"=w2017:refnum<class "TCP-Server.lvclass">, "ICS out"=w2011:refnum<class "ICS.lvclass">)  [unwired: 7 in]
            n695 = call "Read listenner.vi"("error in (no error)"=w2015, "Server in"=w2017) -> ("error out"=w2016:errorcluster, "listenner ID"=w2018:refnum<k5>)  [unwired: 7 in, 1 out]
            n696 = TCP Close Connection(connection ID=w2018, error in (no error)=w2016) -> (error out=w2012:errorcluster)  [unwired: 1 in, 1 out]
          }
        }
        n697 = call-dynamic "Write Messenger.vi"("error in (no error)"=w1938, "Messenger.lvclass"=w1935, "ICS in"=w1939) -> ("error out"=w1937:errorcluster, "ICS out"=w1936:refnum<class "ICS.lvclass">)  [unwired: 7 in]
        n698 = call-dynamic "Read motors.vi"("error in (no error)"=w1937, "ICS in"=w1936) -> ("error out"=w1949:errorcluster, "motors"=w1948:refnum<class "Motor.lvclass">[], "ICS out"=w1947:refnum<class "ICS.lvclass">)  [unwired: 7 in]
        n699 = for {
          tunnel: w1948 -> [w2019] mode=indexing
          tunnel: [w2020] -> w1945 mode=indexing
          shift-right: [w2021] -> w1946
          shift-left: w1949 -> [w2022]
          n700 = call-dynamic "Condition disabled to none.vi"("error in (no error)"=w2022, "Motor in"=w2019) -> ("error out"=w2021:errorcluster, "Motor out"=w2020:refnum<class "Motor.lvclass">)  [unwired: 8 in]
        }
        n701 = call-dynamic "Write motors.vi"("error in (no error)"=w1946, "motors"=w1945, "ICS in"=w1947) -> ("error out"=w1944:errorcluster, "ICS out"=w1943:refnum<class "ICS.lvclass">)  [unwired: 7 in]
      }
      event "start server": Value Change; User Event {
        # "IPs DIFERENTES ??\n\nDISABLED ??\n\nGFOC ??"
        n702 = event-data() -> ()  [unwired: 1 in, 3 out]
        n703 = local read "0mqEndpoint"() -> (w2065:string)
        n704 = local read "pubTime0mq"() -> (w2066:i32)
        n705 = call-dynamic "Read Messenger.vi"("error in (no error)"=w2082, "ICS in"=w2083) -> ("error out"=w2079:errorcluster, "Messenger.lvclass"=w2080:refnum<class "Messenger.lvclass">, "ICS out"=w2081:refnum<class "ICS.lvclass">)  [unwired: 7 in]
        n706 = Equal?(x="channel", y=T5."Inner TCP/IP" ("channel")) -> (x = y?=w2099:bool)
        n707 = local read "address"() -> (w2030:string)
        n708 = Bundle(cluster=T19 {"channel"=enum."Local Panel", "address"="", "port"=0, "timeout"=0} ("channel configuration"), "channel"="channel", "address"=w2065, "port"=u16 0, "timeout"=w2066) -> (w2067:T19)
        n709 = disable-structure shown="Enabled" {
          disable-tunnel: w2080 -> [w2128 w2130]
          disable-tunnel: w2079 -> [w2127 w2129]
          disable-tunnel: "timeout" -> [w2126 _]
          disable-tunnel: [w2124 w2130] -> w2069
          disable-tunnel: [w2123 w2129] -> w2068
          disable-tunnel: w2067 -> [w2121 _]
          frame Disabled {
            n710 = call-dynamic "Create queues.vi"("error in (no error)"=w2127, "timeout"=w2126, "Messenger in"=w2128) -> ("error out"=w2122:errorcluster, "Messenger out"=w2125:refnum<class "Messenger.lvclass">)  [unwired: 7 in]
            n711 = call-dynamic "Run 0mqComm.vi"("error in (no error)"=w2122, "show FP"=FALSE, "channel configuration"=w2121, "Messenger in"=w2125) -> ("error out"=w2123:errorcluster, "Messenger out"=w2124:refnum<class "Messenger.lvclass">)  [unwired: 6 in]
          }
          frame Enabled {
            # "20240619"
          }
        }
        n712 = case shown="True" w2099 {
          tunnel: w2081 -> [w2148 w2170]
          tunnel: w2068 -> [w2147 w2171]
          tunnel: [w2146 w2169] -> w2077
          tunnel: [w2145 w2172] -> w2076
          tunnel: w2030 -> [w2144 w2168]
          tunnel: "port" -> [w2143 w2167]
          tunnel: "timeout" -> [w2142 w2166]
          tunnel: "channel" -> [w2141 _]
          tunnel: w2069 -> [w2140 w2165]
          tunnel: [w2139 w2165] -> w2073
          frame False {
            # "START (RUN) INTERCOMM VI"
            n713 = disable-structure shown="Enabled" {
              disable-tunnel: w2148 -> [w2158 w2164]
              disable-tunnel: w2147 -> [w2156 w2163]
              disable-tunnel: [w2158 w2164] -> w2146
              disable-tunnel: [w2150 w2163] -> w2145
              disable-tunnel: w2144 -> [w2161 _]
              disable-tunnel: w2143 -> [w2160 _]
              disable-tunnel: w2142 -> [w2159 _]
              disable-tunnel: w2141 -> [w2154 _]
              disable-tunnel: w2140 -> [w2151 w2162]
              disable-tunnel: [w2149 w2162] -> w2139
              frame Enabled {
                n714 = Bundle(cluster=T19 {"channel"=enum."Local Panel", "address"="", "port"=0, "timeout"=0} ("channel configuration"), "channel"=w2154, "address"=w2161, "port"=w2160, "timeout"=w2159) -> (w2157:T19)
                n715 = Equal?(x=w2154, y=T5."Local Panel" ("channel")) -> (x = y?=w2152:bool)
                n716 = call-dynamic "Run InterComm.vi"("error in (no error)"=w2156, "show FP"=w2152, "channel configuration"=w2157, "Messenger in"=w2151) -> ("error out"=w2150:errorcluster, "Messenger out"=w2149:refnum<class "Messenger.lvclass">)  [unwired: 6 in]
              }
              frame Disabled {
              }
            }
          }
          frame True {
            # "CREATE LISTENNER FOR INNER TCP/IP CONNECTION"
            n717 = call "Read Server.vi"("error in (no error)"=w2171, "ICS in"=w2170) -> ("error out"=w2184:errorcluster, "Server"=w2185:refnum<class "TCP-Server.lvclass">, "ICS out"=w2183:refnum<class "ICS.lvclass">)  [unwired: 7 in]
            n718 = call "Write socket.vi"("ms timeout listening"=w2166, "error in (no error)"=w2184, "port"=w2167, "ip"=w2168, "Server in"=w2185) -> ("error out"=w2177:errorcluster, "Server out"=w2178:refnum<class "TCP-Server.lvclass">)  [unwired: 5 in]
            n719 = String To IP(1:w2168) -> (0:w2173:u32)
            n720 = call "Read timeouts.vi"("error in (no error)"=w2177, "Server in"=w2178) -> ("error out"=w2175:errorcluster, "ms create listener"=w2174:i32, "Server out"=w2176:refnum<class "TCP-Server.lvclass">)  [unwired: 4 in, 3 out]
            n721 = TCP Create Listener(7:w2173, 8:w2175, 9:w2174, 10:w2167) -> (0:w2182:errorcluster, 3:w2181:refnum<k5>)  [unwired: 1 in, 1 out]
            n722 = call "Write listenner.vi"("error in (no error)"=w2182, "listenner ID"=w2181, "Server in"=w2176) -> ("error out"=w2179:errorcluster, "Server out"=w2180:refnum<class "TCP-Server.lvclass">)  [unwired: 7 in]
            n723 = call "Write Server.vi"("error in (no error)"=w2179, "Server"=w2180, "ICS in"=w2183) -> ("error out"=w2172:errorcluster, "ICS out"=w2169:refnum<class "ICS.lvclass">)  [unwired: 7 in]
          }
        }
        n724 = local read "S4ICS password"() -> (w2115:string)
        n725 = local read "email service"() -> (w2113:string)
        n726 = local read "email enable"() -> (w2114:bool)
        n727 = local read "maint. email"() -> (w2119:string)
        n728 = local read "admin email"() -> (w2118:string)
        n729 = local read "S4ICS email"() -> (w2117:string)
        n730 = local read "S4ICS login"() -> (w2116:string)
        n731 = call-dynamic "Write Messenger.vi"("error in (no error)"=w2076, "Messenger.lvclass"=w2073, "ICS in"=w2077) -> ("error out"=w2074:errorcluster, "ICS out"=w2075:refnum<class "ICS.lvclass">)  [unwired: 7 in]
        n732 = local read "WPROT disabled"() -> (w2104:bool)
        n733 = local read "WPSEL disabled"() -> (w2105:bool)
        n734 = local read "CALW disabled"() -> (w2089:bool)
        n735 = local read "GMIR disabled"() -> (w2103:bool)
        n736 = local read "ASEL disabled"() -> (w2088:bool)
        n737 = Bundle By Name(cluster=T10 {"email service"="", "maint. email"="", "admin email"="", "S4ICS email"="", "S4ICS login"="", "S4ICS password"="", "email enabled"=FALSE} ("email cluster"), "email service"=w2113, "maint. email"=w2119, "admin email"=w2118, "S4ICS email"=w2117, "S4ICS login"=w2116, "S4ICS password"=w2115, "email enabled"=w2114) -> (w2094:T10)
        n738 = Build Array("WPROT mode", "WPSEL mode", "CALW mode", "ASEL mode", "GMIR mode", "GFOC mode") -> (w2092:string[])
        n739 = Build Array("WPROT ip", "WPSEL ip", "CALW ip", "ASEL ip", "GMIR ip", "GMIR ip") -> (w2093:string[])
        n740 = Build Array(w2104, w2105, w2089, w2088, w2103, w2103) -> (w2034:bool[])
        n741 = Build Array("WPROT positions", "WPSEL positions", "CALW positions", "ASEL positions", "GMIR positions", "GFOC positions") -> (w2035:cluster{"pos_name":string, "pos_value":dbl}[][])
        n742 = call-dynamic "Write configuration.vi"("predef positions"=w2035, "disabled flags"=w2034, "email settings"=w2094, "error in (no error)"=w2074, "setup ips"=w2093, "setup modes"=w2092, "ICS in"=w2075) -> ("error out"=w2062:errorcluster, "ICS out"=w2063:refnum<class "ICS.lvclass">)  [unwired: 3 in]
        n743 = call-dynamic "Read motors.vi"("error in (no error)"=w2062, "ICS in"=w2063) -> ("error out"=w2102:errorcluster, "motors"=w2084:refnum<class "Motor.lvclass">[], "ICS out"=w2097:refnum<class "ICS.lvclass">)  [unwired: 7 in]
        n744 = for {
          tunnel: w2084 -> [w2194] mode=indexing
          shift-right: [w2192] -> w2059
          shift-left: w2102 -> [w2187]
          tunnel: [w2193] -> w2101 mode=indexing
          shift-right: [w2190] -> w2060
          shift-left: TRUE -> [w2191]
          tunnel: [w2189] -> w2049 mode=indexing
          tunnel: [w2188] -> w2042 mode=indexing
          tunnel: w2034 -> [w2186] mode=indexing
          # "CHECK COMMUNICATION OF EACH MOTOR"
          n745 = case shown="False" w2186 {
            tunnel: w2194 -> [w2206 w2212]
            tunnel: [w2201 w2212] -> w2193
            tunnel: [w2200 w2213] -> w2192
            tunnel: w2191 -> [w2199 w2215]
            tunnel: [w2198 w2215] -> w2190
            tunnel: [w2197 T1 {"mode"="", "condition"="", "position"="", "pos_name"="", "pos_id"=""} ("wprot stat")] -> w2189
            tunnel: [w2196 FALSE] -> w2188
            tunnel: w2187 -> [w2195 w2213]
            frame False {
              w2207 = "2" ("current code")
              # "MECHANISM ENABLED"
              n746 = local read "enabled log"() -> (w2208:string)
              n747 = call-dynamic "Validate motor.vi"("current code"=w2207, "enabled codes"=w2208, "error in (no error)"=w2195, "Motor in"=w2206) -> ("error out"=w2209:errorcluster, "Motor out"=w2210:refnum<class "Motor.lvclass">)  [unwired: 6 in]
              n748 = call-dynamic "Send positions to motor.vi"("current code"=w2207, "enabled codes"=w2208, "error in (no error)"=w2209, "Motor in"=w2210) -> ("error out"=w2204:errorcluster, "Motor out"=w2205:refnum<class "Motor.lvclass">)  [unwired: 6 in]
              n749 = call-dynamic "Read active flag.vi"("error in (no error)"=w2204, "Motor in"=w2205) -> ("error out"=w2202:errorcluster, "active"=w2196:bool, "Motor out"=w2203:refnum<class "Motor.lvclass">)  [unwired: 7 in]
              n750 = call-dynamic "Read status.vi"("error in (no error)"=w2202, "Motor in"=w2203) -> ("error out"=w2200:errorcluster, "status"=w2197:T1, "Motor out"=w2201:refnum<class "Motor.lvclass">)  [unwired: 6 in, 1 out]
              n751 = And(x=w2196, y=w2199) -> (x .and. y?=w2198:bool)
            }
            frame True {
              # "MECHANISM DISABLED"
            }
          }
        }
        n752 = Not(x=w2060) -> (.not. x?=w2057:bool)
        n753 = Unbundle By Name(w2059) -> ("status"=w2058:bool)
        n754 = call-dynamic "Write motors.vi"("error in (no error)"=w2059, "motors"=w2101, "ICS in"=w2097) -> ("error out"=w2095:errorcluster, "ICS out"=w2096:refnum<class "ICS.lvclass">)  [unwired: 7 in]
        n755 = Index Array(array=w2049) -> (element #1=w2045:T1, element #2=w2046:T1, element #3=w2048:T1, element #4=w2047:T1, element #5=w2044:T1, element #6=w2043:T1)  [unwired: 6 in]
        n756 = Not Or(1:w2057, 2:w2058) -> (0:w2056:bool)
        n757 = case shown="True" w2056 {
          frame False {
          }
          frame True {
            w2136 = ""
            w2137 = FALSE
            w2138 = TRUE
            n758 = property on="GFOC Value" class="DigNum (strict)"("Visible"=w2137) -> ()  [unwired: 2 in, 2 out]
            n759 = property on="WPROT Value" class="DigNum (strict)"("Visible"=w2137) -> ()  [unwired: 2 in, 2 out]
            n760 = property on="wprot stat" class="Clust (strict)"("Visible"=w2138) -> ()  [unwired: 2 in, 2 out]
            n761 = property on="wpsel stat" class="Clust (strict)"("Visible"=w2138) -> ()  [unwired: 2 in, 2 out]
            n762 = property on="GMIR Value" class="DigNum (strict)"("Visible"=w2137) -> ()  [unwired: 2 in, 2 out]
            n763 = property on="WPSEL Value" class="DigNum (strict)"("Visible"=w2137) -> ()  [unwired: 2 in, 2 out]
            n764 = property on="asel stat" class="Clust (strict)"("Visible"=w2138) -> ()  [unwired: 2 in, 2 out]
            n765 = property on="calw stat" class="Clust (strict)"("Visible"=w2138) -> ()  [unwired: 2 in, 2 out]
            n766 = property on="CALW Value" class="DigNum (strict)"("Visible"=w2137) -> ()  [unwired: 2 in, 2 out]
            n767 = property on="ASEL Value" class="DigNum (strict)"("Visible"=w2137) -> ()  [unwired: 2 in, 2 out]
            n768 = property on="gmir stat" class="Clust (strict)"("Visible"=w2138) -> ()  [unwired: 2 in, 2 out]
            n769 = property on="gfoc stat" class="Clust (strict)"("Visible"=w2138) -> ()  [unwired: 2 in, 2 out]
            n770 = local write "loginPW"(w2136) -> ()
            n771 = local write "loginUser"(w2136) -> ()
            n772 = local write "tab menu"(T6."Login" ("tab menu")) -> ()
            n773 = local write "tab body"(enum32{"Motors", "Config"}."Motors" ("tab body")) -> ()
            n774 = property on="loginUser" class="Str"("Key Focus"=TRUE) -> ()  [unwired: 2 in, 2 out]
            n775 = property on="login help" class="Bool"("DisabledEnum"=T12."Disabled" ("Disabled")) -> ()  [unwired: 2 in, 2 out]
            n776 = property on="exitLogin" class="Bool"("Visible"=FALSE) -> ()  [unwired: 2 in, 2 out]
          }
        }
        n777 = Index Array(array=w2042) -> (element #1=w2038:bool, element #2=w2039:bool, element #3=w2041:bool, element #4=w2040:bool, element #5=w2037:bool, element #6=w2036:bool)  [unwired: 6 in]
        n778 = local write "server"(w2056) -> ()
        n779 = local write "wprot stat"(w2045) -> ()
        n780 = local write "wpsel stat"(w2046) -> ()
        n781 = local write "calw stat"(w2048) -> ()
        n782 = local write "asel stat"(w2047) -> ()
        n783 = local write "gmir stat"(w2044) -> ()
        n784 = local write "gfoc stat"(w2043) -> ()
        n785 = global write "Global Test.vi" "TX-RX"("TX-RXdelay") -> ()
        n786 = global write "Global Test.vi" "End"("Enddelay") -> ()
        n787 = local write "commWPROT"(w2038) -> ()
        n788 = local write "commWPSEL"(w2039) -> ()
        n789 = local write "commCALW"(w2041) -> ()
        n790 = local write "commASEL"(w2040) -> ()
        n791 = local write "commGMIR"(w2037) -> ()
        n792 = local write "commGFOC"(w2036) -> ()
        n793 = call <vilib>:"Clear Errors.vi"("error in (no error)"=w2095) -> ("error out"=w2033:errorcluster)  [unwired: 5 in, 1 out]
      }
      event "exitLogin": Value Change {
        w2224 = "exitLogin" ("Message")
        # "THE 0MQ MANAGER EXITS WHEN A EXIT MESSAGE IS READ FROM THE QUEUE"
        n794 = event-data() -> ()  [unwired: 1 in, 6 out]
        n795 = call-dynamic "Read Messenger.vi"("error in (no error)"=w2220, "ICS in"=w2221) -> ("error out"=w2231:errorcluster, "Messenger.lvclass"=w2230:refnum<class "Messenger.lvclass">, "ICS out"=w2226:refnum<class "ICS.lvclass">)  [unwired: 7 in]
        n796 = Bundle By Name(cluster=T18 {"Message"="", "Message Data"=variant} ("message"), "Message"="exit", "Message Data"=w2224) -> (w2229:T18)
        n797 = call-dynamic "Write last status.vi"("error in (no error)"=w2231, "last status"=w2224, "Messenger in"=w2230) -> ("error out"=w2227:errorcluster, "Messenger out"=w2228:refnum<class "Messenger.lvclass">)  [unwired: 7 in]
        n798 = call-dynamic "Send message.vi"("error in (no error)"=w2227, "message"=w2229, "Messenger in"=w2228) -> ("error out"=w2225:errorcluster, "Messenger out"=w2217:refnum<class "Messenger.lvclass">)  [unwired: 7 in]
        n799 = call-dynamic "Write Messenger.vi"("error in (no error)"=w2225, "Messenger.lvclass"=w2217, "ICS in"=w2226) -> ("error out"=w2219:errorcluster, "ICS out"=w2218:refnum<class "ICS.lvclass">)  [unwired: 7 in]
      }
      event "exitStopped": Value Change {
        w2238 = "exitStopped" ("Message")
        # "THE 0MQ MANAGER EXITS WHEN A EXIT MESSAGE IS READ FROM THE QUEUE"
        n800 = event-data() -> ()  [unwired: 1 in, 1 out]
        n801 = call-dynamic "Read Messenger.vi"("error in (no error)"=w2246, "ICS in"=w2247) -> ("error out"=w2245:errorcluster, "Messenger.lvclass"=w2244:refnum<class "Messenger.lvclass">, "ICS out"=w2237:refnum<class "ICS.lvclass">)  [unwired: 7 in]
        n802 = Bundle By Name(cluster=T18 {"Message"="", "Message Data"=variant} ("message"), "Message"="exit", "Message Data"=w2238) -> (w2241:T18)
        n803 = call-dynamic "Write last status.vi"("error in (no error)"=w2245, "last status"=w2238, "Messenger in"=w2244) -> ("error out"=w2239:errorcluster, "Messenger out"=w2240:refnum<class "Messenger.lvclass">)  [unwired: 7 in]
        n804 = call-dynamic "Send message.vi"("error in (no error)"=w2239, "message"=w2241, "Messenger in"=w2240) -> ("error out"=w2236:errorcluster, "Messenger out"=w2233:refnum<class "Messenger.lvclass">)  [unwired: 7 in]
        n805 = call-dynamic "Write Messenger.vi"("error in (no error)"=w2236, "Messenger.lvclass"=w2233, "ICS in"=w2237) -> ("error out"=w2235:errorcluster, "ICS out"=w2234:refnum<class "ICS.lvclass">)  [unwired: 7 in]
      }
      event "assist": Value Change {
        n806 = event-data() -> ()  [unwired: 1 in, 6 out]
        n807 = local write "tab menu"(T6."Assist" ("tab menu")) -> ()
        n808 = local write "tab body"(enum32{"Motors", "Config"}."Motors" ("tab body")) -> ()
      }
      event "return assist": Value Change {
        # "Set assist motor selector\nto \"No selection\".\nRequired by animation."
        n809 = event-data() -> ()  [unwired: 1 in, 6 out]
        n810 = call "Write motor IP.vi"("error in (no error)"=w2256, "motor IP"="", "ICS in"=w2255) -> ("error out"=w2254:errorcluster, "ICS out"=w2253:refnum<class "ICS.lvclass">)  [unwired: 7 in]
        n811 = local write "tab menu"(T6."Stopped" ("tab menu")) -> ()
        n812 = local write "tab body"(enum32{"Motors", "Config"}."Motors" ("tab body")) -> ()
      }
      event "setup": Value Change {
        n813 = event-data() -> ()  [unwired: 1 in, 6 out]
        n814 = stacked-sequence {
          frame #0 {
            # "SET TAB PAGES AND ADJUST CONTROLS"
            n815 = local write "user name"("") -> ()
            n816 = local write "email ok"(FALSE) -> ()
            n817 = local write "tab menu"(T6."Setup" ("tab menu")) -> ()
            n818 = local write "tab body"(enum32{"Motors", "Config"}."Config" ("tab body")) -> ()
            n819 = property on="email ok" class="Bool (strict)"("DisabledEnum"=T12."Disabled and Grayed Out" ("Disabled")) -> ()  [unwired: 2 in, 2 out]
          }
          frame #1 {
            # "DISABLE PM PWR CONTROLS BASED ON MAINS STATE"
            n820 = local read "pwrPM mains"() -> (w2269:bool)
            n821 = Select(t=T12."Disabled and Grayed Out" ("Disabled"), s=w2269, f=T12."Enabled" ("Disabled")) -> (s? t:f=w2268:T12)
            n822 = property on="pwrPM ip" class="Str"("DisabledEnum"=w2268) -> ()  [unwired: 2 in, 2 out]
            n823 = property on="pwrPM port" class="DigNum (strict)"("DisabledEnum"=w2268) -> ()  [unwired: 2 in, 2 out]
            n824 = property on="pwrPM user" class="Str"("DisabledEnum"=w2268) -> ()  [unwired: 2 in, 2 out]
            n825 = property on="pwrPM password" class="Str"("DisabledEnum"=w2268) -> ()  [unwired: 2 in, 2 out]
            n826 = property on="pwrPM outlet" class="DigNum (strict)"("DisabledEnum"=w2268) -> ()  [unwired: 2 in, 2 out]
          }
          frame #2 {
            # "DISABLE GD PWR CONTROLS BASED ON MAINS STATE"
            n827 = local read "pwrGD mains"() -> (w2273:bool)
            n828 = Select(t=T12."Disabled and Grayed Out" ("Disabled"), s=w2273, f=T12."Enabled" ("Disabled")) -> (s? t:f=w2272:T12)
            n829 = property on="pwrGD ip" class="Str"("DisabledEnum"=w2272) -> ()  [unwired: 2 in, 2 out]
            n830 = property on="pwrGD port" class="DigNum (strict)"("DisabledEnum"=w2272) -> ()  [unwired: 2 in, 2 out]
            n831 = property on="pwrGD user" class="Str"("DisabledEnum"=w2272) -> ()  [unwired: 2 in, 2 out]
            n832 = property on="pwrGD password" class="Str"("DisabledEnum"=w2272) -> ()  [unwired: 2 in, 2 out]
            n833 = property on="pwrGD outlet" class="DigNum (strict)"("DisabledEnum"=w2272) -> ()  [unwired: 2 in, 2 out]
          }
        }
      }
      event "save config": Value Change {
        n834 = event-data() -> ()  [unwired: 1 in, 6 out]
        n835 = local read "user list"() -> (w2281:T4)
        n836 = local read "last cfg date"() -> (w2286:string)
        n837 = local read "cfgFile"() -> (w2279:string)
        n838 = local read "last cfg user"() -> (w2285:string)
        n839 = call "Read current user.vi"("error in (no error)"=w2290, "ICS in"=w2289) -> ("error out"=w2283:errorcluster, "current user"=w2284:string, "ICS out"=w2288:refnum<class "ICS.lvclass">)  [unwired: 7 in]
        n840 = Empty String/Path?(string/path=w2279) -> (empty?=w2278:bool)
        n841 = call "Check admin.vi"("users in"=w2281) -> ("admin user?"=w2277:bool, "users out"=w2282:T4)  [unwired: 8 in, 1 out]
        n842 = case shown="False" w2278 {
          tunnel: w2279 -> [w2292 _]
          tunnel: [w2292 w2294] -> w2275
          tunnel: [TRUE ("valid name") w2293] -> w2274
          frame False {
          }
          frame True {
            n843 = call "Input name.vi"() -> ("file name"=w2294:string, "valid name"=w2293:bool)  [unwired: 9 in, 1 out]
          }
        }
        n844 = And(x=w2277, y=w2274) -> (x .and. y?=w2276:bool)
        n845 = case shown="True" w2276 {
          tunnel: [w2296 w2324] -> w2280
          tunnel: w2288 -> [w2297 w2315]
          tunnel: [w2297 w2322] -> w2287
          tunnel: w2282 -> [_ w2313]
          tunnel: w2286 -> [_ w2321]
          tunnel: w2285 -> [_ w2314]
          tunnel: w2284 -> [_ w2312]
          tunnel: w2283 -> [w2296 w2311]
          tunnel: w2275 -> [_ w2304]
          tunnel: w2274 -> [w2295 _]
          frame False {
            n846 = case shown="True" w2295 {
              frame False {
              }
              frame True {
                n847 = local read "language"() -> (w2303:enum32{"PT", "EN", "NONE"})
                n848 = Not Equal?(x=w2303, y=enum32{"PT", "EN", "NONE"}."EN" ("language")) -> (x != y?=w2302:bool)
                n849 = Select(t="É exigido um usuário (diferente\nde S4ICS) com a permissão Admin." ("message"), s=w2302, f="There must be at least one \nuser (other than S4ICS)\nwith Admin permission." ("message")) -> (s? t:f=w2301:string)
                n850 = One Button Dialog(message=w2301) -> ()  [unwired: 1 in, 1 out]
              }
            }
          }
          frame True {
            n851 = call "Get date.vi"() -> ("date/time string"=w2308:string)  [unwired: 3 in]
            n852 = flat-sequence {
              tunnel: w2311 -> [w2328]
              tunnel: w2308 -> [w2327]
              tunnel: [w2328] -> w2316
              tunnel: w2313 -> [w2325]
              tunnel: w2312 -> [w2326]
              frame #0 {
                n853 = local write "last cfg date"(w2327) -> ()
                n854 = local write "last cfg user"(w2326) -> ()
                n855 = local write "user list"(w2325) -> ()
              }
            }
            n856 = local write "cfgFile"(w2304) -> ()
            n857 = call "Get attributes.vi"("error in (no error)"=w2316, "ICS in"=w2315) -> ("error out"=w2323:errorcluster, "email settings"=w2310:T10, "control indices"=w2318:i32[], "ICS out"=w2320:refnum<class "ICS.lvclass">)  [unwired: 6 in]
            n858 = call <vilib>:"Application Directory.vi"() -> ("Application Directory"=w2307:path)
            n859 = Get Control Values by Index(1:w2318, 3:w2323) -> (10:w2317:variant[], 11:w2309:errorcluster)  [unwired: 1 in]
            n860 = Build Path(base path=w2307, name or relative path=w2304) -> (appended path=w2306:path)
            n861 = call "Config file.vi"("path"=w2306, "access (0:read/write)"=enum16{"read/write", "read-only", "write-only"}."write-only", "error in (no error)"=w2309, "data values"=w2317, "email settings"=w2310) -> ("error out"=w2305:errorcluster)  [unwired: 5 in, 1 out]
            n862 = case shown="No Error" w2305 {
              selector: w2305 -> [w2331 w2337]
              tunnel: w2320 -> [w2332 w2347]
              tunnel: [w2332 w2347] -> w2322
              tunnel: [w2331 w2346] -> w2324
              tunnel: w2321 -> [_ w2345]
              tunnel: w2314 -> [_ w2344]
              frame No Error {
                w2336 = ""
                # "WRITE ALL CONFIG PARAMETERS"
                n863 = local read "server"() -> (w2329:bool)
                n864 = local write "loginUser"(w2336) -> ()
                n865 = local write "loginPW"(w2336) -> ()
                n866 = property on="loginUser" class="Str"("Key Focus"=TRUE) -> ()  [unwired: 2 in, 2 out]
                n867 = local write "tab menu"(T6."Login" ("tab menu")) -> ()
                n868 = local write "tab body"(enum32{"Motors", "Config"}."Motors" ("tab body")) -> ()
                n869 = Not(x=w2329) -> (.not. x?=w2334:bool)
                n870 = property on="exitLogin" class="Bool"("Visible"=w2334) -> ()  [unwired: 2 in, 2 out]
              }
              frame Error {
                n871 = local read "language"() -> (w2343:enum32{"PT", "EN", "NONE"})
                n872 = local write "last cfg user"(w2344) -> ()
                n873 = local write "last cfg date"(w2345) -> ()
                n874 = Not Equal?(x=w2343, y=enum32{"PT", "EN", "NONE"}."EN" ("language")) -> (x != y?=w2342:bool)
                n875 = Select(t="Falha ao salvar\na configuração." ("message"), s=w2342, f="Can't write the\nconfiguration." ("message")) -> (s? t:f=w2339:string)
                n876 = call <vilib>:"Clear Errors.vi"("error in (no error)"=w2337) -> ("error out"=w2346:errorcluster)  [unwired: 5 in, 1 out]
                n877 = One Button Dialog(message=w2339) -> ()  [unwired: 1 in, 1 out]
              }
            }
          }
        }
      }
      event "save as": Value Change {
        n878 = event-data() -> ()  [unwired: 1 in, 6 out]
        n879 = call "Input name.vi"() -> ("file name"=w2348:string, "valid name"=w2349:bool)  [unwired: 9 in, 1 out]
        n880 = case shown="True" w2349 {
          tunnel: w2353 -> [w2354 w2365]
          tunnel: w2352 -> [w2355 w2364]
          tunnel: [w2355 w2363] -> w2351
          tunnel: [w2354 w2362] -> w2350
          tunnel: w2348 -> [_ w2356]
          frame False {
          }
          frame True {
            n881 = local read "user list"() -> (w2367:T4)
            n882 = local read "last cfg date"() -> (w2361:string)
            n883 = local read "last cfg user"() -> (w2360:string)
            n884 = call "Read current user.vi"("error in (no error)"=w2365, "ICS in"=w2364) -> ("error out"=w2357:errorcluster, "current user"=w2359:string, "ICS out"=w2368:refnum<class "ICS.lvclass">)  [unwired: 7 in]
            n885 = call "Check admin.vi"("users in"=w2367) -> ("admin user?"=w2369:bool, "users out"=w2366:T4)  [unwired: 8 in, 1 out]
            n886 = case shown="True" w2369 {
              tunnel: [w2370 w2387] -> w2362
              tunnel: w2368 -> [w2372 w2388]
              tunnel: [w2372 w2386] -> w2363
              tunnel: w2366 -> [_ w2378]
              tunnel: w2356 -> [_ w2381]
              tunnel: w2361 -> [_ w2383]
              tunnel: w2360 -> [_ w2382]
              tunnel: w2359 -> [_ w2379]
              tunnel: "%Y-%m-%d %H:%M:%S" ("time format string (%c)") -> [_ w2377]
              tunnel: w2357 -> [w2370 w2376]
              frame False {
                n887 = One Button Dialog(message="THERE MUST BE AT LEAST ONE \nUSER (OTHER THAN S4ICS)\nWITH ADMIN PERMISSION.") -> ()  [unwired: 1 in, 1 out]
              }
              frame True {
                n888 = Format Date/Time String(time format string (%c)=w2377) -> (date/time string=w2391:string)  [unwired: 2 in]
                n889 = flat-sequence {
                  tunnel: w2376 -> [w2398]
                  tunnel: w2391 -> [w2399]
                  tunnel: [w2398] -> w2389
                  tunnel: w2379 -> [w2397]
                  tunnel: w2378 -> [w2396]
                  frame #0 {
                    n890 = local write "last cfg date"(w2399) -> ()
                    n891 = local write "last cfg user"(w2397) -> ()
                    n892 = local write "user list"(w2396) -> ()
                  }
                }
                n893 = call "Get attributes.vi"("error in (no error)"=w2389, "ICS in"=w2388) -> ("error out"=w2393:errorcluster, "email settings"=w2375:T10, "control indices"=w2390:i32[], "ICS out"=w2386:refnum<class "ICS.lvclass">)  [unwired: 6 in]
                n894 = call <vilib>:"Application Directory.vi"() -> ("Application Directory"=w2385:path)
                n895 = Build Path(base path=w2385, name or relative path=w2381) -> (appended path=w2384:path)
                n896 = Get Control Values by Index(1:w2390, 3:w2393) -> (10:w2380:variant[], 11:w2374:errorcluster)  [unwired: 1 in]
                n897 = call "Config file.vi"("path"=w2384, "access (0:read/write)"=enum16{"read/write", "read-only", "write-only"}."write-only", "error in (no error)"=w2374, "data values"=w2380, "email settings"=w2375) -> ("error out"=w2373:errorcluster)  [unwired: 5 in, 1 out]
                n898 = case shown="No Error" w2373 {
                  selector: w2373 -> [w2404 w2412]
                  tunnel: [w2404 w2411] -> w2387
                  frame No Error {
                    n899 = property on="user list" class="Arr (strict)"() -> ("Index Values"=w2401:u32[])  [unwired: 2 in, 2 out]
                    n900 = Replace Array Subset(array=w2401, new element=u32 0 ("index")) -> (w2402:u32[])  [unwired: 1 in]
                    n901 = property on="save config" class="Bool"("DisabledEnum"=T12."Enabled" ("Disabled")) -> ()  [unwired: 2 in, 2 out]
                    n902 = property on="user list" class="Arr (strict)"("Index Values"=w2402) -> ()  [unwired: 2 in, 2 out]
                  }
                  frame Error {
                    n903 = local read "language"() -> (w2408:enum32{"PT", "EN", "NONE"})
                    n904 = Not Equal?(x=w2408, y=enum32{"PT", "EN", "NONE"}."EN" ("language")) -> (x != y?=w2406:bool)
                    n905 = Select(t="Falha ao salvar\na configuração." ("message"), s=w2406, f="Can't write the\nconfiguration." ("message")) -> (s? t:f=w2407:string)
                    n906 = call <vilib>:"Clear Errors.vi"("error in (no error)"=w2412) -> ("error out"=w2411:errorcluster)  [unwired: 5 in, 1 out]
                    n907 = One Button Dialog(message=w2407) -> ()  [unwired: 1 in, 1 out]
                  }
                }
                n908 = flat-sequence {
                  tunnel: w2383 -> [w2395]
                  tunnel: w2382 -> [w2394]
                  tunnel: w2373 -> [_]
                  frame #0 {
                    # "PUT LAST NAMES BACK"
                    n909 = local write "last cfg date"(w2395) -> ()
                    n910 = local write "last cfg user"(w2394) -> ()
                  }
                }
              }
            }
          }
        }
      }
      event "config help": Value Change {
        n911 = event-data() -> ()  [unwired: 1 in, 6 out]
        n912 = call "Help setup.vi"() -> ()  [unwired: 12 in]
      }
      event "log help": Value Change {
        n913 = event-data() -> ()  [unwired: 1 in, 6 out]
        n914 = call "Help logger.vi"() -> ()  [unwired: 12 in]
      }
      event "WPROT disabled": Value Change {
        # "THIS EVENT WILL BE USED TO TURN MOTOR POWER ON/OFF"
        n915 = event-data() -> ()  [unwired: 1 in, 6 out]
      }
      event "WPSEL disabled": Value Change {
        # "THIS EVENT WILL BE USED TO TURN MOTOR POWER ON/OFF"
        n916 = event-data() -> ()  [unwired: 1 in, 6 out]
      }
      event "ASEL disabled": Value Change {
        # "THIS EVENT WILL BE USED TO TURN MOTOR POWER ON/OFF"
        n917 = event-data() -> ()  [unwired: 1 in, 6 out]
      }
      event "CALW disabled": Value Change {
        # "THIS EVENT WILL BE USED TO TURN MOTOR POWER ON/OFF"
        n918 = event-data() -> ()  [unwired: 1 in, 6 out]
      }
      event "GMIR disabled": Value Change {
        # "THIS EVENT WILL BE USED TO TURN MOTOR POWER ON/OFF"
        n919 = event-data() -> ()  [unwired: 1 in, 6 out]
      }
      event "user next": Value Change {
        n920 = event-data() -> ()  [unwired: 1 in, 6 out]
        n921 = local read "user list"() -> (w2432:T4)
        n922 = property on="user list" class="Arr (strict)"() -> ("Index Values"=w2428:u32[])  [unwired: 2 in, 2 out]
        n923 = Index Array(array=w2428) -> (element=w2431:u32)  [unwired: 1 in]
        n924 = Array Size(array=w2432) -> (size(s)=w2430:i32)
        n925 = Increment(x=w2431) -> (x+1=w2427:u32)
        n926 = Less?(x=w2427, y=w2430) -> (x < y?=w2429:bool)
        n927 = case shown="True" w2429 {
          tunnel: w2428 -> [_ w2437]
          tunnel: w2427 -> [_ w2436]
          frame False {
          }
          frame True {
            # "INCREMENT USER LIST INDEX"
            n928 = Replace Array Subset(array=w2437, new element=w2436) -> (w2435:u32[])  [unwired: 1 in]
            n929 = property on="user list" class="Arr (strict)"("Index Values"=w2435) -> ()  [unwired: 2 in, 2 out]
          }
        }
      }
      event "user previous": Value Change {
        n930 = event-data() -> ()  [unwired: 1 in, 6 out]
        n931 = property on="user list" class="Arr (strict)"() -> ("Index Values"=w2439:u32[])  [unwired: 2 in, 2 out]
        n932 = Index Array(array=w2439) -> (element=w2441:u32)  [unwired: 1 in]
        n933 = Decrement(x=w2441) -> (x-1=w2438:u32)
        n934 = Greater Or Equal To 0?(x=w2438) -> (x >= 0?=w2440:bool)
        n935 = case shown="True" w2440 {
          tunnel: w2439 -> [_ w2446]
          tunnel: w2438 -> [_ w2444]
          frame False {
          }
          frame True {
            # "DECREMENT USER LIST INDEX"
            n936 = Replace Array Subset(array=w2446, new element=w2444) -> (w2445:u32[])  [unwired: 1 in]
            n937 = property on="user list" class="Arr (strict)"("Index Values"=w2445) -> ()  [unwired: 2 in, 2 out]
          }
        }
      }
      event "user delete": Value Change {
        w2450 = 0 ("index")
        n938 = event-data() -> ()  [unwired: 1 in, 6 out]
        n939 = call "Read current user.vi"("error in (no error)"=w2462, "ICS in"=w2461) -> ("error out"=w2463:errorcluster, "current user"=w2447:string, "ICS out"=w2459:refnum<class "ICS.lvclass">)  [unwired: 7 in]
        n940 = local read "user list"() -> (w2457:T4)
        n941 = property on="user list" class="Arr (strict)"() -> ("Index Values"=w2451:u32[])  [unwired: 2 in, 2 out]
        n942 = local read "language"() -> (w2456:enum32{"PT", "EN", "NONE"})
        n943 = Index Array(array=w2451, index=w2450) -> (element=w2453:u32)
        n944 = Decrement(x=w2453) -> (x-1=w2452:u32)
        n945 = Index Array(array=w2457, index=w2453) -> (element=w2460:T20)
        n946 = Not Equal?(x=w2456, y=enum32{"PT", "EN", "NONE"}."EN" ("language")) -> (x != y?=w2455:bool)
        n947 = Unbundle By Name(w2460) -> ("name"=w2448:string)
        n948 = Replace Array Subset(array=w2451, new element=w2452, index=w2450) -> (w2449:u32[])
        n949 = Equal?(x=w2448, y=w2447) -> (x = y?=w2458:bool)
        n950 = case shown="False" w2458 {
          tunnel: w2457 -> [w2472 _]
          tunnel: w2453 -> [w2473 _]
          tunnel: w2448 -> [w2469 _]
          tunnel: w2455 -> [w2465 w2489]
          tunnel: w2449 -> [w2464 _]
          frame False {
            n951 = Concatenate Strings("O usuário \"", w2469, "\" será removido.\nContinuar?") -> (w2467:string)
            n952 = Concatenate Strings("The user \"", w2469, "\" will be removed.\nAre you sure?") -> (w2468:string)
            n953 = Select(t=w2467, s=w2465, f=w2468) -> (s? t:f=w2466:string)
            n954 = Two Button Dialog(message=w2466) -> (T button?=w2474:bool)  [unwired: 2 in]
            n955 = case shown="True" w2474 {
              tunnel: w2473 -> [_ w2480]
              tunnel: w2472 -> [_ w2479]
              tunnel: w2464 -> [_ w2478]
              frame False {
              }
              frame True {
                n956 = flat-sequence {
                  tunnel: w2480 -> [w2482]
                  tunnel: w2479 -> [w2484]
                  tunnel: w2478 -> [w2481]
                  tunnel: [w2481] -> w2477
                  tunnel: w2477 -> [w2485]
                  frame #0 {
                    n957 = Delete From Array(array=w2484, index=w2482) -> (array with subset deleted=w2483:T4)  [unwired: 1 in, 1 out]
                    n958 = local write "user list"(w2483) -> ()
                  }
                  frame #1 {
                    n959 = property on="user list" class="Arr (strict)"("Index Values"=w2485) -> ()  [unwired: 2 in, 2 out]
                  }
                }
              }
            }
          }
          frame True {
            n960 = Select(t="A auto-remoção não é permitida." ("message"), s=w2489, f="You can't delete yourself. " ("message")) -> (s? t:f=w2487:string)
            n961 = One Button Dialog(message=w2487) -> ()  [unwired: 1 in, 1 out]
          }
        }
      }
      event "change permission": Value Change {
        n962 = event-data() -> ()  [unwired: 1 in, 6 out]
        n963 = call "Read current user.vi"("error in (no error)"=w2510, "ICS in"=w2509) -> ("error out"=w2508:errorcluster, "current user"=w2490:string, "ICS out"=w2506:refnum<class "ICS.lvclass">)  [unwired: 7 in]
        n964 = local read "user list"() -> (w2501:T4)
        n965 = for {
          tunnel: w2501 -> [w2518] mode=indexing
          shift-right: [w2517] -> w2497
          shift-left: 0 ("index") -> [w2515]
          n966 = Unbundle By Name(w2518) -> ("permission"=w2513:string)
          n967 = Equal?(x="Admin", y=w2513) -> (x = y?=w2516:bool)
          n968 = Increment(x=w2515) -> (x+1=w2514:i32)
          n969 = Select(t=w2514, s=w2516, f=w2515) -> (s? t:f=w2517:i32)
        }
        n970 = property on="user list" class="Arr (strict)"() -> ("Index Values"=w2505:u32[])  [unwired: 2 in, 2 out]
        n971 = local read "user permission"() -> (w2491:string)
        n972 = Index Array(array=w2505, index=0) -> (element=w2507:u32)
        n973 = Index Array(array=w2501, index=w2507) -> (element=w2504:T20)
        n974 = Unbundle By Name(w2504) -> ("name"=w2503:string, "password"=w2502:string)  [unwired: 1 out]
        n975 = Greater?(x=w2497, y=u32 1) -> (0:w2495:bool)
        n976 = Equal?(x=w2503, y=w2490) -> (x = y?=w2492:bool)
        n977 = Equal?(x=w2491, y="Admin") -> (x = y?=w2496:bool)
        n978 = And(x=w2496, y=w2495) -> (x .and. y?=w2494:bool)
        n979 = Or(x=w2494, y=w2492) -> (x .or. y?=w2493:bool)
        n980 = case shown="True" w2493 {
          tunnel: w2504 -> [w2523 _]
          tunnel: w2502 -> [w2521 _]
          tunnel: w2503 -> [w2522 _]
          tunnel: w2501 -> [w2526 _]
          tunnel: w2507 -> [w2525 _]
          tunnel: w2491 -> [w2519 _]
          tunnel: w2492 -> [_ w2537]
          frame False {
            # "EXCHANGE PERMISSION"
            n981 = Bundle By Name(cluster=w2523, "name"=w2522, "permission"=w2519, "password"=w2521) -> (w2520:T20)
            n982 = Replace Array Subset(array=w2526, new element=w2520, index=w2525) -> (w2524:T4)
            n983 = local write "user list"(w2524) -> ()
          }
          frame True {
            # "INVALID ENTRY"
            n984 = local read "language"() -> (w2529:enum32{"PT", "EN", "NONE"})
            n985 = Not Equal?(x=w2529, y=enum32{"PT", "EN", "NONE"}."EN" ("language")) -> (x != y?=w2528:bool)
            n986 = Select(t="Você não pode mudar\nsua própria permissão. " ("message"), s=w2528, f="You can't exchange \nyour own permission. " ("message")) -> (s? t:f=w2532:string)
            n987 = Select(t="A permissão Admin é\nlimitada a 2 usuários." ("message"), s=w2528, f="Admin permission\nlimited to only 2 users." ("message")) -> (s? t:f=w2531:string)
            n988 = Select(t=w2532, s=w2537, f=w2531) -> (s? t:f=w2530:string)
            n989 = One Button Dialog(message=w2530) -> ()  [unwired: 1 in, 1 out]
          }
        }
      }
      event "user insert": Value Change {
        # "Check\nconfig \nuser qty."
        # "Check for empty name"
        # "Check for equal names"
        n990 = event-data() -> ()  [unwired: 1 in, 6 out]
        n991 = local read "user list"() -> (w2539:T4)
        n992 = for {
          tunnel: w2539 -> [w2562] mode=indexing
          tunnel: [w2565] -> w2553
          tunnel: "user name" -> [w2563]
          tunnel: [w2562] -> w2552
          stop <- w2565 stop-if-true
          n993 = Unbundle By Name(w2562) -> ("name"=w2564:string)
          n994 = Equal?(x=w2563, y=w2564) -> (x = y?=w2565:bool)
        }
        n995 = for {
          tunnel: w2539 -> [w2561] mode=indexing
          shift-right: [w2560] -> w2548
          shift-left: u32 0 ("x") -> [w2558]
          n996 = Unbundle By Name(w2561) -> ("permission"=w2556:string)
          n997 = Equal?(x="Admin", y=w2556) -> (x = y?=w2559:bool)
          n998 = Increment(x=w2558) -> (x+1=w2557:u32)
          n999 = Select(t=w2557, s=w2559, f=w2558) -> (s? t:f=w2560:u32)
        }
        n1000 = Empty String/Path?(string/path="user name") -> (empty?=w2554:bool)
        n1001 = Or(x=w2554, y=w2553) -> (x .or. y?=w2544:bool)
        n1002 = Greater?(x=w2548, y=u32 1) -> (0:w2538:bool)
        n1003 = Equal?(x="user permission", y="Admin") -> (x = y?=w2545:bool)
        n1004 = And(x=w2545, y=w2538) -> (x .and. y?=w2543:bool)
        n1005 = Or(x=w2543, y=w2544) -> (x .or. y?=w2542:bool)
        n1006 = case shown="True" w2542 {
          tunnel: w2539 -> [w2575 _]
          tunnel: w2552 -> [w2574 _]
          tunnel: "user name" -> [w2573 _]
          tunnel: "user permission" -> [w2569 _]
          tunnel: w2538 -> [_ w2585]
          frame False {
            w2567 = ""
            # "INSERT USER INTO USER LIST"
            n1007 = Array Size(array=w2575) -> (size(s)=w2571:i32)
            n1008 = Bundle By Name(cluster=w2574, "name"=w2573, "permission"=w2569, "password"=w2567) -> (w2572:T20)
            n1009 = local write "user name"(w2567) -> ()
            n1010 = Build Array(w2571) -> (w2570:i32[])
            n1011 = property on="user list" class="Arr (strict)"("Index Values"=w2570) -> ()  [unwired: 2 in, 2 out]
            n1012 = Insert Into Array(array=w2575, new element=w2572) -> (w2566:T4)  [unwired: 1 in]
            n1013 = property on="user name" class="Str"("Key Focus"=TRUE) -> ()  [unwired: 2 in, 2 out]
            n1014 = local write "user list"(w2566) -> ()
          }
          frame True {
            # "INVALID USER NAME"
            n1015 = local read "language"() -> (w2584:enum32{"PT", "EN", "NONE"})
            n1016 = Not Equal?(x=w2584, y=enum32{"PT", "EN", "NONE"}."EN" ("language")) -> (x != y?=w2583:bool)
            n1017 = Select(t="A permissão Admin é\nlimitada a 2 usuários." ("message"), s=w2583, f="Admin permission\nlimited to only 2 users." ("message")) -> (s? t:f=w2578:string)
            n1018 = Select(t="Nome de usuário inválido" ("message"), s=w2583, f="Invalid user name." ("message")) -> (s? t:f=w2577:string)
            n1019 = Select(t=w2578, s=w2585, f=w2577) -> (s? t:f=w2586:string)
            n1020 = One Button Dialog(message=w2586) -> ()  [unwired: 1 in, 1 out]
          }
        }
      }
      event "check email": Value Change {
        n1021 = event-data() -> ()  [unwired: 1 in, 6 out]
        n1022 = local read "language"() -> (w2602:enum32{"PT", "EN", "NONE"})
        n1023 = property on="email ok" class="Bool (strict)"(error in=w2591, "DisabledEnum"=T12."Enabled" ("Disabled")) -> (error out=w2605:errorcluster)  [unwired: 1 in, 1 out]
        n1024 = Not Equal?(x=w2602, y=enum32{"PT", "EN", "NONE"}."EN" ("language")) -> (x != y?=w2601:bool)
        n1025 = call "Get attributes.vi"("error in (no error)"=w2591, "ICS in"=w2594) -> ("error out"=w2593:errorcluster, "email settings"=w2590:T10, "ICS out"=w2592:refnum<class "ICS.lvclass">)  [unwired: 6 in, 1 out]
        n1026 = Bundle By Name(cluster=w2590, "email enabled"=TRUE) -> (w2589:T10)
        n1027 = property on="email ok" class="Bool (strict)"(error in=w2605, "Blinking"=TRUE) -> (error out=w2587:errorcluster)  [unwired: 1 in, 1 out]
        n1028 = Select(t="O S4ICS está testando o e-mail.\nPor favor, não responda a\nesta menssagem.\n" ("menssagem:"), s=w2601, f="S4ICS is testing the email service.\nPlease do not reply to this message.\n" ("menssagem:")) -> (s? t:f=w2596:string)
        n1029 = call "Send email.vi"("error in (no error)"=w2587, "message"=w2596, "email settings"=w2589) -> ("error out"=w2595:errorcluster, "fail"=w2597:bool)  [unwired: 7 in]
        n1030 = Not(x=w2597) -> (.not. x?=→"email ok":bool)
        n1031 = property on="email ok" class="Bool (strict)"(error in=w2595, "Blinking"=FALSE) -> ()  [unwired: 1 in, 2 out]
      }
      event "pwrPM mains": Value Change {
        n1032 = event-data() -> ()  [unwired: 1 in, 6 out]
        n1033 = Select(t=T12."Disabled and Grayed Out" ("Disabled"), s="pwrPM mains", f=T12."Enabled" ("Disabled")) -> (s? t:f=w2611:T12)
        n1034 = property on="pwrPM ip" class="Str"("DisabledEnum"=w2611) -> ()  [unwired: 2 in, 2 out]
        n1035 = property on="pwrPM port" class="DigNum (strict)"("DisabledEnum"=w2611) -> ()  [unwired: 2 in, 2 out]
        n1036 = property on="pwrPM user" class="Str"("DisabledEnum"=w2611) -> ()  [unwired: 2 in, 2 out]
        n1037 = property on="pwrPM password" class="Str"("DisabledEnum"=w2611) -> ()  [unwired: 2 in, 2 out]
        n1038 = property on="pwrPM outlet" class="DigNum (strict)"("DisabledEnum"=w2611) -> ()  [unwired: 2 in, 2 out]
      }
      event "pwrGD mains": Value Change {
        n1039 = event-data() -> ()  [unwired: 1 in, 6 out]
        n1040 = Select(t=T12."Disabled and Grayed Out" ("Disabled"), s="pwrGD mains", f=T12."Enabled" ("Disabled")) -> (s? t:f=w2617:T12)
        n1041 = property on="pwrGD ip" class="Str"("DisabledEnum"=w2617) -> ()  [unwired: 2 in, 2 out]
        n1042 = property on="pwrGD port" class="DigNum (strict)"("DisabledEnum"=w2617) -> ()  [unwired: 2 in, 2 out]
        n1043 = property on="pwrGD user" class="Str"("DisabledEnum"=w2617) -> ()  [unwired: 2 in, 2 out]
        n1044 = property on="pwrGD password" class="Str"("DisabledEnum"=w2617) -> ()  [unwired: 2 in, 2 out]
        n1045 = property on="pwrGD outlet" class="DigNum (strict)"("DisabledEnum"=w2617) -> ()  [unwired: 2 in, 2 out]
      }
      event "return setup": Value Change {
        # "RECOVER THE LAST CONFIGURATION FROM DATALOG FILE TO CANCEL ALL CHANGES."
        n1046 = event-data() -> ()  [unwired: 1 in, 6 out]
        n1047 = call "Get attributes.vi"("error in (no error)"=w2626, "ICS in"=w2638) -> ("error out"=w2629:errorcluster, "email settings"=w2624:T10, "control indices"=w2628:i32[], "ICS out"=w2631:refnum<class "ICS.lvclass">)  [unwired: 6 in]
        n1048 = local read "cfgFile"() -> (w2633:string)
        n1049 = call <vilib>:"Application Directory.vi"() -> ("Application Directory"=w2634:path)
        n1050 = Build Array(u32 0) -> (w2636:u32[])
        n1051 = Get Control Values by Index(1:w2628, 3:w2629) -> (10:w2627:variant[], 11:w2625:errorcluster)  [unwired: 1 in]
        n1052 = Build Path(base path=w2634, name or relative path=w2633) -> (appended path=w2630:path)
        n1053 = local write "tab menu"(T6."Stopped" ("tab menu")) -> ()
        n1054 = local write "tab body"(enum32{"Motors", "Config"}."Motors" ("tab body")) -> ()
        n1055 = property on="user list" class="Arr (strict)"("Index Values"=w2636) -> ()  [unwired: 2 in, 2 out]
        n1056 = call "Config file.vi"("path"=w2630, "access (0:read/write)"=enum16{"read/write", "read-only", "write-only"}."read-only", "error in (no error)"=w2625, "data values"=w2627, "email settings"=w2624) -> ("error out"=w2623:errorcluster, "data out"=w2622:variant[])  [unwired: 5 in]
        n1057 = Set Control Values by Index(1:w2628, 2:w2622, 3:w2623) -> (11:w2632:errorcluster)  [unwired: 1 in]
      }
      event "control": Value Change {
        w2641 = T12."Disabled and Grayed Out" ("Disabled")
        # "TEMPORARY. THE\nGOTO SUBROUTINES OF ALL MOTORS MUST\nBE STORED INTO MOTOR MEMORY IN ORDER TO ENABLE THE JUMP FUNCTION."
        n1058 = event-data() -> ()  [unwired: 1 in, 6 out]
        n1059 = local write "tab menu"(T6."Control" ("tab menu")) -> ()
        n1060 = local write "tab body"(enum32{"Motors", "Config"}."Motors" ("tab body")) -> ()
        n1061 = local read "WPROT disabled"() -> (w2648:bool)
        n1062 = local read "WPSEL disabled"() -> (w2649:bool)
        n1063 = local read "CALW disabled"() -> (w2647:bool)
        n1064 = local read "GMIR disabled"() -> (w2646:bool)
        n1065 = local read "ASEL disabled"() -> (w2650:bool)
        n1066 = property on="control motor sel" class="RadioBtnsControl (strict)"("Value"=T7."No Selection" ("control motor sel")) -> ()  [unwired: 2 in, 2 out]
        n1067 = property on="control motor sel" class="RadioBtnsControl (strict)"() -> ("Controls[]"=w2645:refnum<vi>[])  [unwired: 2 in, 2 out]
        n1068 = Build Array(w2648, w2649, w2650, w2647, w2646, w2646) -> (w2644:bool[])
        n1069 = for {
          tunnel: w2645 -> [w2656] mode=indexing
          tunnel: w2644 -> [w2658] mode=indexing
          tunnel: T12."Disabled" ("Disabled") -> [w2655]
          tunnel: T12."Enabled" ("Disabled") -> [w2654]
          # "APPLY CONFIG.\nDISABLE CONTROLS TO MOTOR SELECTOR"
          n1070 = Select(t=w2655, s=w2658, f=w2654) -> (s? t:f=w2657:T12)
          n1071 = property class="Ctl"(reference=w2656, "DisabledEnum"=w2657) -> ()  [unwired: 1 in, 2 out]
        }
        n1072 = property on="control send" class="Bool"("DisabledEnum"=w2641) -> ()  [unwired: 2 in, 2 out]
        n1073 = property on="control jump" class="Bool"("DisabledEnum"=w2641) -> ()  [unwired: 2 in, 2 out]
        n1074 = property on="control jump" class="Bool"("DisabledEnum"=w2641) -> ()  [unwired: 2 in, 2 out]
        n1075 = property on="control position" class="DigNum (strict)"("DisabledEnum"=w2641) -> ()  [unwired: 2 in, 2 out]
      }
      event "control motor sel": Value Change {
        n1076 = event-data() -> ()  [unwired: 1 in, 6 out]
        n1077 = Equal?(x="control motor sel", y=T7."No Selection" ("control motor sel")) -> (x = y?=w2665:bool)
        n1078 = case shown="\"No Selection\", Default" "control motor sel" {
          tunnel: [w2670 w2671 w2672 w2673 w2674 w2675 ""] -> w2660
          frame "control WPROT" {
            # "GET MOTOR IP"
            n1079 = local read "WPROT ip"() -> (w2670:string)
          }
          frame "control WPSEL" {
            # "GET MOTOR IP"
            n1080 = local read "WPSEL ip"() -> (w2671:string)
          }
          frame "control ASEL" {
            # "GET MOTOR IP"
            n1081 = local read "ASEL ip"() -> (w2672:string)
          }
          frame "control CALW" {
            # "GET MOTOR IP"
            n1082 = local read "CALW ip"() -> (w2673:string)
          }
          frame "control GFOC" {
            # "GET MOTOR IP"
            n1083 = local read "GMIR ip"() -> (w2674:string)
          }
          frame "control GMIR" {
            # "GET MOTOR IP"
            n1084 = local read "GMIR ip"() -> (w2675:string)
          }
          frame "No Selection", Default {
            # "GET MOTOR IP"
          }
        }
        n1085 = Select(t=T12."Disabled and Grayed Out" ("Disabled"), s=w2665, f=T12."Enabled" ("Disabled")) -> (s? t:f=w2667:T12)
        n1086 = call "Write motor IP.vi"("error in (no error)"=w2663, "motor IP"=w2660, "ICS in"=w2664) -> ("error out"=w2662:errorcluster, "ICS out"=w2661:refnum<class "ICS.lvclass">)  [unwired: 7 in]
        n1087 = property on="control jump" class="Bool"("DisabledEnum"=w2667) -> ()  [unwired: 2 in, 2 out]
        n1088 = property on="control send" class="Bool"("DisabledEnum"=w2667) -> ()  [unwired: 2 in, 2 out]
      }
      event "control send": Value Change {
        n1089 = event-data() -> ()  [unwired: 1 in, 6 out]
        n1090 = call-dynamic "Read motor IP.vi"("error in (no error)"=w2682, "ICS in"=w2681) -> ("error out"=w2680:errorcluster, "motor IP"=w2677:string, "ICS out"=w2679:refnum<class "ICS.lvclass">)  [unwired: 7 in]
        n1091 = Empty String/Path?(string/path="control instruction") -> (empty?=w2683:bool)
        n1092 = Empty String/Path?(string/path=w2677) -> (empty?=w2678:bool)
        n1093 = Or(x=w2683, y=w2678) -> (x .or. y?=w2684:bool)
        n1094 = case shown="False" w2684 {
          tunnel: w2680 -> [w2702 w2708]
          tunnel: "control instruction" -> [w2701 _]
          tunnel: [w2688 w2708] -> w2685
          tunnel: w2677 -> [w2687 _]
          frame False {
            # "SEND INSTRUCTION AND WAITS FOR MOTOR RESPONSE"
            n1095 = call "Send batch.vi"("error in (no error)"=w2702, "motor ip"=w2687, "instruction"=w2701) -> ("error out"=w2699:errorcluster, "ok"=w2693:bool, "response"=→"control response":string)  [unwired: 4 in, 2 out]
            n1096 = call <vilib>:"Space Constant.vi"() -> ("String"=w2700:string)
            n1097 = Search and Replace String(replace all?=TRUE ("replace all? (F)"), input string=w2701, search string=w2700, error in=w2699) -> (result string=w2697:string, error out=w2688:errorcluster)  [unwired: 4 in, 2 out]
            n1098 = Match Pattern(string=w2697, regular expression="EO=") -> (after substring=w2692:string, offset past match=w2695:i32)  [unwired: 1 in, 2 out]
            n1099 = Equal?(x="1" ("regular expression"), y=w2692) -> (x = y?=w2689:bool)
            n1100 = Greater Or Equal To 0?(x=w2695) -> (x >= 0?=w2694:bool)
            n1101 = And(x=w2693, y=w2694) -> (x .and. y?=w2690:bool)
            n1102 = case shown="True" w2690 {
              tunnel: w2689 -> [_ w2707]
              frame False {
              }
              frame True {
                # "DIS/ENABLE ACCORDING TO MOTOR EO (ENABLE OUTPUT)"
                n1103 = Select(t=T12."Disabled and Grayed Out" ("Disabled"), s=w2707, f=T12."Enabled" ("Disabled")) -> (s? t:f=w2704:T12)
                n1104 = property on="return control" class="Bool"("DisabledEnum"=w2704) -> ()  [unwired: 2 in, 2 out]
                n1105 = property on="control motor sel" class="RadioBtnsControl (strict)"("DisabledEnum"=w2704) -> ()  [unwired: 2 in, 2 out]
              }
            }
          }
          frame True {
            # "NO COMMAND, DO NOTHING"
          }
        }
      }
      event "control jump": Value Change {
        # "MECH.   RANGE    UNIT    DMX-ETH\nWPROT  0 - 360  degree  0 - 36000\nWPSEL  0 - 100     %    0 - 10000\nASEL   0 - 100     %    0 - 10000\nCALW   0 - 360  degree  0 - 36000\nGMIR   0 - 360  degree  0 - 36000\nGFOC   0 - 20     mm    0 - 20000"
        n1106 = event-data() -> ()  [unwired: 1 in, 6 out]
        n1107 = local read "control motor sel"() -> (w2713:T7)
        n1108 = Equal?(x=T7."No Selection" ("control motor sel"), y=w2713) -> (x = y?=w2712:bool)
        n1109 = case shown="False" w2712 {
          tunnel: w2713 -> [w2730 _]
          tunnel: w2711 -> [w2729 w2757]
          tunnel: [w2727 w2757] -> w2710
          frame False {
            # "CALL GOTO SUBROUTINE"
            n1110 = case shown="\"No Selection\", Default" w2730 {
              tunnel: [w2739 w2742 w2745 w2748 w2751 w2754 w2755] -> w2718
              tunnel: [100.0 ("y") 100.0 ("y") 100.0 ("y") 100.0 ("y") 100.0 ("y") 1000.0 ("y") 0.0 ("y")] -> w2725
              tunnel: ["GOSUB 12" "GOSUB 13" "GOSUB 14" "GOSUB 15" "GOSUB 16" "GOSUB 17" w2755] -> w2717
              frame "control WPROT" {
                # "MOTOR INDEX"
                n1111 = local read "WPROT ip"() -> (w2739:string)
              }
              frame "control WPSEL" {
                # "MOTOR INDEX"
                n1112 = local read "WPSEL ip"() -> (w2742:string)
              }
              frame "control ASEL" {
                # "MOTOR INDEX"
                n1113 = local read "ASEL ip"() -> (w2745:string)
              }
              frame "control CALW" {
                # "MOTOR INDEX"
                n1114 = local read "CALW ip"() -> (w2748:string)
              }
              frame "control GFOC" {
                # "MOTOR INDEX"
                n1115 = local read "GMIR ip"() -> (w2751:string)
              }
              frame "control GMIR" {
                # "MOTOR INDEX"
                n1116 = local read "GMIR ip"() -> (w2754:string)
              }
              frame "No Selection", Default {
                w2755 = ""
                # "MOTOR INDEX"
              }
            }
            n1117 = Multiply(x="control position", y=w2725) -> (x*y=w2724:dbl)
            n1118 = To Long Integer(number=w2724) -> (32bit integer=w2722:i32)
            n1119 = Number To Decimal String(number=w2722) -> (decimal integer string=w2721:string)  [unwired: 1 in]
            n1120 = Concatenate Strings(w2721, "V12=") -> (w2720:string)
            n1121 = call "Send instruction.vi"("error in (no error)"=w2729, "motor ip"=w2718, "instruction"=w2720) -> ("error out"=w2728:errorcluster, "response"=w2719:string)  [unwired: 5 in, 2 out]
            n1122 = flat-sequence {
              tunnel: w2720 -> [w2736]
              tunnel: w2719 -> [w2735]
              tunnel: [w2733] -> w2715
              frame #0 {
                n1123 = local write "control instruction"(w2736) -> ()
                n1124 = local write "control response"(w2735) -> ()
                n1125 = Wait (ms)(milliseconds to wait=u32 250) -> (millisecond timer value=w2733:u32)
              }
            }
            n1126 = call "Send instruction.vi"("error in (no error)"=w2728, "motor ip"=w2718, "instruction"=w2717) -> ("error out"=w2727:errorcluster, "response"=w2716:string)  [unwired: 5 in, 2 out]
            n1127 = flat-sequence {
              tunnel: w2717 -> [w2732]
              tunnel: w2716 -> [w2731]
              tunnel: w2715 -> [_]
              frame #0 {
                n1128 = local write "control instruction"(w2732) -> ()
                n1129 = local write "control response"(w2731) -> ()
              }
            }
          }
          frame True {
            # "NO COMMAND, DO NOTHING"
          }
        }
      }
      event "control stop": Value Change {
        n1130 = event-data() -> ()  [unwired: 1 in, 6 out]
        n1131 = local read "control motor sel"() -> (w2762:T7)
        n1132 = Equal?(x=T7."No Selection" ("control motor sel"), y=w2762) -> (x = y?=w2761:bool)
        n1133 = case shown="False" w2761 {
          tunnel: w2762 -> [w2769 _]
          tunnel: w2760 -> [w2768 w2779]
          tunnel: [w2766 w2779] -> w2759
          frame False {
            w2764 = "STOPX" ("regular expression")
            # "SEND STOP INSTRUCTION"
            n1134 = case shown="\"No Selection\", Default" w2769 {
              tunnel: [w2772 w2773 w2774 w2775 w2776 w2777 ""] -> w2767
              frame "control WPROT" {
                # "MOTOR INDEX"
                n1135 = local read "WPROT ip"() -> (w2772:string)
              }
              frame "control WPSEL" {
                # "MOTOR INDEX"
                n1136 = local read "WPSEL ip"() -> (w2773:string)
              }
              frame "control ASEL" {
                # "MOTOR INDEX"
                n1137 = local read "ASEL ip"() -> (w2774:string)
              }
              frame "control CALW" {
                # "MOTOR INDEX"
                n1138 = local read "CALW ip"() -> (w2775:string)
              }
              frame "control GFOC" {
                # "MOTOR INDEX"
                n1139 = local read "GMIR ip"() -> (w2776:string)
              }
              frame "control GMIR" {
                # "MOTOR INDEX"
                n1140 = local read "GMIR ip"() -> (w2777:string)
              }
              frame "No Selection", Default {
                # "MOTOR INDEX"
              }
            }
            n1141 = call "Send instruction.vi"("error in (no error)"=w2768, "motor ip"=w2767, "instruction"=w2764) -> ("error out"=w2766:errorcluster, "response"=w2765:string)  [unwired: 5 in, 2 out]
            n1142 = flat-sequence {
              tunnel: w2764 -> [w2771]
              tunnel: w2765 -> [w2770]
              frame #0 {
                n1143 = local write "control instruction"(w2771) -> ()
                n1144 = local write "control response"(w2770) -> ()
              }
            }
          }
          frame True {
            # "NO COMMAND, DO NOTHING"
          }
        }
      }
      event "return control": Value Change {
        w2782 = ""
        n1145 = event-data() -> ()  [unwired: 1 in, 6 out]
        n1146 = call "Write motor IP.vi"("error in (no error)"=w2787, "motor IP"="", "ICS in"=w2786) -> ("error out"=w2784:errorcluster, "ICS out"=w2785:refnum<class "ICS.lvclass">)  [unwired: 7 in]
        n1147 = local write "tab menu"(T6."Stopped" ("tab menu")) -> ()
        n1148 = local write "tab body"(enum32{"Motors", "Config"}."Motors" ("tab body")) -> ()
        n1149 = local write "control motor sel"(T7."No Selection" ("control motor sel")) -> ()
        n1150 = local write "control response"(w2782) -> ()
        n1151 = local write "control instruction"(w2782) -> ()
      }
    }
    n1152 = call-dynamic "Publish 0mq.vi"("error in (no error)"=w260, "ICS in"=w261) -> ("error out"=w259:errorcluster, "ICS out"=w258:refnum<class "ICS.lvclass">)  [unwired: 8 in]
    n1153 = case shown="True" "animation" {
      tunnel: w258 -> [w274 w280]
      tunnel: [w274 w277] -> w267
      tunnel: [w273 w276] -> w266
      tunnel: w259 -> [w273 w275]
      frame False {
      }
      frame True {
        n1154 = call-dynamic "Read motors.vi"("error in (no error)"=w275, "ICS in"=w280) -> ("error out"=w276:errorcluster, "motors"=w279:refnum<class "Motor.lvclass">[], "ICS out"=w277:refnum<class "ICS.lvclass">)  [unwired: 7 in]
        n1155 = for {
          tunnel: w279 -> [w285] mode=indexing
          tunnel: w276 -> [w286]
          shift-right: [w284] -> _
          shift-left: FALSE -> [w283]
          n1156 = call-dynamic "Get name and position.vi"("error in (no error)"=w286, "Motor in"=w285) -> ("position"=w281:dbl, "name"=w282:string)  [unwired: 6 in, 2 out]
          n1157 = case shown="\"WPSEL\", Default" w282 {
            tunnel: w281 -> [w301 w317 w330 w369 w381 w397]
            tunnel: [w300 w316 w329 w368 w382 w396] -> w284
            tunnel: w283 -> [w300 w316 w329 w368 w382 _]
            frame "WPSEL", Default {
              w287 = 160.0 ("RANGE")
              # "MAX"
              # "X0"
              # "RANGE"
              n1158 = Equal To 0?(x=w301) -> (x = 0?=w297:bool)
              "wpsel lim/2" <- w297
              n1159 = Equal?(x=w287, y=w301) -> (x = y?=w298:bool)
              "wpsel lim/4" <- w298
              n1160 = Multiply(x=182.0 ("RANGE"), y=w301) -> (x*y=w295:dbl)
              n1161 = Divide(x=w295, y=w287) -> (x/y=w294:dbl)
              n1162 = Or(x=w297, y=w298) -> (x .or. y?=w299:bool)
              n1163 = In Range and Coerce(upper limit=80.5 ("RANGE"), x=w301, lower limit=79.5 ("RANGE")) -> (In Range?=w288:bool)  [unwired: 1 out]
              n1164 = Or(x=w300, y=w288) -> (x .or. y?=→"wp home":bool)
              n1165 = property on="wprot ctl" class="Knob (strict)"("Visible"=w299) -> ()  [unwired: 2 in, 2 out]
              n1166 = Add(x=113.0 ("OFFSET"), y=w294) -> (x+y=w296:dbl)
              n1167 = property on="wpsel anime" class="Pict"("Left"=w296) -> ()  [unwired: 2 in, 2 out]
              "WPSEL Value" <- w301
            }
            frame "ASEL" {
              (unwired) 100.0 ("y")
              (unwired) 100.0 ("ASEL position")
              # "MAX"
              n1168 = local read "asel image"() -> (w315:T2)
              n1169 = Divide(x=-30.0 ("ASEL position"), y=30.0 ("ASEL position")) -> (x/y=w312:dbl)
              n1170 = Multiply(x=w312, y=w317) -> (x*y=w311:dbl)
              n1171 = Less Or Equal To 0?(x=w317) -> (x <= 0?=→"asel lim off":bool)
              n1172 = Greater Or Equal?(x=w317, y=28.0) -> (x >= y?=→"asel lim on":bool)
              n1173 = call "Picture Rotation.vi"("transparent?"=TRUE, "theta (deg)"=w311, "image data in"=w315) -> ("image data out"=w310:T2)  [unwired: 7 in, 1 out]
              n1174 = call <vilib>:"Get Image Subset.vi"("subset rect"=T14 {"left"=276, "top"=25, "right"=700, "bottom"=480}, "image data"=w310) -> ("image subset"=w308:T2)  [unwired: 4 in, 1 out]
              n1175 = call <vilib>:"Draw Flattened Pixmap.vi"("image data"=w308, "picture"=picture data[5B]) -> ("new picture"=→"asel anime":picture)  [unwired: 7 in]
              "ASEL Value" <- w317
            }
            frame "CALW" {
              n1176 = Absolute Value(x=w330) -> (abs(x)=w323:dbl)
              n1177 = Quotient & Remainder(x=w323, y=360.0) -> (x-y*floor(x/y)=w328:dbl)  [unwired: 1 out]
              n1178 = Cluster To Array(cluster=cluster{dbl, dbl, dbl, dbl, dbl} {0.0, 72.0, 144.0, 216.0, 288.0} ("Knob")) -> (array=w321:dbl[])
              n1179 = for {
                tunnel: w321 -> [w353] mode=indexing
                tunnel: [w355] -> w320 mode=indexing
                tunnel: w328 -> [w351]
                # "OFFSET"
                n1180 = Subtract(x=360.0 ("y"), y=w353) -> (x-y=w352:dbl)
                n1181 = Add(x=w351, y=10.0) -> (x+y=w350:dbl)
                n1182 = Subtract(x=w350, y=w352) -> (x-y=w356:dbl)
                n1183 = Add(x=w353, y=w350) -> (x+y=w357:dbl)
                n1184 = Greater Or Equal?(x=w357, y=360.0) -> (x >= y?=w358:bool)
                n1185 = Select(t=w356, s=w358, f=w357) -> (s? t:f=w355:dbl)
              }
              n1186 = To Word Integer(number=w328) -> (16bit integer=w324:i16)
              n1187 = Array To Cluster(array=w320) -> (cluster=w322:T21)
              n1188 = case shown="-1, Default" w324 {
                tunnel: [TRUE FALSE TRUE FALSE TRUE FALSE] -> w325
                tunnel: [FALSE FALSE FALSE TRUE TRUE FALSE] -> w326
                tunnel: [FALSE TRUE TRUE FALSE FALSE FALSE] -> w327
                frame 0 {
                }
                frame 72 {
                }
                frame 144 {
                }
                frame 216 {
                }
                frame 288 {
                }
                frame -1, Default {
                }
              }
              "calw0" <- w325
              "calw1" <- w327
              "calw2" <- w326
              n1189 = local write "calw knob"(w322) -> ()
              "CALW Value" <- w330
            }
            frame "GFOC" {
              w360 = 25.0 ("x")
              # "MAX"
              # "X0"
              # "RANGE"
              n1190 = Multiply(x=22.0, y=w369) -> (x*y=w364:dbl)
              n1191 = Equal To 0?(x=w369) -> (x = 0?=→"GFOC home":bool)
              n1192 = Equal?(x=w360, y=w369) -> (x = y?=→"GFOC limit":bool)
              n1193 = Divide(x=w364, y=w360) -> (x/y=w365:dbl)
              n1194 = Add(x=73.0, y=w365) -> (x+y=w363:dbl)
              n1195 = property on="guider cam anime" class="Pict"("Left"=w363) -> ()  [unwired: 2 in, 2 out]
              "GFOC Value" <- w369
            }
            frame "GMIR" {
              n1196 = Absolute Value(x=w381) -> (abs(x)=w375:dbl)
              n1197 = Quotient & Remainder(x=w375, y=360.0) -> (x-y*floor(x/y)=w374:dbl)  [unwired: 1 out]
              n1198 = Subtract(x=w374, y=0.0) -> (x-y=w379:dbl)
              n1199 = Add(x=0.0, y=w374) -> (x+y=w378:dbl)
              n1200 = Equal To 0?(x=w374) -> (x = 0?=→"GMIR home":bool)
              n1201 = Greater Or Equal?(x=w378, y=360.0) -> (x >= y?=w377:bool)
              n1202 = Select(t=w379, s=w377, f=w378) -> (s? t:f=→"gmir knob":dbl)
              "GMIR Value" <- w381
            }
            frame "WPROT" {
              n1203 = Absolute Value(x=w397) -> (abs(x)=w391:dbl)
              n1204 = Quotient & Remainder(x=w391, y=360.0) -> (x-y*floor(x/y)=w385:dbl)  [unwired: 1 out]
              n1205 = Subtract(x=w385, y=0.0) -> (x-y=w394:dbl)
              n1206 = Add(x=0.0, y=w385) -> (x+y=w393:dbl)
              n1207 = Greater Or Equal?(x=w393, y=360.0) -> (x >= y?=w392:bool)
              n1208 = property on="wprot ctl" class="Knob (strict)"() -> ("Visible"=w383:bool)  [unwired: 2 in, 2 out]
              n1209 = Less Or Equal?(x=w385, y=0.5) -> (x <= y?=w384:bool)
              n1210 = Select(t=w394, s=w392, f=w393) -> (s? t:f=→"wprot ctl":dbl)
              n1211 = And(x=w383, y=w384) -> (x .and. y?=w396:bool)
              "WPROT Value" <- w397
            }
          }
        }
      }
    }
    n1212 = flat-sequence {
      frame #0 {
        # "ANIMAÇÃO DO PAINEL: 100ms"
      }
    }
  }
  n1213 = Bundle By Name(cluster=T8 {"S4commandQueueName"="", "S4statusQueueName"="", "comm configuration"={"channel"=enum."Local Panel", "address"="", "port"=0, "timeout"=0}} ("intercomm configuration"), "S4commandQueueName"="S4command", "S4statusQueueName"="S4status", "comm configuration.address"=w1, "comm configuration.timeout"="pubTime0mq") -> (w6:T8)
  n1214 = while {
    tunnel: w6 -> [w2790]
    tunnel: [w2789] -> w8
    stop <- w2789 stop-if-true
    # "THE 0MQ COMM  STOPS RUNNING WHEN A EXIT MESSAGE IS READ FROM THE QUEUE BUT DOES NOT DESTROY THE QUEUES."
    # "RUNS THE ZEROMQ COMM"
    n1215 = disable-structure shown="Enabled" {
      disable-tunnel: w2790 -> [w2792 w2793]
      disable-tunnel: [w2791 w2794] -> w2789
      frame Disabled {
        n1216 = call "0mqManager.vi"("intercomm configuration"=w2792) -> ("exit"=w2791:bool)  [unwired: 9 in, 1 out]
      }
      frame Enabled {
        # "20240731"
        n1217 = call "0mqPubRep.vi"("intercomm configuration"=w2793) -> ("exit"=w2794:bool)  [unwired: 9 in, 1 out]
      }
    }
  }
  n1218 = flat-sequence {
    tunnel: w10 -> [w2806]
    tunnel: w30 -> [w2807]
    tunnel: w8 -> [_]
    frame #0 {
      w2812 = ""
      # "20240718"
      # "20240621"
      n1219 = call-dynamic "Read Messenger.vi"("error in (no error)"=w2806, "ICS in"=w2807) -> ("error out"=w2803:errorcluster, "Messenger.lvclass"=w2804:refnum<class "Messenger.lvclass">, "ICS out"=w2805:refnum<class "ICS.lvclass">)  [unwired: 7 in]
      n1220 = local read "enabled log"() -> (w2798:string)
      n1221 = disable-structure shown="Enabled" {
        disable-tunnel: w2804 -> [w2819 w2824]
        disable-tunnel: w2803 -> [w2818 w2821]
        disable-tunnel: [w2817 w2825] -> w2800
        disable-tunnel: T18 {"Message"="exit", "Message Data"=variant} ("message") -> [_ w2820]
        frame Disabled {
          n1222 = call-dynamic "Stop 0mqComm.vi"("error in (no error)"=w2818, "Messenger in"=w2819) -> ("error out"=w2817:errorcluster)  [unwired: 8 in, 1 out]
        }
        frame Enabled {
          # "20240716"
          # "20240619"
          n1223 = call-dynamic "Send message.vi"("error in (no error)"=w2821, "message"=w2820, "Messenger in"=w2824) -> ("error out"=w2822:errorcluster, "Messenger out"=w2823:refnum<class "Messenger.lvclass">)  [unwired: 7 in]
          n1224 = call-dynamic "Destroy queues.vi"("error in (no error)"=w2822, "Messenger in"=w2823) -> ("error out"=w2825:errorcluster)  [unwired: 8 in, 1 out]
        }
      }
      n1225 = local read "version"() -> (w2797:string)
      n1226 = call "Read Server.vi"("error in (no error)"=w2803, "ICS in"=w2805) -> ("error out"=w2813:errorcluster, "Server"=w2815:refnum<class "TCP-Server.lvclass">)  [unwired: 7 in, 1 out]
      n1227 = call "Read listenner.vi"("error in (no error)"=w2813, "Server in"=w2815) -> ("error out"=w2814:errorcluster, "listenner ID"=w2816:refnum<k5>)  [unwired: 7 in, 1 out]
      n1228 = TCP Close Connection(connection ID=w2816, error in (no error)=w2814) -> (error out=w2801:errorcluster)  [unwired: 1 in, 1 out]
      n1229 = call "Write log to file.vi"("prefix"="EXIT" ("current priority"), "version"=w2797, "current priority"="6", "enabled priority"=w2798) -> ()  [unwired: 5 in, 3 out]
      n1230 = Merge Errors(w2801, w2800) -> (w2802:errorcluster)
      n1231 = property class="App"() -> ("App.Kind"=w2811:T22)  [unwired: 2 in, 2 out]
      n1232 = call <vilib>:"Clear Errors.vi"("error in (no error)"=w2802) -> ("error out"=w2810:errorcluster)  [unwired: 5 in, 1 out]
      n1233 = case shown="\"Run Time System\"" w2811 {
        tunnel: w2810 -> [_ _]
        frame "Development System", Default {
        }
        frame "Run Time System" {
          n1234 = Quit LabVIEW(quit? (T)=TRUE) -> ()
        }
      }
      n1235 = local write "tab menu"(T6."Login" ("tab menu")) -> ()
      n1236 = local write "tab body"(enum32{"Motors", "Config"}."Motors" ("tab body")) -> ()
      n1237 = local write "loginUser"(w2812) -> ()
      n1238 = local write "loginPW"(w2812) -> ()
    }
  }
  "version" <- "20240924" ("version")
